vi "磨合台.vi"() -> ()   [LabVIEW 2020]
uses:
  <vilib>/Utility/config.llb/NI_LVConfig.lvlib
  <vilib>/Analysis/NI_AALBase.lvlib
  <vilib>/Analysis/baseanly.llb/Mean (DBL).vi
  Global_Variable/A131258.vi
  Global_Variable/Global.vi
  Database/Global1.vi
  <vilib>/addons/database/NI_Database_API.lvlib
  <vilib>/addons/database/Recordset.llb/Rec Fetch Recordset Data (R).vi
  <vilib>/addons/database/Connection.llb/DB Tools Open Connec (String).vi
  <vilib>/addons/database/Connection.llb/Conn Execute.vi
  <userlib>/_MGI/Menu Building/MenuItemStatusChange/MGI_MenuItemStatusChange.lvclass
  System.Windows.Forms
panel:
  in  "系数":bool
  out "右平均差":string
  out "左平均差":string
  out "右逆向空载":dbl
  out "左逆向空载":dbl
  in  "MenuStrip":refnum<k24>(container)
  in  "选项卡控件 2":enum32{"检测曲线", "参数查看"}(tab)
  out "平均值差下限":dbl format="%_4g"
  out "平均值差上限":dbl format="%_4g"
  out "右工位正逆平均扭矩差(Nm)":dbl format="%.3g"
  out "左工位正逆平均扭矩差(Nm)":dbl format="%.3g"
  out "最小值下限":dbl format="%_4g"
  out "力位移曲线 4":cluster{dbl[], dbl[]}[](graph)
  out "力位移曲线 3":cluster{dbl[], dbl[]}[](graph)
  out "不合格指示灯  2":bool
  out "合格指示灯 2":bool
  out "最大值上限":dbl format="%_4g"
  out "波动值下限":dbl format="%_4g"
  out "波动值上限":dbl format="%_4g"
  out "平均值下限":dbl format="%_4g"
  out "平均值上限":dbl format="%_4g"
  out "不合格指示灯":bool
  out "合格指示灯":bool
  out "最小值上限":dbl format="%_4g"
  out "最大值下限":dbl format="%_4g"
  out "左工位追溯码":string
  out "右工位追溯码":string
  out "左工位正向平均扭矩(Nm)":dbl format="%.3g"
  out "左工位正向波动扭矩(Nm)":dbl format="%.3g"
  out "左工位正向最大扭矩(Nm)":dbl format="%.3g"
  out "左工位正向最小扭矩(Nm)":dbl format="%.3g"
  out "右工位逆向平均扭矩(Nm)":dbl format="%.3g"
  out "右工位逆向波动扭矩(Nm)":dbl format="%.3g"
  out "右工位逆向最小扭矩(Nm)":dbl format="%.3g"
  out "右工位逆向最大扭矩(Nm)":dbl format="%.3g"
  out "左工位逆向最大扭矩(Nm)":dbl format="%.3g"
  out "左工位逆向最小扭矩(Nm)":dbl format="%.3g"
  out "左工位逆向波动扭矩(Nm)":dbl format="%.3g"
  out "左工位逆向平均扭矩(Nm)":dbl format="%.3g"
  out "右工位正向最小扭矩(Nm)":dbl format="%.3g"
  out "右工位正向最大扭矩(Nm)":dbl format="%.3g"
  out "右工位正向波动扭矩(Nm)":dbl format="%.3g"
  out "右工位正向平均扭矩(Nm)":dbl format="%.3g"
  in  "删除":bool
  in  "确定":bool
  in  "添加":bool
  in  "退出":bool
  in  "更新":bool
  in  "产品型号":string(combo)
  in  "选项卡控件 3":enum32{"工位参数", "产品管理", "用户管理"}(tab)
  in  "坐标轴参数":string[][](table)=[["mm"], ["mm/s"]]
  in  "判定框参数":string[][](table)=[["mm"], ["mm/s"]]
  in  "结果判定参数":string[][](table)=[["mm"], ["mm/s"]]
  in  "系数 2":string[][](table)=[["1"], ["1"], ["1"], ["1"], ["1"], ["0.75"]]
  in  "请输入添加的产品名称":string
  in  "请选择要删除的产品":string(combo)
  in  "确定按钮":bool
  out "左空载系数":dbl
  out "右空载系数":dbl
  out "右扭矩波动":dbl
  out "左扭矩波动":dbl
  out "右平均扭矩系数":dbl
  out "左平均扭矩系数":dbl
  out "系数":dbl
  out "字符串":string
  out "code 3":string
  out "code 2":string
  out "右正波结果":string
  out "右正平结果":string
  out "右正大结果":string
  out "右正小结果":string
  out "右逆波结果":string
  out "右逆平结果":string
  out "右逆大结果":string
  out "右逆小结果":string
  out "左正波结果":string
  out "左正平结果":string
  out "左正大结果":string
  out "左正小结果":string
  out "左逆波结果":string
  out "左逆平结果":string
  out "左逆大结果":string
  out "左逆小结果":string
  out "RIGHTRESULT":string
  out "LEFTRESULT":string
  out "RIGHTCODEID":string
  out "DEVICEID":string
  out "PRODUCTID":string
  out "USERID":string
  out "LEFTCODEID":string
  out "产品型号":string
  out "联机模式":string
  out "用户权限":string
  out "用户名":string
  in  "附加信息":string
  in  "设备状态":enum16{"设备离线", "设备正常", "设备缺料", "设备故障", "质量报警"}(ring)=enum."设备故障"
  in  "附加信息 2":string
  in  "设备状态 2":enum16{"设备离线", "设备正常", "设备缺料", "设备故障", "质量报警"}(ring)=enum."设备缺料"
  in  "附加信息 3":string
  in  "设备状态 3":enum16{"设备离线", "设备正常", "设备缺料", "设备故障", "质量报警"}(ring)=enum."质量报警"
  in  "质量报警":bool
  in  "设备缺料":bool
  in  "设备故障":bool
  in  "右工位判定结果 4":bool[][](array[boolean])=[[TRUE]]
  in  "右工位报表":string[][](table)=[["mm"], ["mm/s"]]
  in  "左工位判定结果 3":bool[][](array[boolean])=[[TRUE]]
  in  "左工位报表":string[][](table)=[["mm"], ["mm/s"]]
  in  "Initialize 4":bool
  in  "Initialize 2":bool
  in  "Initialize 5":bool
  in  "Initialize 3":bool
  # "020芯轴分总成磨合"
  # "左工位逆空载"
  # "右工位逆空载"
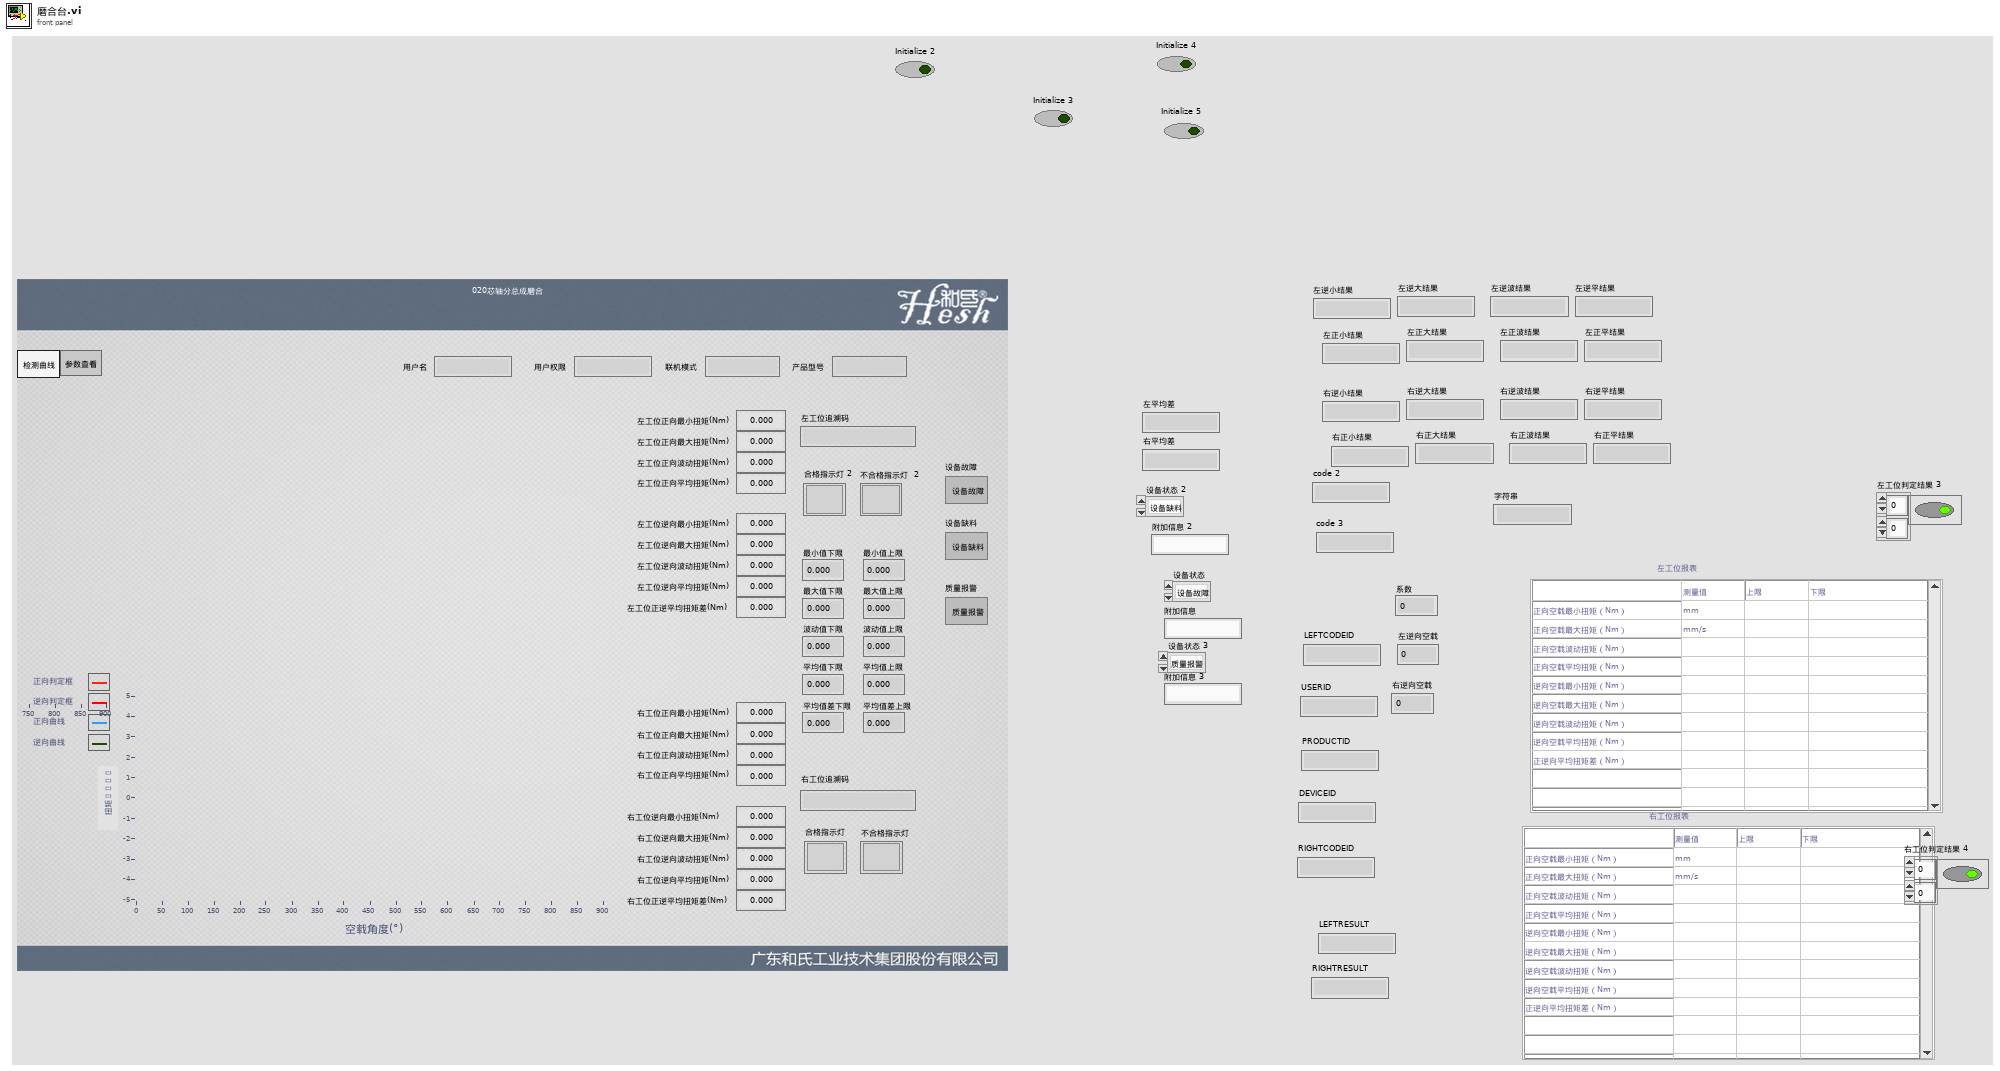
[diagram p1: front panel]
types:
  T1 = enum32{"Invalid", "Standard", "Closed", "Hidden", "Minimized", "Maximized"}
  T2 = cluster{"用户编号":string, "用户名":string, "用户密码(密文)":string, "用户权限":string}
  T3 = cluster{"设备名称":string, "用户名":string, "设备状态":enum16{"设备离线", "设备正常", "设备缺料", "设备故障", "质量报警"}, "附加信息":string}
  T4 = typedef "NI_LVConfig.lvlib/Config Data RefNum.ctl" = refnum<k1>
  T5 = cluster{i64, i64, string, "右工位正向波动扭矩(Nm)":dbl, "波动值下限":dbl, "波动值上限":dbl, string, "右正波结果  ":string}
  T6 = cluster{i64, i64, string, "右工位逆向最小扭矩(Nm)":dbl, "最小值下限":dbl, "最小值上限":dbl, string, "右逆小结果":string}
  T7 = cluster{i64, i64, string, "右工位逆向最大扭矩(Nm)":dbl, "最大值下限":dbl, "最大值上限":dbl, string, "右逆大结果 ":string}
  T8 = cluster{i64, i64, string, "右工位正向最大扭矩(Nm)":dbl, "最大值上限":dbl, "最大值下限":dbl, string, "右正大结果 ":string}
  T9 = cluster{i64, i64, string, "右工位逆向平均扭矩(Nm)":dbl, "平均值下限":dbl, "平均值上限":dbl, string, "右逆平结果 ":string}
  T10 = cluster{i64, i64, string, "右工位正向最小扭矩(Nm)":dbl, "最小值下限":dbl, "最小值上限":dbl, string, "右正小结果  ":string}
  T11 = cluster{i64, i64, string, "右工位正向平均扭矩(Nm)":dbl, "平均值下限":dbl, "平均值上限":dbl, string, "右正平结果  ":string}
  T12 = cluster{i64, i64, string, "右工位逆向波动扭矩(Nm)":dbl, "波动值下限":dbl, "波动值上限":dbl, string, "右逆波结果 ":string}
  T13 = cluster{i64, i64, string, "右工位正逆平均扭矩差(Nm)":dbl, "平均值差下限":dbl, "平均值差上限":dbl, string, "右平均差":string}
  T14 = cluster{i64, i64, string, "右工位正逆平均扭矩差(Nm)":dbl, "平均值差下限":dbl, "平均值差上限":dbl, string, "右平均差":string}[]
  T15 = typedef "NI_Database_API.lvlib/Conn ObjectReference.ctl" = refnum<k1>
  T16 = cluster{i64, i64, "右工位正逆平均扭矩差(Nm)":dbl, "平均值差下限":dbl, "平均值差上限":dbl, string, "右平均差":string}
  T17 = cluster{i64, i64, i64, "RIGHTRESULT":string, "result string":string}
  T18 = cluster{i64, i64, i64, "RIGHTRESULT":string, "result string":string}[]
  T19 = cluster{i64, i64, "RIGHTRESULT":string, "result string":string}
  T20 = cluster{i64, i64, string, "左工位逆向最小扭矩(Nm)":dbl, "最小值下限":dbl, "最小值上限":dbl, string, "左逆小结果":string}
  T21 = cluster{i64, i64, string, "左工位逆向最大扭矩(Nm)":dbl, "最大值下限":dbl, "最大值上限":dbl, string, "左逆大结果":string}
  T22 = cluster{i64, i64, string, "左工位逆向波动扭矩(Nm)":dbl, "波动值下限":dbl, "波动值上限":dbl, string, "左逆波结果":string}
  T23 = cluster{i64, i64, string, "左工位逆向平均扭矩(Nm)":dbl, "平均值下限":dbl, "平均值上限":dbl, string, "左逆平结果":string}
  T24 = cluster{i64, i64, string, "左工位正向最小扭矩(Nm)":dbl, "最小值下限":dbl, "最小值上限":dbl, string, "左正小结果 ":string}
  T25 = cluster{i64, i64, string, "左工位正向最大扭矩(Nm)":dbl, "最大值下限":dbl, "最大值上限":dbl, string, "左正大结果":string}
  T26 = cluster{i64, i64, string, "左工位正向波动扭矩(Nm)":dbl, "波动值下限":dbl, "波动值上限":dbl, string, "左正波结果 ":string}
  T27 = cluster{i64, i64, string, "左工位正向平均扭矩(Nm)":dbl, "平均值下限":dbl, "平均值上限":dbl, string, "左正平结果 ":string}
  T28 = cluster{i64, i64, string, "左工位正逆平均扭矩差(Nm)":dbl, "平均值差下限":dbl, "平均值差上限":dbl, string, "左正平结果 ":string}
  T29 = cluster{i64, i64, string, "左工位正逆平均扭矩差(Nm)":dbl, "平均值差下限":dbl, "平均值差上限":dbl, string, "左正平结果 ":string}[]
  T30 = cluster{i64, i64, "左工位正逆平均扭矩差(Nm)":dbl, "平均值差下限":dbl, "平均值差上限":dbl, string, "左正平结果 ":string}
  T31 = cluster{i64, i64, i64, "LEFTRESULT":string, "result string":string}
  T32 = cluster{i64, i64, i64, "LEFTRESULT":string, "result string":string}[]
  T33 = cluster{"LEFTRESULT":string, "result string":string}
  T34 = typedef "NI_Database_API.lvlib/Rec ObjectReference.ctl" = refnum<k1>
  T35 = cluster{"设备名称":string, "用户名":string, "设备状态 2":enum16{"设备离线", "设备正常", "设备缺料", "设备故障", "质量报警"}, "附加信息 2":string}
  T36 = cluster{"设备名称":string, "用户名":string, "设备状态 3":enum16{"设备离线", "设备正常", "设备缺料", "设备故障", "质量报警"}, "附加信息 3":string}
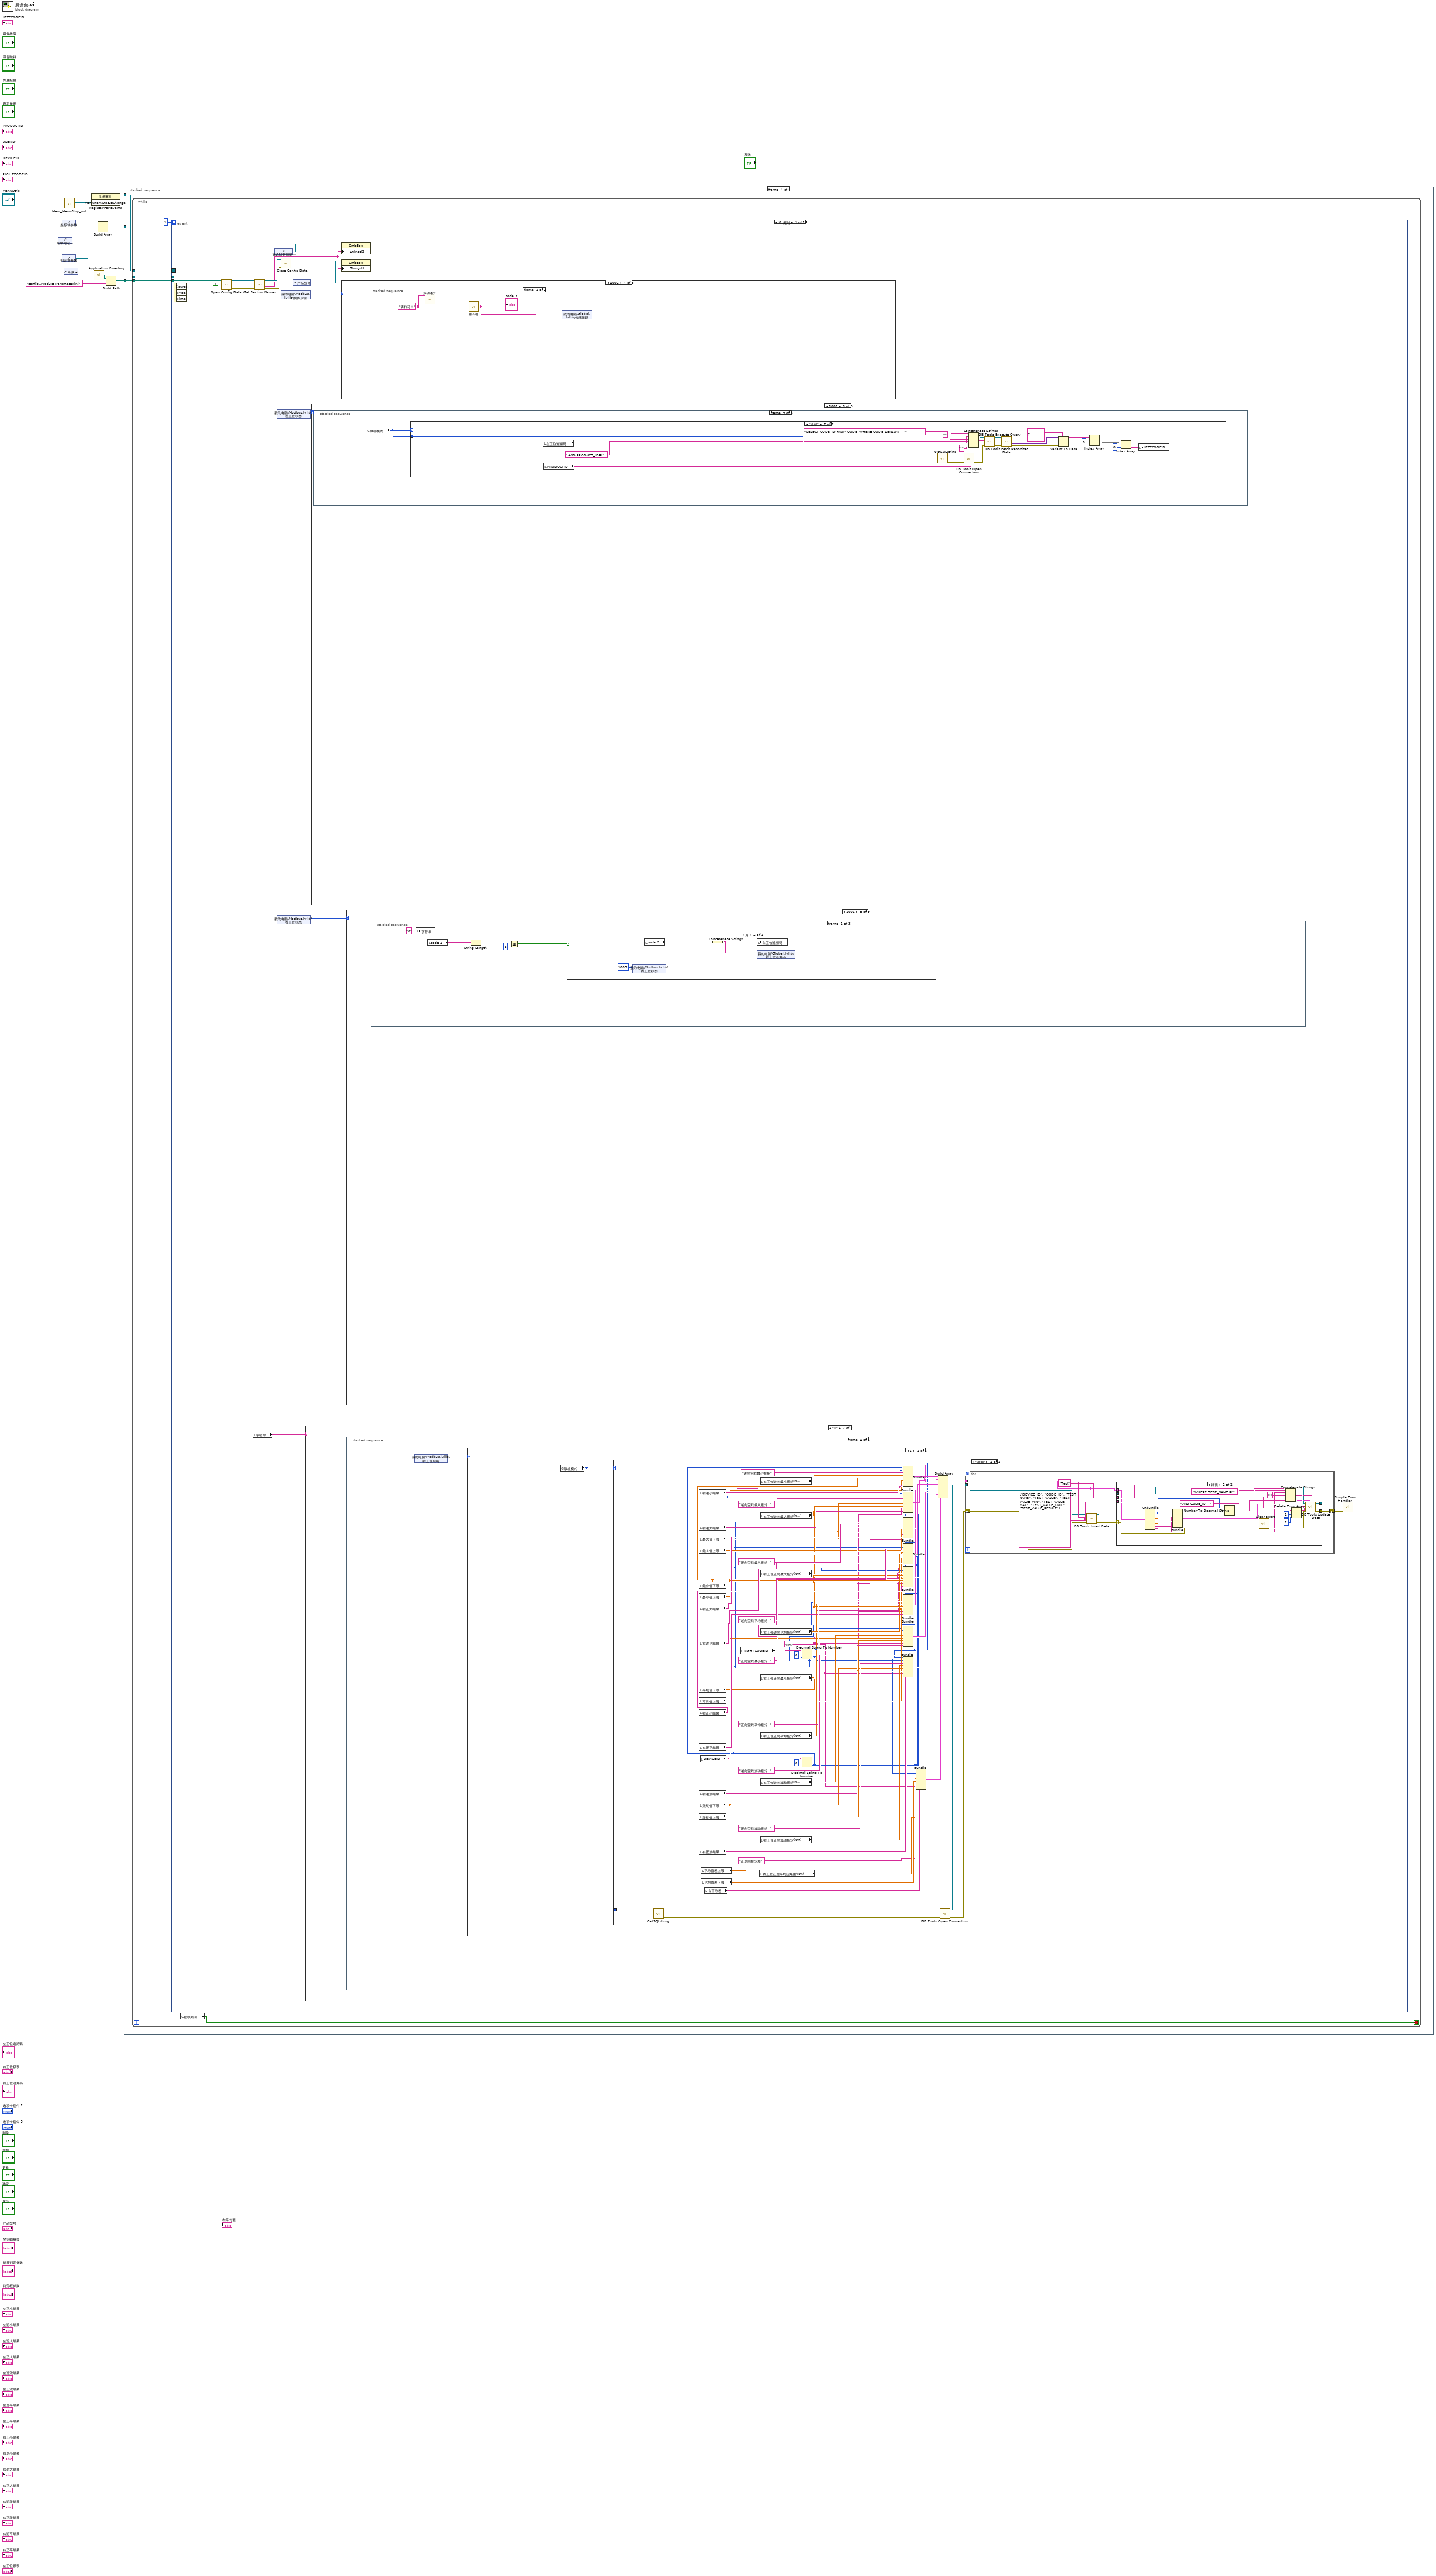
[diagram p0: block diagram]
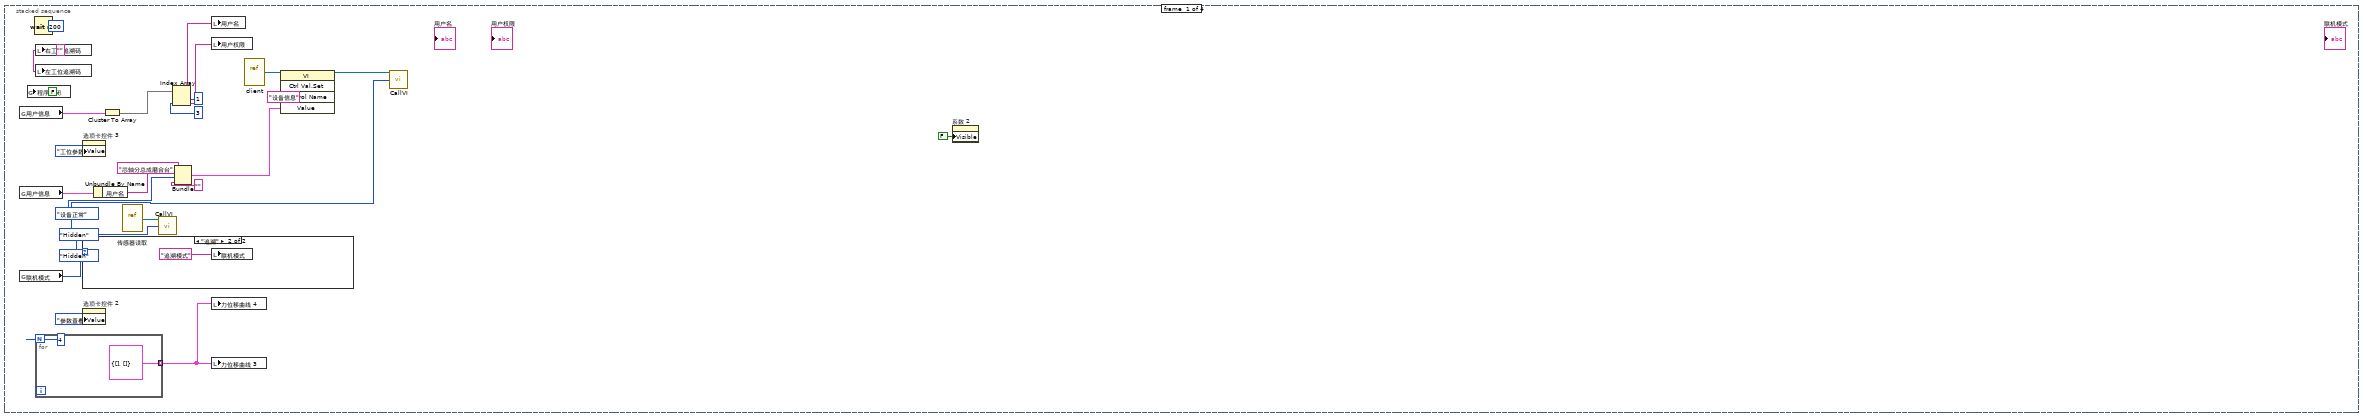
[diagram p2: hidden frame]
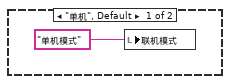
[diagram p3: hidden frame]
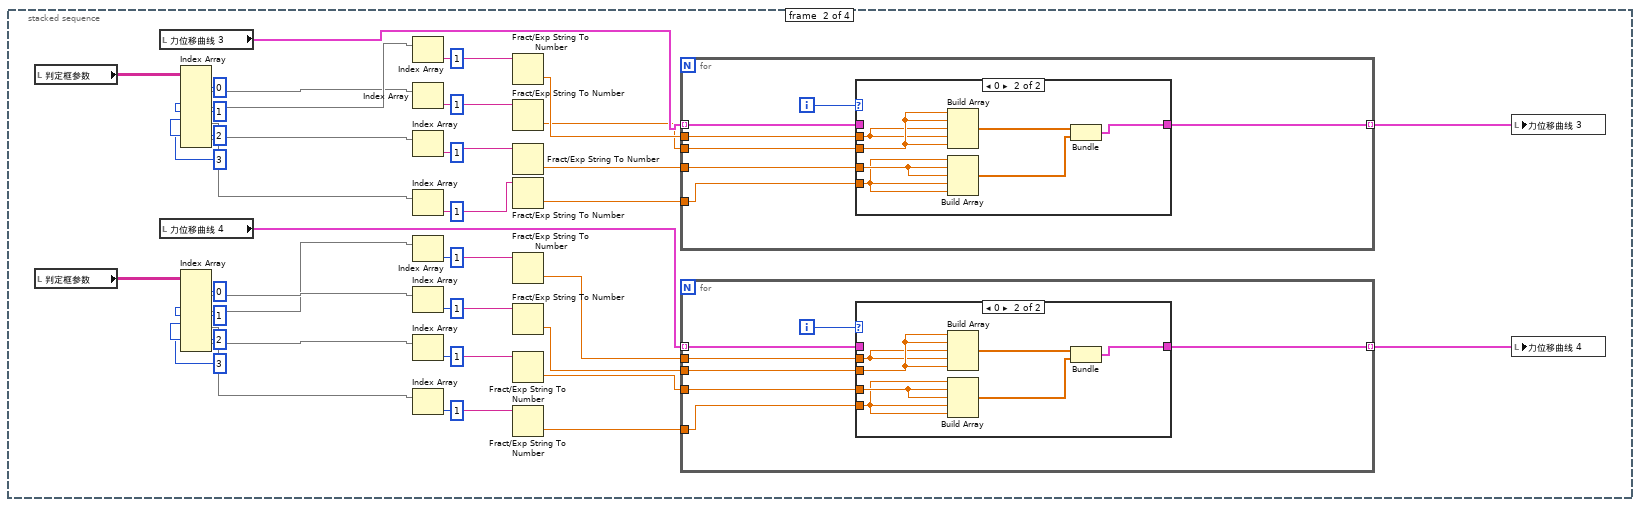
[diagram p4: hidden frame]
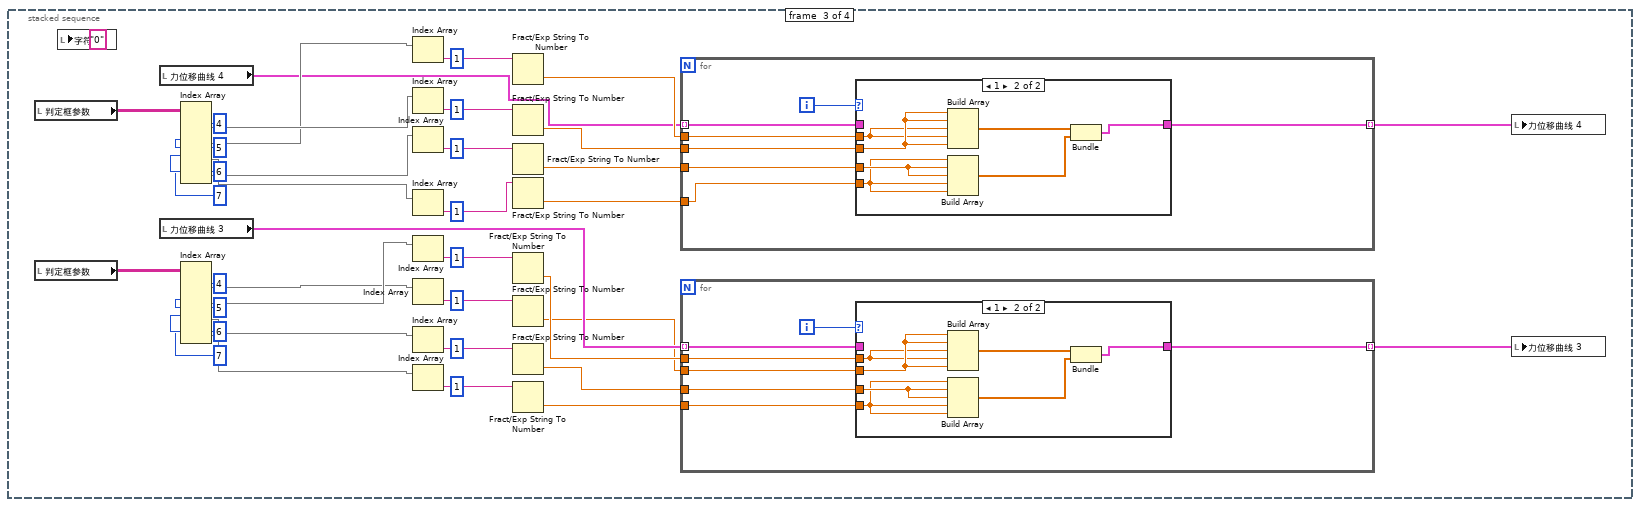
[diagram p7: hidden frame]
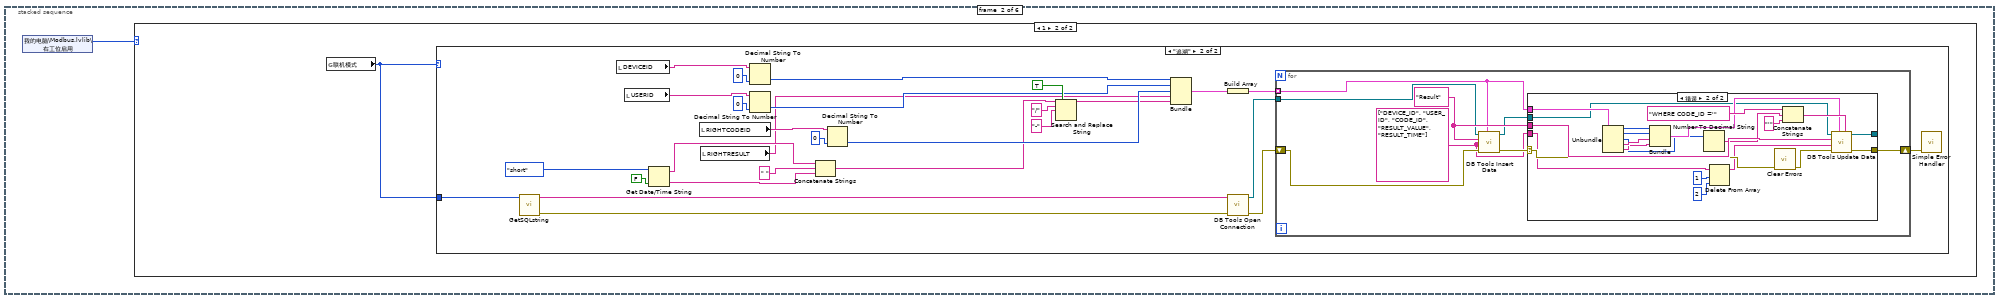
[diagram p14: hidden frame]
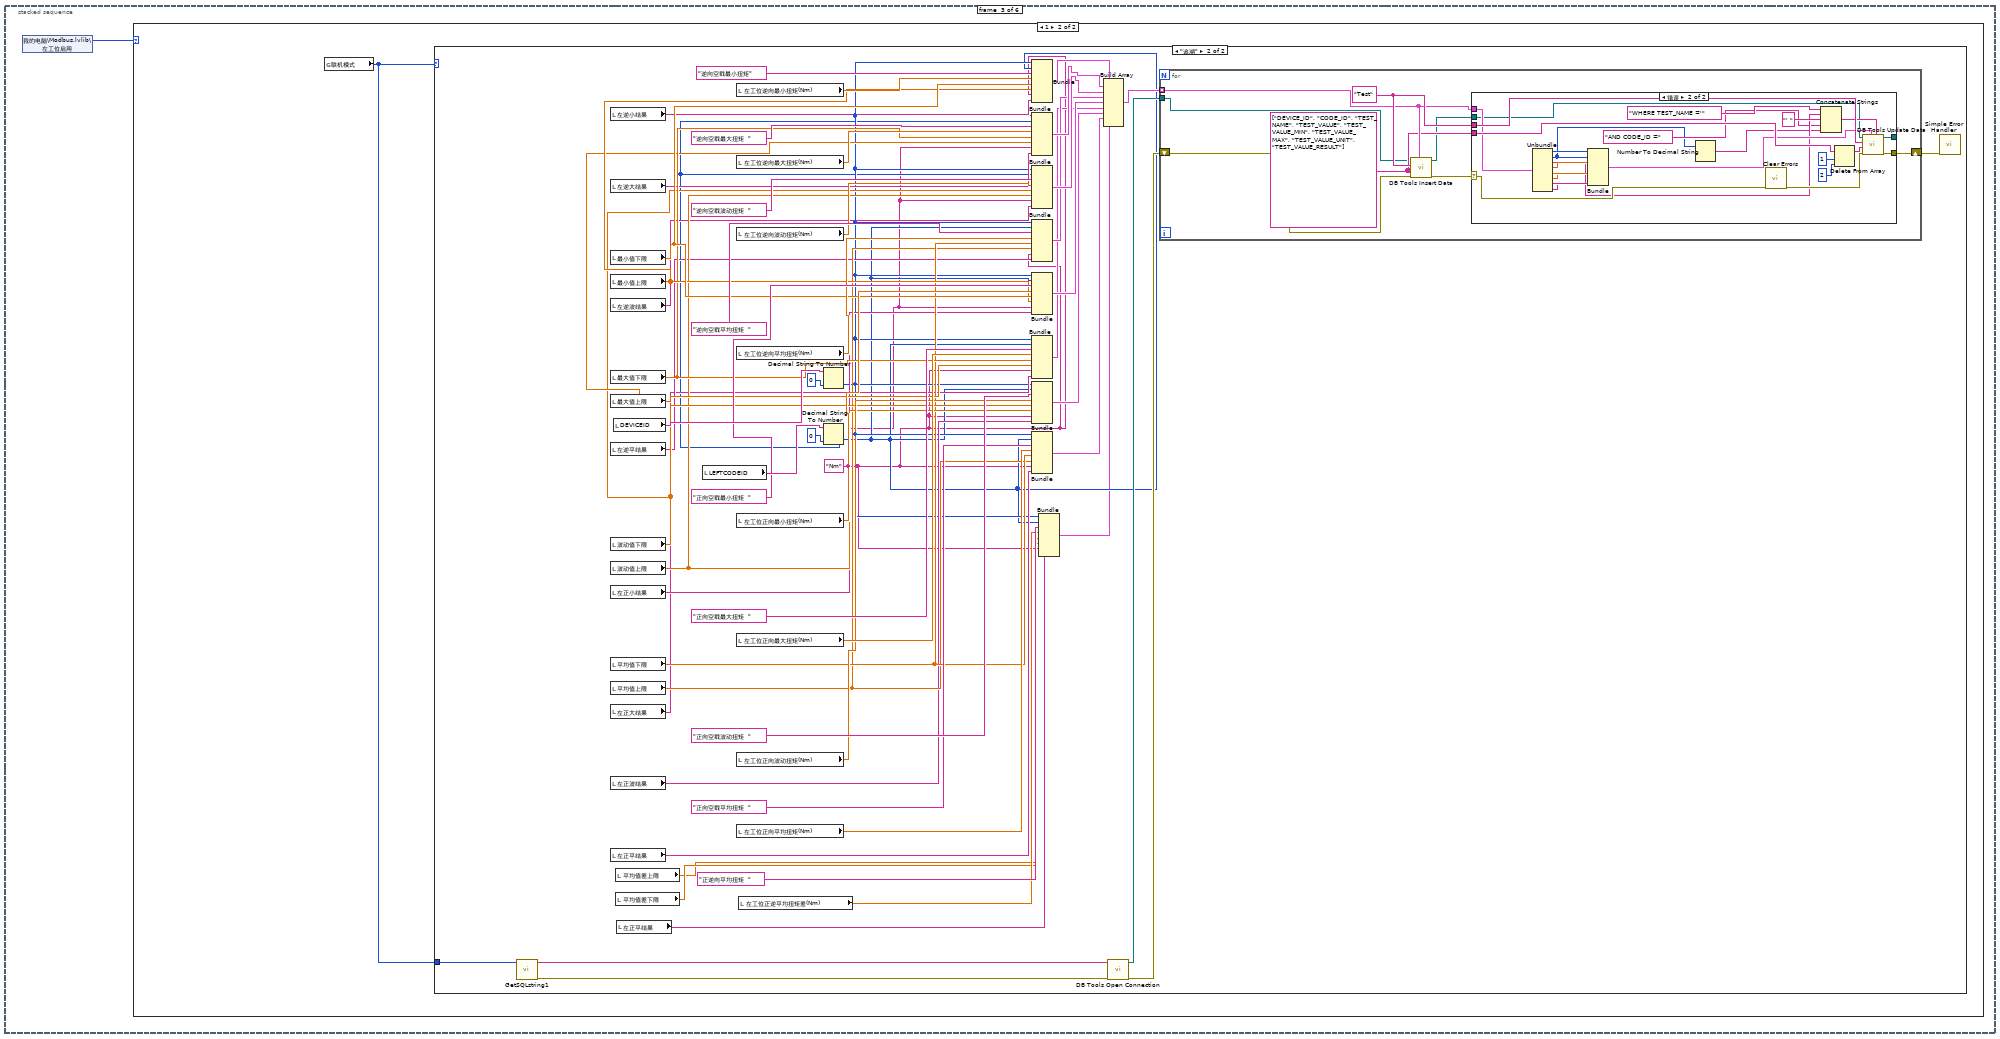
[diagram p18: hidden frame]
diagram:
  n1 = control-ref of="结果判定参数"() -> (w6:refnum<vi>)
  n2 = control-ref of="坐标轴参数"() -> (w7:refnum<vi>)
  n3 = control-ref of="判定框参数"() -> (w5:refnum<vi>)
  n4 = control-ref of="系数 2"() -> (w4:refnum<vi>)
  n5 = call "Main_MenuStrip_init.vi"("MenuStrip"="MenuStrip") -> ("MenuItemStatusChange"=w3:refnum<user-event>)  [unwired: 9 in, 1 out]
  n6 = register-events(w3) -> (reference out=w1:refnum<event-registration>)  [unwired: 2 in, 1 out]
  n7 = call <vilib>:"Application Directory.vi"() -> ("Application Directory"=w11:path)
  n8 = Build Array(w7, w6, w5, w4) -> (w8:refnum<vi>[])
  n9 = Build Path(base path=w11, name or relative path="config\\Product_Parameter.ini" ("名称或相对路径")) -> (appended path=w9:path)
  n10 = stacked-sequence {
    tunnel: w9 -> [_ _ _ w197]
    tunnel: w8 -> [_ _ _ w196]
    tunnel: w1 -> [_ _ _ w195]
    frame #0 {
      w28 = ""
      n11 = global read "Global1.vi" "用户信息"() -> (w36:T2)
      n12 = global read "Global1.vi" "用户信息"() -> (w21:T2)
      n13 = global read "Global1.vi" "联机模式"() -> (w30:enum16{"单机", "追溯"})
      n14 = global write "Global.vi" "程序关闭"(FALSE ("程序关闭")) -> ()
      n15 = Wait (ms)(milliseconds to wait=u32 200 ("等待时间（毫秒）")) -> ()  [unwired: 1 out]
      n16 = local write "右工位追溯码"(w28) -> ()
      n17 = local write "左工位追溯码"(w28) -> ()
      n18 = for {
        N: 4 -> [_]
        tunnel: [cluster{dbl[], dbl[]} {[], []}] -> w37 mode=indexing
      }
      n19 = property on="选项卡控件 3" class="TabCtl (严格)"("Value"=enum32{"工位参数", "产品管理", "用户管理"}."工位参数" ("选项卡控件 3")) -> ()  [unwired: 2 in, 2 out]
      n20 = case shown="\"追溯\"" w30 {
        frame "单机", Default {
          n21 = local write "联机模式"("单机模式" ("联机模式")) -> ()
        }
        frame "追溯" {
          n22 = local write "联机模式"("追溯模式" ("联机模式")) -> ()
        }
      }
      n23 = property on="选项卡控件 2" class="TabCtl (严格)"("Value"=enum32{"检测曲线", "参数查看"}."参数查看" ("选项卡控件 2")) -> ()  [unwired: 2 in, 2 out]
      n24 = Unbundle By Name(w21) -> ("用户名"=w20:string)
      n25 = Cluster To Array(cluster=w36) -> (array=w35:string[])
      n26 = vi-ref "传感器读取.vi"() -> (w27:refnum<vi>)
      n27 = call "CallVI.vi"("VI引用"=w27, "状态"=T1."Hidden") -> ()  [unwired: 11 in, 3 out]
      n28 = Index Array(array=w35, index #1=1 ("索引"), index #2=3 ("索引")) -> (element #1=w32:string, element #2=w31:string)
      n29 = Bundle("设备名称"="芯轴分总成磨合台", "用户名"=w20, "设备状态"=enum16{"设备离线", "设备正常", "设备缺料", "设备故障", "质量报警"}."设备正常", "附加信息"="") -> (w19:T3)  [unwired: 1 in]
      n30 = local write "用户名"(w32) -> ()
      n31 = local write "用户权限"(w31) -> ()
      n32 = local write "力位移曲线 4"(w37) -> ()
      n33 = local write "力位移曲线 3"(w37) -> ()
      n34 = vi-ref "client.vi"() -> (w18:refnum<vi>)
      n35 = invoke class="VI" method="Ctrl Val.Set"(reference=w18, "Control Name"="设备信息" ("控件名"), "Value"=w19) -> (reference out=w22:refnum<vi>)  [unwired: 2 in, 4 out]
      n36 = call "CallVI.vi"("VI引用"=w22, "状态"=T1."Hidden") -> ()  [unwired: 11 in, 3 out]
      n37 = property on="系数 2" class="Tbl (严格)"("Visible"=FALSE ("可见")) -> ()  [unwired: 2 in, 2 out]
    }
    frame #1 {
      n38 = local read "判定框参数"() -> (w64:string[][])
      n39 = local read "判定框参数"() -> (w65:string[][])
      n40 = local read "力位移曲线 3"() -> (w63:cluster{dbl[], dbl[]}[])
      n41 = local read "力位移曲线 4"() -> (w66:cluster{dbl[], dbl[]}[])
      n42 = Index Array(array=w64, index (row) #1=0 ("索引 (行)"), index (row) #2=1 ("索引 (行)"), index (row) #3=2 ("索引 (行)"), index (row) #4=3 ("索引 (行)")) -> (element #1=w50:string[], element #2=w51:string[], element #3=w52:string[], element #4=w53:string[])  [unwired: 4 in]
      n43 = Index Array(array=w65, index (row) #1=0 ("索引 (行)"), index (row) #2=1 ("索引 (行)"), index (row) #3=2 ("索引 (行)"), index (row) #4=3 ("索引 (行)")) -> (element #1=w83:string[], element #2=w78:string[], element #3=w77:string[], element #4=w76:string[])  [unwired: 4 in]
      n44 = Index Array(array=w51, index=1 ("索引")) -> (element=w59:string)
      n45 = Index Array(array=w50, index=1 ("索引")) -> (element=w58:string)
      n46 = Index Array(array=w53, index=1 ("索引")) -> (element=w61:string)
      n47 = Index Array(array=w52, index=1 ("索引")) -> (element=w60:string)
      n48 = Index Array(array=w78, index=1 ("索引")) -> (element=w70:string)
      n49 = Index Array(array=w83, index=1 ("索引")) -> (element=w71:string)
      n50 = Index Array(array=w76, index=1 ("索引")) -> (element=w68:string)
      n51 = Index Array(array=w77, index=1 ("索引")) -> (element=w69:string)
      n52 = Fract/Exp String To Number(string=w59) -> (number=w55:dbl)  [unwired: 3 in, 1 out]
      n53 = Fract/Exp String To Number(string=w58) -> (number=w54:dbl)  [unwired: 3 in, 1 out]
      n54 = Fract/Exp String To Number(string=w61) -> (number=w56:dbl)  [unwired: 3 in, 1 out]
      n55 = Fract/Exp String To Number(string=w60) -> (number=w57:dbl)  [unwired: 3 in, 1 out]
      n56 = Fract/Exp String To Number(string=w70) -> (number=w74:dbl)  [unwired: 3 in, 1 out]
      n57 = Fract/Exp String To Number(string=w71) -> (number=w75:dbl)  [unwired: 3 in, 1 out]
      n58 = Fract/Exp String To Number(string=w68) -> (number=w73:dbl)  [unwired: 3 in, 1 out]
      n59 = Fract/Exp String To Number(string=w69) -> (number=w72:dbl)  [unwired: 3 in, 1 out]
      n60 = for {
        tunnel: [w94] -> w62 mode=indexing
        tunnel: w63 -> [w93] mode=indexing
        tunnel: w54 -> [w91]
        tunnel: w55 -> [w90]
        tunnel: w56 -> [w89]
        tunnel: w57 -> [w88]
        i -> [w92]
        n61 = case shown="0" w92 {
          tunnel: [w95 w100] -> w94
          tunnel: w93 -> [w95 _]
          tunnel: w91 -> [_ w99]
          tunnel: w90 -> [_ w98]
          tunnel: w89 -> [_ w97]
          tunnel: w88 -> [_ w96]
          frame Default {
          }
          frame 0 {
            n62 = Build Array(w99, w99, w98, w98, w99) -> (w101:dbl[])
            n63 = Build Array(w96, w97, w97, w96, w96) -> (w102:dbl[])
            n64 = Bundle(w101, w102) -> (w100:cluster{dbl[], dbl[]})  [unwired: 1 in]
          }
        }
      }
      n65 = for {
        tunnel: [w109] -> w67 mode=indexing
        tunnel: w66 -> [w108] mode=indexing
        tunnel: w75 -> [w106]
        tunnel: w74 -> [w105]
        tunnel: w73 -> [w104]
        tunnel: w72 -> [w103]
        i -> [w107]
        n66 = case shown="0" w107 {
          tunnel: [w110 w115] -> w109
          tunnel: w108 -> [w110 _]
          tunnel: w106 -> [_ w114]
          tunnel: w105 -> [_ w113]
          tunnel: w104 -> [_ w112]
          tunnel: w103 -> [_ w111]
          frame Default {
          }
          frame 0 {
            n67 = Build Array(w114, w114, w113, w113, w114) -> (w116:dbl[])
            n68 = Build Array(w111, w112, w112, w111, w111) -> (w117:dbl[])
            n69 = Bundle(w116, w117) -> (w115:cluster{dbl[], dbl[]})  [unwired: 1 in]
          }
        }
      }
      n70 = local write "力位移曲线 3"(w62) -> ()
      n71 = local write "力位移曲线 4"(w67) -> ()
    }
    frame #2 {
      n72 = local read "判定框参数"() -> (w129:string[][])
      n73 = local read "判定框参数"() -> (w162:string[][])
      n74 = local write "字符串"("0" ("字符串")) -> ()
      n75 = local read "力位移曲线 4"() -> (w128:cluster{dbl[], dbl[]}[])
      n76 = local read "力位移曲线 3"() -> (w163:cluster{dbl[], dbl[]}[])
      n77 = Index Array(array=w129, index (row) #1=4 ("索引 (行)"), index (row) #2=5 ("索引 (行)"), index (row) #3=6 ("索引 (行)"), index (row) #4=7 ("索引 (行)")) -> (element #1=w141:string[], element #2=w140:string[], element #3=w139:string[], element #4=w138:string[])  [unwired: 4 in]
      n78 = Index Array(array=w162, index (row) #1=4 ("索引 (行)"), index (row) #2=5 ("索引 (行)"), index (row) #3=6 ("索引 (行)"), index (row) #4=7 ("索引 (行)")) -> (element #1=w150:string[], element #2=w151:string[], element #3=w152:string[], element #4=w153:string[])  [unwired: 4 in]
      n79 = Index Array(array=w140, index=1 ("索引")) -> (element=w132:string)
      n80 = Index Array(array=w141, index=1 ("索引")) -> (element=w133:string)
      n81 = Index Array(array=w138, index=1 ("索引")) -> (element=w130:string)
      n82 = Index Array(array=w139, index=1 ("索引")) -> (element=w131:string)
      n83 = Index Array(array=w151, index=1 ("索引")) -> (element=w159:string)
      n84 = Index Array(array=w150, index=1 ("索引")) -> (element=w158:string)
      n85 = Index Array(array=w153, index=1 ("索引")) -> (element=w161:string)
      n86 = Index Array(array=w152, index=1 ("索引")) -> (element=w160:string)
      n87 = Fract/Exp String To Number(string=w132) -> (number=w136:dbl)  [unwired: 3 in, 1 out]
      n88 = Fract/Exp String To Number(string=w133) -> (number=w137:dbl)  [unwired: 3 in, 1 out]
      n89 = Fract/Exp String To Number(string=w130) -> (number=w135:dbl)  [unwired: 3 in, 1 out]
      n90 = Fract/Exp String To Number(string=w131) -> (number=w134:dbl)  [unwired: 3 in, 1 out]
      n91 = Fract/Exp String To Number(string=w159) -> (number=w155:dbl)  [unwired: 3 in, 1 out]
      n92 = Fract/Exp String To Number(string=w158) -> (number=w154:dbl)  [unwired: 3 in, 1 out]
      n93 = Fract/Exp String To Number(string=w161) -> (number=w156:dbl)  [unwired: 3 in, 1 out]
      n94 = Fract/Exp String To Number(string=w160) -> (number=w157:dbl)  [unwired: 3 in, 1 out]
      n95 = for {
        tunnel: [w171] -> w127 mode=indexing
        tunnel: w128 -> [w170] mode=indexing
        tunnel: w137 -> [w168]
        tunnel: w136 -> [w167]
        tunnel: w135 -> [w166]
        tunnel: w134 -> [w165]
        i -> [w169]
        n96 = case shown="1" w169 {
          tunnel: [w172 w177] -> w171
          tunnel: w170 -> [w172 _]
          tunnel: w168 -> [_ w176]
          tunnel: w167 -> [_ w175]
          tunnel: w166 -> [_ w174]
          tunnel: w165 -> [_ w173]
          frame Default {
          }
          frame 1 {
            n97 = Build Array(w176, w176, w175, w175, w176) -> (w178:dbl[])
            n98 = Build Array(w173, w174, w174, w173, w173) -> (w179:dbl[])
            n99 = Bundle(w178, w179) -> (w177:cluster{dbl[], dbl[]})  [unwired: 1 in]
          }
        }
      }
      n100 = for {
        tunnel: [w186] -> w164 mode=indexing
        tunnel: w163 -> [w185] mode=indexing
        tunnel: w154 -> [w183]
        tunnel: w155 -> [w182]
        tunnel: w156 -> [w181]
        tunnel: w157 -> [w180]
        i -> [w184]
        n101 = case shown="1" w184 {
          tunnel: [w187 w192] -> w186
          tunnel: w185 -> [w187 _]
          tunnel: w183 -> [_ w191]
          tunnel: w182 -> [_ w190]
          tunnel: w181 -> [_ w189]
          tunnel: w180 -> [_ w188]
          frame Default {
          }
          frame 1 {
            n102 = Build Array(w191, w191, w190, w190, w191) -> (w193:dbl[])
            n103 = Build Array(w188, w189, w189, w188, w188) -> (w194:dbl[])
            n104 = Bundle(w193, w194) -> (w192:cluster{dbl[], dbl[]})  [unwired: 1 in]
          }
        }
      }
      n105 = local write "力位移曲线 4"(w127) -> ()
      n106 = local write "力位移曲线 3"(w164) -> ()
    }
    frame #3 {
      n107 = while {
        tunnel: w197 -> [w201]
        tunnel: w196 -> [w200]
        tunnel: w195 -> [w198]
        stop <- w199 stop-if-true
        n108 = event shown="[0] 超时" {
          selector: w198 -> [_ _ _ _ _ _ _ _ _ _ _ _ _ _ _ _]
          dyn-events: _ -> [_ _ _ _ _ _ _ _ _ _ _ _ _ _ _ _]
          timeout: 1 -> [_ _ _ _ _ _ _ _ _ _ _ _ _ _ _ _]
          tunnel: w201 -> [w207 _ w1677 _ _ _ w2017 w2036 _ w2047 _ _ _ _ _ _]
          tunnel: w200 -> [_ _ _ _ _ _ w2016 w2035 _ w2046 _ _ _ _ _ _]
          event Timeout {
            n109 = event-data() -> ()  [unwired: 1 in, 3 out]
            n110 = call <vilib>:"Open Config Data.vi"("create file if necessary (T)"=TRUE, "configuration file path"=w207) -> ("error out"=w212:errorcluster, "refnum"=w211:T4)  [unwired: 7 in, 1 out]
            n111 = local read "字符串"() -> (w204:string)
            n112 = call <vilib>:"Get Section Names.vi"("error in (no error)"=w212, "refnum"=w211) -> ("error out"=w214:errorcluster, "section names"=w210:string[], "refnum out"=w213:T4)  [unwired: 7 in]
            n113 = control-ref of="请选择要删除的产品"() -> (w208:refnum<vi>)
            n114 = shared-variable "我的电脑\\Modbus.lvlib\\左工位状态"() -> (w206:u16)  [unwired: 1 in, 1 out]
            n115 = shared-variable "我的电脑\\Modbus.lvlib\\右工位状态"() -> (w205:u16)  [unwired: 1 in, 1 out]
            n116 = call <vilib>:"Close Config Data.vi"("error in (no error)"=w214, "refnum"=w213) -> ()  [unwired: 8 in, 2 out]
            n117 = shared-variable "我的电脑\\Modbus.lvlib\\跳转步骤"() -> (w203:u16)  [unwired: 1 in, 1 out]
            n118 = control-ref of="产品型号"() -> (w209:refnum<vi>)
            n119 = case shown="\"1\"" w204 {
              frame "假", Default {
              }
              frame "1" {
                n120 = stacked-sequence {
                  frame #0 {
                    n121 = shared-variable "我的电脑\\Modbus.lvlib\\右工位启用"() -> (w216:u16)  [unwired: 1 in, 1 out]
                    n122 = case shown="1" w216 {
                      frame 0, Default {
                      }
                      frame 1 {
                        n123 = global read "Global1.vi" "联机模式"() -> (w217:enum16{"单机", "追溯"})
                        n124 = case shown="\"追溯\"" w217 {
                          tunnel: w217 -> [_ w276]
                          frame "单机", Default {
                          }
                          frame "追溯" {
                            w220 = "Nm"
                            n125 = call "GetSQLstring.vi"("联机模式"=w276) -> ("错误输出"=w274:errorcluster, "连接字符串"=w275:string)  [unwired: 9 in]
                            n126 = local read "右逆小结果"() -> (w258:string)
                            n127 = local read "右逆大结果"() -> (w257:string)
                            n128 = local read "最大值下限"() -> (w238:dbl)
                            n129 = local read "最大值上限"() -> (w239:dbl)
                            n130 = local read "最小值下限"() -> (w241:dbl)
                            n131 = local read "最小值上限"() -> (w240:dbl)
                            n132 = local read "右正大结果"() -> (w253:string)
                            n133 = local read "右逆平结果"() -> (w255:string)
                            n134 = local read "平均值下限"() -> (w235:dbl)
                            n135 = local read "平均值上限"() -> (w234:dbl)
                            n136 = local read "右正小结果"() -> (w254:string)
                            n137 = local read "右正平结果"() -> (w251:string)
                            n138 = local read "右逆波结果"() -> (w256:string)
                            n139 = local read "波动值下限"() -> (w237:dbl)
                            n140 = local read "波动值上限"() -> (w236:dbl)
                            n141 = local read "右正波结果"() -> (w252:string)
                            n142 = local read "DEVICEID"() -> (w269:string)
                            n143 = local read "平均值差上限"() -> (w221:dbl)
                            n144 = local read "平均值差下限"() -> (w224:dbl)
                            n145 = local read "右平均差"() -> (w219:string)
                            n146 = local read "RIGHTCODEID"() -> (w267:string)
                            n147 = local read "右工位正逆平均扭矩差(Nm)"() -> (w223:dbl)
                            n148 = local read "右工位逆向最小扭矩(Nm)"() -> (w250:dbl)
                            n149 = local read "右工位逆向最大扭矩(Nm)"() -> (w249:dbl)
                            n150 = local read "右工位正向最大扭矩(Nm)"() -> (w244:dbl)
                            n151 = local read "右工位逆向平均扭矩(Nm)"() -> (w246:dbl)
                            n152 = local read "右工位正向最小扭矩(Nm)"() -> (w245:dbl)
                            n153 = local read "右工位正向平均扭矩(Nm)"() -> (w242:dbl)
                            n154 = local read "右工位逆向波动扭矩(Nm)"() -> (w247:dbl)
                            n155 = local read "右工位正向波动扭矩(Nm)"() -> (w243:dbl)
                            n156 = Decimal String To Number(string=w267, default (0L)=i64 0 ("默认(0 I32)")) -> (number=w225:i64)  [unwired: 1 in, 1 out]
                            n157 = Decimal String To Number(string=w269, default (0L)=i64 0 ("默认(0 I32)")) -> (number=w226:i64)  [unwired: 1 in, 1 out]
                            n158 = Bundle(w226, w225, "正向空载波动扭矩  ", "右工位正向波动扭矩(Nm)"=w243, "波动值下限"=w237, "波动值上限"=w236, w220, "右正波结果"=w252) -> (w228:T5)  [unwired: 1 in]
                            n159 = Bundle(w226, w225, "逆向空载最小扭矩", "右工位逆向最小扭矩(Nm)"=w250, "最小值下限"=w241, "最小值上限"=w240, w220, "右逆小结果"=w258) -> (w271:T6)  [unwired: 1 in]
                            n160 = Bundle(w226, w225, "逆向空载最大扭矩  ", "右工位逆向最大扭矩(Nm)"=w249, "最大值下限"=w238, "最大值上限"=w239, w220, "右逆大结果"=w257) -> (w248:T7)  [unwired: 1 in]
                            n161 = Bundle(w226, w225, "正向空载最大扭矩  ", "右工位正向最大扭矩(Nm)"=w244, "最大值上限"=w239, "最大值下限"=w238, w220, "右正大结果"=w253) -> (w233:T8)  [unwired: 1 in]
                            n162 = Bundle(w226, w225, "逆向空载平均扭矩  ", "右工位逆向平均扭矩(Nm)"=w246, "平均值下限"=w235, "平均值上限"=w234, w220, "右逆平结果"=w255) -> (w232:T9)  [unwired: 1 in]
                            n163 = Bundle(w226, w225, "正向空载最小扭矩  ", "右工位正向最小扭矩(Nm)"=w245, "最小值下限"=w241, "最小值上限"=w240, w220, "右正小结果"=w254) -> (w231:T10)  [unwired: 1 in]
                            n164 = Bundle(w226, w225, "正向空载平均扭矩  ", "右工位正向平均扭矩(Nm)"=w242, "平均值下限"=w235, "平均值上限"=w234, w220, "右正平结果"=w251) -> (w230:T11)  [unwired: 1 in]
                            n165 = Bundle(w226, w225, "逆向空载波动扭矩  ", "右工位逆向波动扭矩(Nm)"=w247, "波动值下限"=w237, "波动值上限"=w236, w220, "右逆波结果"=w256) -> (w229:T12)  [unwired: 1 in]
                            n166 = Bundle(w226, w225, "正逆向扭矩差", "右工位正逆平均扭矩差(Nm)"=w223, "平均值差下限"=w224, "平均值差上限"=w221, w220, "右平均差"=w219) -> (w218:T13)  [unwired: 1 in]
                            n167 = Build Array(w271, w248, w233, w232, w231, w230, w229, w228, w218) -> (w270:T14)
                            n168 = call-poly <vilib>:"DB Tools Open Connection.vi"("error in (no error)"=w274, "connection information"=w275) -> ("error out"=w277:errorcluster, "connection reference"=w273:T15)  [unwired: 6 in]
                            n169 = for {
                              tunnel: w270 -> [w282] mode=indexing
                              tunnel: w273 -> [w280]
                              shift-right: [w278] -> w272
                              shift-left: w277 -> [w285]
                              w281 = string[] ["DEVICE_ID", "CODE_ID", "TEST_NAME", "TEST_VALUE", "TEST_VALUE_MIN", "TEST_VALUE_MAX", "TEST_VALUE_UNIT", "TEST_VALUE_RESULT"] ("columns")
                              w283 = "Test" ("table")
                              n170 = call <vilib>:"DB Tools Insert Data.vi"("data"=w282, "error in (no error)"=w285, "columns"=w281, "table"=w283, "connection reference"=w280) -> ("error out"=w284:errorcluster, "connection reference out"=w279:T15)  [unwired: 5 in]
                              n171 = case shown="错误" w284 {
                                selector: w284 -> [w286 w311]
                                tunnel: w281 -> [_ w308]
                                tunnel: w279 -> [w287 w293]
                                tunnel: w283 -> [_ w312]
                                tunnel: w282 -> [_ w302]
                                tunnel: [w287 w292] -> _
                                tunnel: [w286 w291] -> w278
                                frame No Error {
                                }
                                frame Error {
                                n172 = Unbundle(w302) -> (w301:i64, w289:i64, w294:string, "右工位正逆平均扭矩差(Nm)"=w300:dbl, "平均值差下限"=w299:dbl, "平均值差上限"=w298:dbl, w297:string, "右平均差"=w296:string)
                                n173 = Bundle(w301, w289, "右工位正逆平均扭矩差(Nm)"=w300, "平均值差下限"=w299, "平均值差上限"=w298, w297, "右平均差"=w296) -> (w295:T16)  [unwired: 1 in]
                                n174 = Number To Decimal String(number=w289) -> (decimal integer string=w288:string)  [unwired: 1 in]
                                n175 = call <vilib>:"Clear Errors.vi"("error in (no error)"=w311) -> ("error out"=w310:errorcluster)  [unwired: 5 in, 1 out]
                                n176 = Concatenate Strings("WHERE TEST_NAME ='" ("condition"), w294, "'", "AND CODE_ID =" ("condition"), w288) -> (w304:string)
                                n177 = Delete From Array(array=w308, length=1 ("长度"), index=2 ("索引")) -> (array with subset deleted=w309:string[])  [unwired: 1 out]
                                n178 = call <vilib>:"DB Tools Update Data.vi"("condition"=w304, "data"=w295, "error in (no error)"=w310, "columns"=w309, "table"=w312, "connection reference"=w293) -> ("error out"=w291:errorcluster, "connection reference out"=w292:T15)  [unwired: 4 in]
                                }
                              }
                            }
                            n179 = call <vilib>:"Simple Error Handler.vi"("error in (no error)"=w272) -> ()  [unwired: 4 in, 5 out]
                          }
                        }
                      }
                    }
                  }
                  frame #1 {
                    n180 = shared-variable "我的电脑\\Modbus.lvlib\\右工位启用"() -> (w313:u16)  [unwired: 1 in, 1 out]
                    n181 = case shown="1" w313 {
                      frame 0, Default {
                      }
                      frame 1 {
                        n182 = global read "Global1.vi" "联机模式"() -> (w314:enum16{"单机", "追溯"})
                        n183 = case shown="\"追溯\"" w314 {
                          tunnel: w314 -> [_ w341]
                          frame "单机", Default {
                          }
                          frame "追溯" {
                            n184 = call "GetSQLstring.vi"("联机模式"=w341) -> ("错误输出"=w339:errorcluster, "连接字符串"=w340:string)  [unwired: 9 in]
                            n185 = local read "DEVICEID"() -> (w334:string)
                            n186 = local read "USERID"() -> (w316:string)
                            n187 = Get Date/Time String(date format (0)=enum16{"short", "long", "abbreviated"}."short" ("日期格式(0)"), want seconds? (F)=FALSE ("需要秒？(F)")) -> (date string=w326:string, time string=w325:string)  [unwired: 1 in]
                            n188 = local read "RIGHTCODEID"() -> (w331:string)
                            n189 = local read "RIGHTRESULT"() -> (w315:string)
                            n190 = Decimal String To Number(string=w334, default (0L)=i64 0 ("默认(0 I32)")) -> (number=w332:i64)  [unwired: 1 in, 1 out]
                            n191 = Decimal String To Number(string=w316, default (0L)=i64 0 ("默认(0 I32)")) -> (number=w317:i64)  [unwired: 1 in, 1 out]
                            n192 = Concatenate Strings(w326, " " ("字符串"), w325) -> (w322:string)
                            n193 = Decimal String To Number(string=w331, default (0L)=i64 0 ("默认(0 I32)")) -> (number=w329:i64)  [unwired: 1 in, 1 out]
                            n194 = Search and Replace String(replace all?=TRUE ("替换全部？(F)"), input string=w322, search string="/" ("替换字符串(\"\")"), replace string="-" ("替换字符串(\"\")")) -> (result string=w323:string)  [unwired: 4 in, 3 out]
                            n195 = Bundle(w332, w317, w329, "RIGHTRESULT"=w315, "result string"=w323) -> (w336:T17)  [unwired: 1 in]
                            n196 = Build Array(w336) -> (w335:T18)
                            n197 = call-poly <vilib>:"DB Tools Open Connection.vi"("error in (no error)"=w339, "connection information"=w340) -> ("error out"=w342:errorcluster, "connection reference"=w338:T15)  [unwired: 6 in]
                            n198 = for {
                              tunnel: w335 -> [w347] mode=indexing
                              tunnel: w338 -> [w345]
                              shift-right: [w343] -> w337
                              shift-left: w342 -> [w350]
                              w346 = string[] ["DEVICE_ID", "USER_ID", "CODE_ID", "RESULT_VALUE", "RESULT_TIME"] ("columns")
                              w348 = "Result" ("table")
                              n199 = call <vilib>:"DB Tools Insert Data.vi"("data"=w347, "error in (no error)"=w350, "columns"=w346, "table"=w348, "connection reference"=w345) -> ("error out"=w349:errorcluster, "connection reference out"=w344:T15)  [unwired: 5 in]
                              n200 = case shown="错误" w349 {
                                selector: w349 -> [w351 w372]
                                tunnel: w346 -> [_ w369]
                                tunnel: w344 -> [w352 w357]
                                tunnel: w348 -> [_ w373]
                                tunnel: w347 -> [_ w363]
                                tunnel: [w352 w356] -> _
                                tunnel: [w351 w355] -> w343
                                frame No Error {
                                }
                                frame Error {
                                n201 = Unbundle(w363) -> (w362:i64, w361:i64, w353:i64, "RIGHTRESULT"=w360:string, "result string"=w359:string)
                                n202 = Bundle(w362, w361, "RIGHTRESULT"=w360, "result string"=w359) -> (w358:T19)  [unwired: 1 in]
                                n203 = Number To Decimal String(number=w353) -> (decimal integer string=w354:string)  [unwired: 1 in]
                                n204 = Delete From Array(array=w369, length=1 ("长度"), index=2 ("索引")) -> (array with subset deleted=w370:string[])  [unwired: 1 out]
                                n205 = call <vilib>:"Clear Errors.vi"("error in (no error)"=w372) -> ("error out"=w371:errorcluster)  [unwired: 5 in, 1 out]
                                n206 = Concatenate Strings("WHERE CODE_ID ='" ("condition"), w354, "'") -> (w365:string)
                                n207 = call <vilib>:"DB Tools Update Data.vi"("condition"=w365, "data"=w358, "error in (no error)"=w371, "columns"=w370, "table"=w373, "connection reference"=w357) -> ("error out"=w355:errorcluster, "connection reference out"=w356:T15)  [unwired: 4 in]
                                }
                              }
                            }
                            n208 = call <vilib>:"Simple Error Handler.vi"("error in (no error)"=w337) -> ()  [unwired: 4 in, 5 out]
                          }
                        }
                      }
                    }
                  }
                  frame #2 {
                    n209 = shared-variable "我的电脑\\Modbus.lvlib\\左工位启用"() -> (w374:u16)  [unwired: 1 in, 1 out]
                    n210 = case shown="1" w374 {
                      frame 0, Default {
                      }
                      frame 1 {
                        n211 = global read "Global1.vi" "联机模式"() -> (w375:enum16{"单机", "追溯"})
                        n212 = case shown="\"追溯\"" w375 {
                          tunnel: w375 -> [_ w385]
                          frame "单机", Default {
                          }
                          frame "追溯" {
                            w378 = "Nm"
                            n213 = call "GetSQLstring1.vi"("联机模式"=w385) -> ("错误输出"=w433:errorcluster, "连接字符串"=w434:string)  [unwired: 9 in]
                            n214 = local read "左逆小结果"() -> (w398:string)
                            n215 = local read "左逆大结果"() -> (w397:string)
                            n216 = local read "最小值下限"() -> (w409:dbl)
                            n217 = local read "最小值上限"() -> (w408:dbl)
                            n218 = local read "左逆波结果"() -> (w396:string)
                            n219 = local read "最大值下限"() -> (w406:dbl)
                            n220 = local read "最大值上限"() -> (w405:dbl)
                            n221 = local read "左逆平结果"() -> (w395:string)
                            n222 = local read "波动值下限"() -> (w403:dbl)
                            n223 = local read "波动值上限"() -> (w402:dbl)
                            n224 = local read "左正小结果"() -> (w394:string)
                            n225 = local read "平均值下限"() -> (w400:dbl)
                            n226 = local read "平均值上限"() -> (w399:dbl)
                            n227 = local read "左正大结果"() -> (w393:string)
                            n228 = local read "左正波结果"() -> (w392:string)
                            n229 = local read "左正平结果"() -> (w391:string)
                            n230 = local read "DEVICEID"() -> (w427:string)
                            n231 = local read "平均值差上限"() -> (w379:dbl)
                            n232 = local read "平均值差下限"() -> (w380:dbl)
                            n233 = local read "左正平结果"() -> (w377:string)
                            n234 = local read "LEFTCODEID"() -> (w425:string)
                            n235 = local read "左工位逆向最小扭矩(Nm)"() -> (w414:dbl)
                            n236 = local read "左工位逆向最大扭矩(Nm)"() -> (w413:dbl)
                            n237 = local read "左工位逆向波动扭矩(Nm)"() -> (w412:dbl)
                            n238 = local read "左工位逆向平均扭矩(Nm)"() -> (w411:dbl)
                            n239 = local read "左工位正向最小扭矩(Nm)"() -> (w410:dbl)
                            n240 = local read "左工位正向最大扭矩(Nm)"() -> (w407:dbl)
                            n241 = local read "左工位正向波动扭矩(Nm)"() -> (w404:dbl)
                            n242 = local read "左工位正向平均扭矩(Nm)"() -> (w401:dbl)
                            n243 = local read "左工位正逆平均扭矩差(Nm)"() -> (w381:dbl)
                            n244 = Decimal String To Number(string=w427, default (0L)=i64 0 ("默认(0 I32)")) -> (number=w384:i64)  [unwired: 1 in, 1 out]
                            n245 = Decimal String To Number(string=w425, default (0L)=i64 0 ("默认(0 I32)")) -> (number=w383:i64)  [unwired: 1 in, 1 out]
                            n246 = Bundle(w384, w383, "逆向空载最小扭矩", "左工位逆向最小扭矩(Nm)"=w414, "最小值下限"=w409, "最小值上限"=w408, w378, "左逆小结果"=w398) -> (w429:T20)  [unwired: 1 in]
                            n247 = Bundle(w384, w383, "逆向空载最大扭矩  ", "左工位逆向最大扭矩(Nm)"=w413, "最大值下限"=w406, "最大值上限"=w405, w378, "左逆大结果"=w397) -> (w416:T21)  [unwired: 1 in]
                            n248 = Bundle(w384, w383, "逆向空载波动扭矩  ", "左工位逆向波动扭矩(Nm)"=w412, "波动值下限"=w403, "波动值上限"=w402, w378, "左逆波结果"=w396) -> (w415:T22)  [unwired: 1 in]
                            n249 = Bundle(w384, w383, "逆向空载平均扭矩  ", "左工位逆向平均扭矩(Nm)"=w411, "平均值下限"=w400, "平均值上限"=w399, w378, "左逆平结果"=w395) -> (w390:T23)  [unwired: 1 in]
                            n250 = Bundle(w384, w383, "正向空载最小扭矩  ", "左工位正向最小扭矩(Nm)"=w410, "最小值下限"=w409, "最小值上限"=w408, w378, "左正小结果"=w394) -> (w389:T24)  [unwired: 1 in]
                            n251 = Bundle(w384, w383, "正向空载最大扭矩  ", "左工位正向最大扭矩(Nm)"=w407, "最大值下限"=w406, "最大值上限"=w405, w378, "左正大结果"=w393) -> (w388:T25)  [unwired: 1 in]
                            n252 = Bundle(w384, w383, "正向空载波动扭矩  ", "左工位正向波动扭矩(Nm)"=w404, "波动值下限"=w403, "波动值上限"=w402, w378, "左正波结果"=w392) -> (w387:T26)  [unwired: 1 in]
                            n253 = Bundle(w384, w383, "正向空载平均扭矩  ", "左工位正向平均扭矩(Nm)"=w401, "平均值下限"=w400, "平均值上限"=w399, w378, "左正平结果"=w391) -> (w386:T27)  [unwired: 1 in]
                            n254 = Bundle(w384, w383, "正逆向平均扭矩  ", "左工位正逆平均扭矩差(Nm)"=w381, "平均值差下限"=w380, "平均值差上限"=w379, w378, "左正平结果"=w377) -> (w376:T28)  [unwired: 1 in]
                            n255 = Build Array(w429, w416, w415, w390, w389, w388, w387, w386, w376) -> (w428:T29)
                            n256 = call-poly <vilib>:"DB Tools Open Connection.vi"("error in (no error)"=w433, "connection information"=w434) -> ("error out"=w435:errorcluster, "connection reference"=w432:T15)  [unwired: 6 in]
                            n257 = for {
                              tunnel: w428 -> [w440] mode=indexing
                              tunnel: w432 -> [w438]
                              shift-right: [w436] -> w430
                              shift-left: w435 -> [w443]
                              w439 = string[] ["DEVICE_ID", "CODE_ID", "TEST_NAME", "TEST_VALUE", "TEST_VALUE_MIN", "TEST_VALUE_MAX", "TEST_VALUE_UNIT", "TEST_VALUE_RESULT"] ("columns")
                              w441 = "Test" ("table")
                              n258 = call <vilib>:"DB Tools Insert Data.vi"("data"=w440, "error in (no error)"=w443, "columns"=w439, "table"=w441, "connection reference"=w438) -> ("error out"=w442:errorcluster, "connection reference out"=w437:T15)  [unwired: 5 in]
                              n259 = case shown="错误" w442 {
                                selector: w442 -> [w444 w469]
                                tunnel: w439 -> [_ w466]
                                tunnel: w437 -> [w445 w451]
                                tunnel: w441 -> [_ w470]
                                tunnel: w440 -> [_ w460]
                                tunnel: [w445 w450] -> _
                                tunnel: [w444 w449] -> w436
                                frame No Error {
                                }
                                frame Error {
                                n260 = Unbundle(w460) -> (w459:i64, w447:i64, w452:string, "左工位正逆平均扭矩差(Nm)"=w458:dbl, "平均值差下限"=w457:dbl, "平均值差上限"=w456:dbl, w455:string, "左正平结果"=w454:string)
                                n261 = Bundle(w459, w447, "左工位正逆平均扭矩差(Nm)"=w458, "平均值差下限"=w457, "平均值差上限"=w456, w455, "左正平结果"=w454) -> (w453:T30)  [unwired: 1 in]
                                n262 = Number To Decimal String(number=w447) -> (decimal integer string=w446:string)  [unwired: 1 in]
                                n263 = call <vilib>:"Clear Errors.vi"("error in (no error)"=w469) -> ("error out"=w468:errorcluster)  [unwired: 5 in, 1 out]
                                n264 = Concatenate Strings("WHERE TEST_NAME ='" ("condition"), w452, "' ", "AND CODE_ID =" ("condition"), w446) -> (w462:string)
                                n265 = Delete From Array(array=w466, length=1 ("长度"), index=2 ("索引")) -> (array with subset deleted=w467:string[])  [unwired: 1 out]
                                n266 = call <vilib>:"DB Tools Update Data.vi"("condition"=w462, "data"=w453, "error in (no error)"=w468, "columns"=w467, "table"=w470, "connection reference"=w451) -> ("error out"=w449:errorcluster, "connection reference out"=w450:T15)  [unwired: 4 in]
                                }
                              }
                            }
                            n267 = call <vilib>:"Simple Error Handler.vi"("error in (no error)"=w430) -> ()  [unwired: 4 in, 5 out]
                          }
                        }
                      }
                    }
                  }
                  frame #3 {
                    n268 = shared-variable "我的电脑\\Modbus.lvlib\\左工位启用"() -> (w471:u16)  [unwired: 1 in, 1 out]
                    n269 = case shown="1" w471 {
                      frame 0, Default {
                      }
                      frame 1 {
                        n270 = global read "Global1.vi" "联机模式"() -> (w472:enum16{"单机", "追溯"})
                        n271 = case shown="\"追溯\"" w472 {
                          tunnel: w472 -> [_ w499]
                          frame "单机", Default {
                          }
                          frame "追溯" {
                            n272 = call "GetSQLstring1.vi"("联机模式"=w499) -> ("错误输出"=w497:errorcluster, "连接字符串"=w498:string)  [unwired: 9 in]
                            n273 = local read "DEVICEID"() -> (w492:string)
                            n274 = local read "USERID"() -> (w474:string)
                            n275 = Get Date/Time String(date format (0)=enum16{"short", "long", "abbreviated"}."short" ("日期格式(0)"), want seconds? (F)=FALSE ("需要秒？(F)")) -> (date string=w484:string, time string=w483:string)  [unwired: 1 in]
                            n276 = local read "LEFTCODEID"() -> (w489:string)
                            n277 = local read "LEFTRESULT"() -> (w473:string)
                            n278 = Decimal String To Number(string=w492, default (0L)=i64 0 ("默认(0 I32)")) -> (number=w490:i64)  [unwired: 1 in, 1 out]
                            n279 = Decimal String To Number(string=w474, default (0L)=i64 0 ("默认(0 I32)")) -> (number=w475:i64)  [unwired: 1 in, 1 out]
                            n280 = Concatenate Strings(w484, " " ("字符串"), w483) -> (w480:string)
                            n281 = Decimal String To Number(string=w489, default (0L)=i64 0 ("默认(0 I32)")) -> (number=w487:i64)  [unwired: 1 in, 1 out]
                            n282 = Search and Replace String(replace all?=TRUE ("替换全部？(F)"), input string=w480, search string="/" ("替换字符串(\"\")"), replace string="-" ("替换字符串(\"\")")) -> (result string=w481:string)  [unwired: 4 in, 3 out]
                            n283 = Bundle(w490, w475, w487, "LEFTRESULT"=w473, "result string"=w481) -> (w494:T31)  [unwired: 1 in]
                            n284 = Build Array(w494) -> (w493:T32)
                            n285 = call-poly <vilib>:"DB Tools Open Connection.vi"("error in (no error)"=w497, "connection information"=w498) -> ("error out"=w500:errorcluster, "connection reference"=w496:T15)  [unwired: 6 in]
                            n286 = for {
                              tunnel: w493 -> [w505] mode=indexing
                              tunnel: w496 -> [w503]
                              shift-right: [w501] -> w495
                              shift-left: w500 -> [w508]
                              w504 = string[] ["DEVICE_ID", "USER_ID", "CODE_ID", "RESULT_VALUE", "RESULT_TIME"] ("columns")
                              w506 = "Result" ("table")
                              n287 = call <vilib>:"DB Tools Insert Data.vi"("data"=w505, "error in (no error)"=w508, "columns"=w504, "table"=w506, "connection reference"=w503) -> ("error out"=w507:errorcluster, "connection reference out"=w502:T15)  [unwired: 5 in]
                              n288 = case shown="错误" w507 {
                                selector: w507 -> [w509 w530]
                                tunnel: w504 -> [_ w527]
                                tunnel: w502 -> [w510 w518]
                                tunnel: w506 -> [_ w531]
                                tunnel: w505 -> [_ w522]
                                tunnel: [w510 w517] -> _
                                tunnel: [w509 w516] -> w501
                                frame No Error {
                                }
                                frame Error {
                                n289 = Unbundle(w522) -> (w511:i64, w514:i64, "LEFTRESULT"=w521:string, "result string"=w520:string)  [unwired: 1 out]
                                n290 = Bundle("LEFTRESULT"=w521, "result string"=w520) -> (w519:T33)  [unwired: 1 in]
                                n291 = Array Subset(array=w527, index=3 ("长度"), length=2 ("索引")) -> (w528:string[])
                                n292 = Number To Decimal String(number=w514) -> (decimal integer string=w515:string)  [unwired: 1 in]
                                n293 = Number To Decimal String(number=w511) -> (decimal integer string=w512:string)  [unwired: 1 in]
                                n294 = Concatenate Strings("WHERE CODE_ID =" ("condition"), w515, "AND DEVICE_ID=", w512) -> (w513:string)
                                n295 = call <vilib>:"Clear Errors.vi"("error in (no error)"=w530) -> ("error out"=w529:errorcluster)  [unwired: 5 in, 1 out]
                                n296 = call <vilib>:"DB Tools Update Data.vi"("condition"=w513, "data"=w519, "error in (no error)"=w529, "columns"=w528, "table"=w531, "connection reference"=w518) -> ("error out"=w516:errorcluster, "connection reference out"=w517:T15)  [unwired: 4 in]
                                }
                              }
                            }
                            n297 = call <vilib>:"Simple Error Handler.vi"("error in (no error)"=w495) -> ()  [unwired: 4 in, 5 out]
                          }
                        }
                      }
                    }
                  }
                  frame #4 {
                    n298 = Wait (ms)(milliseconds to wait=u32 1000 ("等待时间（毫秒）")) -> ()  [unwired: 1 out]
                  }
                  frame #5 {
                    n299 = local write "字符串"("0" ("字符串")) -> ()
                  }
                }
              }
            }
            n300 = case shown="1001" w206 {
              frame 0, Default {
              }
              frame 500 {
                n301 = local read "力位移曲线 4"() -> (w1091:cluster{dbl[], dbl[]}[])
                n302 = for {
                  tunnel: [w1095] -> w1092 mode=indexing
                  tunnel: w1091 -> [w1094] mode=indexing
                  i -> [w1093]
                  n303 = case shown="2" w1093 {
                    tunnel: [w1096 w1110] -> w1095
                    tunnel: w1094 -> [w1096 w1109]
                    frame Default {
                    }
                    frame 2 {
                      n304 = local read "左空载系数"() -> (w1104:dbl)
                      n305 = local write "Initialize 2"(FALSE ("Initialize 2")) -> ()
                      n306 = global read "全局1.vi" "左加载"() -> (w1101:dbl)
                      n307 = global read "Global.vi" "空载速度(°/s)"() -> (w1097:dbl)
                      n308 = case shown="假" "Initialize 2" {
                        tunnel: [w1115 0.0] -> w1099
                        frame False {
                          n309 = global read "全局 1.vi" "工位2正向磨合开始时间"() -> (w1116:u32)
                          n310 = Tick Count (ms)() -> (millisecond timer value=w1119:u32)
                          n311 = Subtract(x=w1119, y=w1116) -> (x-y=w1118:u32)
                          n312 = Divide(x=w1118, y=u32 1000) -> (x/y=w1115:dbl)
                          n313 = global write "全局 1.vi" "工位2正向磨合结束时间"(w1115) -> ()
                        }
                        frame True {
                          n314 = Tick Count (ms)() -> (millisecond timer value=w1121:u32)
                          n315 = global write "全局 1.vi" "工位2正向磨合开始时间"(w1121) -> ()
                        }
                      }
                      n316 = Subtract(x=w1101, y=0.0) -> (x-y=w1105:dbl)
                      n317 = shared-variable "我的电脑\\Modbus.lvlib\\加载传感器偏移值"() -> (w1108:sgl[])  [unwired: 1 in, 1 out]
                      n318 = Multiply(x=w1105, y=w1104) -> (x*y=w1103:dbl)
                      n319 = Unbundle(w1109) -> (w1114:dbl[], w1113:dbl[])
                      n320 = Build Array (concatenate)(w1113, w1103) -> (w1111:dbl[])
                      n321 = Index Array(array=w1108, index=0) -> ()  [unwired: 1 out]
                      n322 = Multiply(x=w1097, y=w1099) -> (x*y=w1098:dbl)
                      n323 = Build Array (concatenate)(w1114, w1098) -> (w1112:dbl[])
                      n324 = Bundle(w1112, w1111) -> (w1110:cluster{dbl[], dbl[]})  [unwired: 1 in]
                    }
                  }
                }
                n325 = local write "力位移曲线 4"(w1092) -> ()
              }
              frame 600 {
                n326 = local read "力位移曲线 4"() -> (w1122:cluster{dbl[], dbl[]}[])
                n327 = for {
                  tunnel: [w1126] -> w1123 mode=indexing
                  tunnel: w1122 -> [w1125] mode=indexing
                  i -> [w1124]
                  n328 = case shown="3" w1124 {
                    tunnel: [w1127 w1141] -> w1126
                    tunnel: w1125 -> [w1127 w1140]
                    frame Default {
                    }
                    frame 3 {
                      n329 = local write "Initialize 4"(FALSE ("Initialize 2")) -> ()
                      n330 = local read "左逆向空载"() -> (w1128:dbl)
                      n331 = global read "全局1.vi" "左加载"() -> (w1133:dbl)
                      n332 = global read "Global.vi" "空载速度(°/s)"() -> (w1129:dbl)
                      n333 = case shown="假" "Initialize 4" {
                        tunnel: [w1146 w1153] -> w1131
                        frame False {
                          n334 = global read "全局 1.vi" "工位2正向磨合结束时间"() -> (w1148:dbl)
                          n335 = global read "全局 1.vi" "工位2逆向磨合开始时间"() -> (w1149:u32)
                          n336 = Tick Count (ms)() -> (millisecond timer value=w1152:u32)
                          n337 = Subtract(x=w1152, y=w1149) -> (x-y=w1151:u32)
                          n338 = Divide(x=w1151, y=u32 1000) -> (x/y=w1147:dbl)
                          n339 = Subtract(x=w1148, y=w1147) -> (x-y=w1146:dbl)
                        }
                        frame True {
                          n340 = Tick Count (ms)() -> (millisecond timer value=w1154:u32)
                          n341 = global write "全局 1.vi" "工位2逆向磨合开始时间"(w1154) -> ()
                          n342 = global read "全局 1.vi" "工位2正向磨合结束时间"() -> (w1153:dbl)
                        }
                      }
                      n343 = Subtract(x=w1133, y=0.0) -> (x-y=w1136:dbl)
                      n344 = shared-variable "我的电脑\\Modbus.lvlib\\加载传感器偏移值"() -> (w1139:sgl[])  [unwired: 1 in, 1 out]
                      n345 = Multiply(x=w1136, y=w1128) -> (x*y=w1135:dbl)
                      n346 = Unbundle(w1140) -> (w1145:dbl[], w1144:dbl[])
                      n347 = Build Array (concatenate)(w1144, w1135) -> (w1142:dbl[])
                      n348 = Index Array(array=w1139, index=1) -> ()  [unwired: 1 out]
                      n349 = Multiply(x=w1131, y=w1129) -> (x*y=w1130:dbl)
                      n350 = Build Array (concatenate)(w1145, w1130) -> (w1143:dbl[])
                      n351 = Bundle(w1143, w1142) -> (w1141:cluster{dbl[], dbl[]})  [unwired: 1 in]
                    }
                  }
                }
                n352 = local write "力位移曲线 4"(w1123) -> ()
              }
              frame 700 {
                n353 = local read "左扭矩波动"() -> (w1163:dbl)
                n354 = local read "判定框参数"() -> (w1190:string[][])
                n355 = local read "左平均扭矩系数"() -> (w1168:dbl)
                n356 = local read "力位移曲线 4"() -> (w1219:cluster{dbl[], dbl[]}[])
                n357 = local read "力位移曲线 4"() -> (w1203:cluster{dbl[], dbl[]}[])
                n358 = Index Array(array=w1190, index (row) #1=4 ("索引 (行)"), index (row) #2=5 ("索引 (行)"), index (row) #3=0 ("索引 (行)"), index (row) #4=1 ("索引 (行)")) -> (element #1=w1182:string[], element #2=w1183:string[], element #3=w1184:string[], element #4=w1185:string[])  [unwired: 4 in]
                n359 = Index Array(array=w1219) -> (element #4=w1214:cluster{dbl[], dbl[]})  [unwired: 4 in, 3 out]
                n360 = Index Array(array=w1203) -> (element #3=w1196:cluster{dbl[], dbl[]})  [unwired: 4 in, 3 out]
                n361 = Unbundle(w1214) -> (w1209:dbl[], w1211:dbl[])
                n362 = Index Array(array=w1182, index=1 ("索引")) -> (element=w1186:string)
                n363 = Index Array(array=w1183, index=1 ("索引")) -> (element=w1187:string)
                n364 = Index Array(array=w1184, index=1 ("索引")) -> (element=w1188:string)
                n365 = Index Array(array=w1185, index=1 ("索引")) -> (element=w1189:string)
                n366 = Fract/Exp String To Number(string=w1186) -> (number=w1170:dbl)  [unwired: 3 in, 1 out]
                n367 = Fract/Exp String To Number(string=w1187) -> (number=w1171:dbl)  [unwired: 3 in, 1 out]
                n368 = Fract/Exp String To Number(string=w1188) -> (number=w1172:dbl)  [unwired: 3 in, 1 out]
                n369 = Fract/Exp String To Number(string=w1189) -> (number=w1173:dbl)  [unwired: 3 in, 1 out]
                n370 = Reverse 1D Array(array=w1209) -> (reversed array=w1210:dbl[])
                n371 = Unbundle(w1196) -> (w1201:dbl[], w1202:dbl[])
                n372 = Threshold 1D Array(2:w1170, 3:w1210) -> (0:w1218:dbl)  [unwired: 1 in]
                n373 = Threshold 1D Array(2:w1172, 3:w1201) -> (0:w1200:dbl)  [unwired: 1 in]
                n374 = Reverse 1D Array(array=w1211) -> (reversed array=w1212:dbl[])
                n375 = Split 1D Array(array=w1212, index=w1218) -> (second subarray=w1217:dbl[])  [unwired: 1 out]
                n376 = Split 1D Array(array=w1202, index=w1200) -> (second subarray=w1199:dbl[])  [unwired: 1 out]
                n377 = Split 1D Array(array=w1210, index=w1218) -> (second subarray=w1216:dbl[])  [unwired: 1 out]
                n378 = Split 1D Array(array=w1201, index=w1200) -> (second subarray=w1198:dbl[])  [unwired: 1 out]
                n379 = Threshold 1D Array(2:w1171, 3:w1216) -> (0:w1215:dbl)  [unwired: 1 in]
                n380 = Threshold 1D Array(2:w1173, 3:w1198) -> (0:w1197:dbl)  [unwired: 1 in]
                n381 = Split 1D Array(array=w1216, index=w1215) -> ()  [unwired: 2 out]
                n382 = Split 1D Array(array=w1198, index=w1197) -> ()  [unwired: 2 out]
                n383 = Split 1D Array(array=w1217, index=w1215) -> (first subarray=w1213:dbl[])  [unwired: 1 out]
                n384 = Split 1D Array(array=w1199, index=w1197) -> (first subarray=w1195:dbl[])  [unwired: 1 out]
                n385 = call-poly <vilib>:"Mean.vi"("X"=w1213) -> ("mean"=w1208:dbl)  [unwired: 1 out]
                n386 = call-poly <vilib>:"Mean.vi"("X"=w1195) -> ("mean"=w1191:dbl)  [unwired: 1 out]
                n387 = Array Max & Min(array=w1213) -> (max value=w1160:dbl, min value=w1159:dbl)  [unwired: 2 out]
                n388 = Array Max & Min(array=w1195) -> (max value=w1162:dbl, min value=w1161:dbl)  [unwired: 2 out]
                n389 = Subtract(x=w1160, y=w1159) -> (x-y=w1206:dbl)
                n390 = Subtract(x=w1161, y=w1162) -> (x-y=w1192:dbl)
                n391 = Absolute Value(x=w1160) -> (abs(x)=→"左工位逆向最小扭矩(Nm)":dbl)
                n392 = Absolute Value(x=w1159) -> (abs(x)=→"左工位逆向最大扭矩(Nm)":dbl)
                n393 = Absolute Value(x=w1208) -> (abs(x)=w1207:dbl)
                n394 = Absolute Value(x=w1162) -> (abs(x)=→"左工位正向最大扭矩(Nm)":dbl)
                n395 = Absolute Value(x=w1161) -> (abs(x)=→"左工位正向最小扭矩(Nm)":dbl)
                n396 = Absolute Value(x=w1191) -> (abs(x)=w1169:dbl)
                n397 = Multiply(x=w1168, y=w1207) -> (x*y=w1158:dbl)
                "左工位逆向平均扭矩(Nm)" <- w1158
                n398 = Multiply(x=w1169, y=w1168) -> (x*y=w1157:dbl)
                "左工位正向平均扭矩(Nm)" <- w1157
                n399 = Absolute Value(x=w1206) -> (abs(x)=w1167:dbl)
                n400 = Absolute Value(x=w1192) -> (abs(x)=w1165:dbl)
                n401 = Subtract(x=w1158, y=w1157) -> (x-y=w1156:dbl)
                n402 = Multiply(x=w1167, y=w1163) -> (x*y=→"左工位逆向波动扭矩(Nm)":dbl)
                n403 = Multiply(x=w1165, y=w1163) -> (x*y=→"左工位正向波动扭矩(Nm)":dbl)
                n404 = Absolute Value(x=w1156) -> (abs(x)=→"左工位正逆平均扭矩差(Nm)":dbl)
              }
              frame 1 {
                n405 = stacked-sequence {
                  frame #0 {
                    n406 = Wait (ms)(milliseconds to wait=u32 200 ("等待时间（毫秒）")) -> ()  [unwired: 1 out]
                    n407 = control-ref of="力位移曲线 4"() -> (w1263:refnum<vi>)
                    n408 = local read "结果判定参数"() -> (w1285:string[][])
                    n409 = global write "A131258.vi" "左工位空载曲线"(w1263) -> ()
                    n410 = local read "左工位逆向最大扭矩(Nm)"() -> (w1245:dbl)
                    n411 = local read "左工位正向最大扭矩(Nm)"() -> (w1243:dbl)
                    n412 = local read "左工位逆向波动扭矩(Nm)"() -> (w1311:dbl)
                    n413 = local read "左工位正向平均扭矩(Nm)"() -> (w1310:dbl)
                    n414 = local read "左工位正向波动扭矩(Nm)"() -> (w1315:dbl)
                    n415 = local read "左工位逆向平均扭矩(Nm)"() -> (w1307:dbl)
                    n416 = local read "左工位逆向最小扭矩(Nm)"() -> (w1239:dbl)
                    n417 = local read "左工位正向最小扭矩(Nm)"() -> (w1235:dbl)
                    n418 = Index Array(array=w1285, index (row) #1=0 ("索引 (行)"), index (row) #2=0 ("索引 (行)"), index (row) #3=1 ("索引 (行)"), index (row) #4=1 ("索引 (行)"), index (row) #5=2 ("索引 (行)"), index (row) #6=2 ("索引 (行)"), index (row) #7=3 ("索引 (行)"), index (row) #8=4 ("索引 (行)")) -> (element #1=w1293:string[], element #2=w1292:string[], element #3=w1291:string[], element #4=w1290:string[], element #5=w1282:string[], element #6=w1281:string[], element #7=w1257:string[], element #8=w1231:string[])  [unwired: 8 in]
                    n419 = local read "左工位正逆平均扭矩差(Nm)"() -> (w1224:dbl)
                    n420 = Index Array(array=w1231, index #1=1 ("索引"), index #2=2 ("索引")) -> (element #1=w1228:string, element #2=w1227:string)
                    n421 = Index Array(array=w1293, index=1 ("索引")) -> (element=w1289:string)
                    n422 = Index Array(array=w1292, index=2 ("索引")) -> (element=w1288:string)
                    n423 = Index Array(array=w1291, index=1 ("索引")) -> (element=w1287:string)
                    n424 = Index Array(array=w1290, index=2 ("索引")) -> (element=w1286:string)
                    n425 = Index Array(array=w1282, index=1 ("索引")) -> (element=w1284:string)
                    n426 = Index Array(array=w1281, index=2 ("索引")) -> (element=w1283:string)
                    n427 = Index Array(array=w1257, index #1=2 ("索引"), index #2=1 ("索引")) -> (element #1=w1259:string, element #2=w1237:string)
                    n428 = Fract/Exp String To Number(string=w1228) -> (number=w1226:dbl)  [unwired: 3 in, 1 out]
                    n429 = Fract/Exp String To Number(string=w1227) -> (number=w1225:dbl)  [unwired: 3 in, 1 out]
                    n430 = Fract/Exp String To Number(string=w1289) -> (number=w1242:dbl)  [unwired: 3 in, 1 out]
                    n431 = Fract/Exp String To Number(string=w1288) -> (number=w1241:dbl)  [unwired: 3 in, 1 out]
                    n432 = Fract/Exp String To Number(string=w1287) -> (number=w1267:dbl)  [unwired: 3 in, 1 out]
                    n433 = Fract/Exp String To Number(string=w1286) -> (number=w1266:dbl)  [unwired: 3 in, 1 out]
                    n434 = Fract/Exp String To Number(string=w1284) -> (number=w1265:dbl)  [unwired: 3 in, 1 out]
                    n435 = Fract/Exp String To Number(string=w1283) -> (number=w1264:dbl)  [unwired: 3 in, 1 out]
                    n436 = Fract/Exp String To Number(string=w1237) -> (number=w1234:dbl)  [unwired: 3 in, 1 out]
                    n437 = Fract/Exp String To Number(string=w1259) -> (number=w1233:dbl)  [unwired: 3 in, 1 out]
                    n438 = In Range and Coerce(upper limit=w1226, x=w1224, lower limit=w1225) -> (In Range?=w1222:bool)  [unwired: 1 out]
                    n439 = Greater Or Equal?(x=w1267, y=w1311) -> (x >= y?=w1268:bool)
                    n440 = Greater Or Equal?(x=w1311, y=w1266) -> (x >= y?=w1312:bool)
                    n441 = Greater Or Equal?(x=w1265, y=w1310) -> (x >= y?=w1309:bool)
                    n442 = Greater Or Equal?(x=w1310, y=w1264) -> (x >= y?=w1308:bool)
                    n443 = Greater Or Equal?(x=w1267, y=w1315) -> (x >= y?=w1314:bool)
                    n444 = Greater Or Equal?(x=w1315, y=w1266) -> (x >= y?=w1313:bool)
                    n445 = Greater Or Equal?(x=w1265, y=w1307) -> (x >= y?=w1306:bool)
                    n446 = Greater Or Equal?(x=w1307, y=w1264) -> (x >= y?=w1305:bool)
                    n447 = In Range and Coerce(upper limit=w1242, x=w1245, lower limit=w1241) -> (In Range?=w1246:bool)  [unwired: 1 out]
                    n448 = In Range and Coerce(upper limit=w1242, x=w1243, lower limit=w1241) -> (In Range?=w1244:bool)  [unwired: 1 out]
                    n449 = In Range and Coerce(upper limit=w1234, x=w1239, lower limit=w1233) -> (In Range?=w1240:bool)  [unwired: 1 out]
                    n450 = In Range and Coerce(upper limit=w1234, x=w1235, lower limit=w1233) -> (In Range?=w1236:bool)  [unwired: 1 out]
                    n451 = case shown="真" w1246 {
                      tunnel: [u32 16711680 u32 56369] -> w1252
                      frame False {
                        n452 = local write "左逆大结果"("NG" ("LEFTRESULT")) -> ()
                      }
                      frame True {
                        n453 = local write "左逆大结果"("OK" ("LEFTRESULT")) -> ()
                      }
                    }
                    n454 = case shown="真" w1240 {
                      tunnel: [u32 16711680 u32 56369] -> w1255
                      frame False {
                        n455 = local write "左逆小结果"("NG" ("LEFTRESULT")) -> ()
                      }
                      frame True {
                        n456 = local write "左逆小结果"("OK" ("LEFTRESULT")) -> ()
                      }
                    }
                    n457 = case shown="假" w1244 {
                      tunnel: [u32 16711680 u32 56369] -> w1251
                      frame False {
                        n458 = local write "左正大结果"("NG" ("LEFTRESULT")) -> ()
                      }
                      frame True {
                        n459 = local write "左正大结果"("OK" ("LEFTRESULT")) -> ()
                      }
                    }
                    n460 = case shown="假" w1236 {
                      tunnel: [u32 16711680 u32 56369] -> w1256
                      frame False {
                        n461 = local write "左正小结果"("NG" ("LEFTRESULT")) -> ()
                      }
                      frame True {
                        n462 = local write "左正小结果"("OK" ("LEFTRESULT")) -> ()
                      }
                    }
                    n463 = case shown="真" w1222 {
                      tunnel: [u32 16711680 u32 56369] -> w1223
                      frame False {
                        n464 = local write "左平均差"("NG" ("LEFTRESULT")) -> ()
                      }
                      frame True {
                        n465 = local write "左平均差"("OK" ("LEFTRESULT")) -> ()
                      }
                    }
                    n466 = And(x=w1246, y=w1244) -> (x .and. y?=w1300:bool)
                    n467 = And(x=w1240, y=w1236) -> (x .and. y?=w1253:bool)
                    n468 = And(x=w1268, y=w1312) -> (x .and. y?=w1304:bool)
                    n469 = And(x=w1309, y=w1308) -> (x .and. y?=w1303:bool)
                    n470 = And(x=w1314, y=w1313) -> (x .and. y?=w1302:bool)
                    n471 = And(x=w1306, y=w1305) -> (x .and. y?=w1301:bool)
                    n472 = case shown="假" w1303 {
                      tunnel: [u32 16711680 u32 56369] -> w1247
                      frame False {
                        n473 = local write "左正平结果"("NG" ("LEFTRESULT")) -> ()
                      }
                      frame True {
                        n474 = local write "左正平结果"("OK" ("LEFTRESULT")) -> ()
                      }
                    }
                    n475 = case shown="假" w1301 {
                      tunnel: [u32 16711680 u32 56369] -> w1249
                      frame False {
                        n476 = local write "左逆平结果"("NG" ("LEFTRESULT")) -> ()
                      }
                      frame True {
                        n477 = local write "左逆平结果"("OK" ("LEFTRESULT")) -> ()
                      }
                    }
                    n478 = case shown="真" w1304 {
                      tunnel: [u32 16711680 u32 56369] -> w1248
                      frame False {
                        n479 = local write "左逆波结果"("NG" ("LEFTRESULT")) -> ()
                      }
                      frame True {
                        n480 = local write "左逆波结果"("OK" ("LEFTRESULT")) -> ()
                      }
                    }
                    n481 = case shown="真" w1302 {
                      tunnel: [u32 16711680 u32 56369] -> w1250
                      frame False {
                        n482 = local write "左正波结果"("NG" ("LEFTRESULT")) -> ()
                      }
                      frame True {
                        n483 = local write "左正波结果"("OK" ("LEFTRESULT")) -> ()
                      }
                    }
                    n484 = And(x=w1304, y=w1303) -> (x .and. y?=w1299:bool)
                    n485 = And(x=w1302, y=w1301) -> (x .and. y?=w1298:bool)
                    n486 = And(x=w1300, y=w1299) -> (x .and. y?=w1297:bool)
                    n487 = And(x=w1297, y=w1298) -> (x .and. y?=w1254:bool)
                    n488 = And(x=w1254, y=w1253) -> (x .and. y?=w1221:bool)
                    n489 = And(x=w1221, y=w1222) -> (x .and. y?=w1220:bool)
                    n490 = case shown="真" w1220 {
                      tunnel: [u16 2 ("左工位生产结果") u16 1 ("左工位生产结果")] -> w1296
                      tunnel: [FALSE ("合格指示灯") TRUE ("合格指示灯")] -> w1295
                      tunnel: [TRUE ("不合格指示灯") FALSE ("不合格指示灯")] -> w1294
                      tunnel: [bool[][] [[TRUE, FALSE]] ("判定结果") bool[][] [[TRUE, TRUE]] ("判定结果")] -> w1261
                      frame False {
                        n491 = local write "LEFTRESULT"("NG" ("LEFTRESULT")) -> ()
                      }
                      frame True {
                        "LEFTRESULT" <- "OK" ("LEFTRESULT")
                      }
                    }
                    "不合格指示灯  2" <- w1294
                    "合格指示灯 2" <- w1295
                    n492 = property on="左工位逆向最大扭矩(Nm)" class="DigNum (严格)"("NumText.BGColor"=w1252) -> ()  [unwired: 2 in, 2 out]
                    n493 = property on="左工位逆向最小扭矩(Nm)" class="DigNum (严格)"("NumText.BGColor"=w1255) -> ()  [unwired: 2 in, 2 out]
                    n494 = property on="左工位正向最大扭矩(Nm)" class="DigNum (严格)"("NumText.BGColor"=w1251) -> ()  [unwired: 2 in, 2 out]
                    n495 = property on="左工位正向最小扭矩(Nm)" class="DigNum (严格)"("NumText.BGColor"=w1256) -> ()  [unwired: 2 in, 2 out]
                    n496 = property on="左工位正逆平均扭矩差(Nm)" class="DigNum (严格)"("NumText.BGColor"=w1223) -> ()  [unwired: 2 in, 2 out]
                    n497 = property on="左工位正向平均扭矩(Nm)" class="DigNum (严格)"("NumText.BGColor"=w1247) -> ()  [unwired: 2 in, 2 out]
                    n498 = property on="左工位逆向平均扭矩(Nm)" class="DigNum (严格)"("NumText.BGColor"=w1249) -> ()  [unwired: 2 in, 2 out]
                    n499 = property on="左工位逆向波动扭矩(Nm)" class="DigNum (严格)"("NumText.BGColor"=w1248) -> ()  [unwired: 2 in, 2 out]
                    n500 = property on="左工位正向波动扭矩(Nm)" class="DigNum (严格)"("NumText.BGColor"=w1250) -> ()  [unwired: 2 in, 2 out]
                    n501 = shared-variable "我的电脑\\Modbus.lvlib\\左工位生产结果"(w1296) -> ()  [unwired: 1 in, 1 out]
                    n502 = local write "左工位判定结果 3"(w1261) -> ()
                  }
                  frame #1 {
                    n503 = stacked-sequence {
                      frame #0 {
                        n504 = Wait (ms)(milliseconds to wait=u32 500 ("等待时间（毫秒）")) -> ()  [unwired: 1 out]
                        n505 = call "浮动通知.vi"("通知内容"="报表生成中" ("Status")) -> ()  [unwired: 11 in]
                      }
                      frame #1 {
                      }
                    }
                    n506 = local read "最小值上限"() -> (w1384:dbl)
                    n507 = local read "最小值下限"() -> (w1382:dbl)
                    n508 = local read "最大值上限"() -> (w1440:dbl)
                    n509 = local read "最大值下限"() -> (w1439:dbl)
                    n510 = local read "波动值上限"() -> (w1436:dbl)
                    n511 = local read "波动值下限"() -> (w1435:dbl)
                    n512 = local read "平均值上限"() -> (w1428:dbl)
                    n513 = local read "平均值下限"() -> (w1426:dbl)
                    n514 = local read "最小值上限"() -> (w1375:dbl)
                    n515 = local read "最小值下限"() -> (w1377:dbl)
                    n516 = local read "最大值上限"() -> (w1415:dbl)
                    n517 = local read "最大值下限"() -> (w1413:dbl)
                    n518 = local read "波动值上限"() -> (w1402:dbl)
                    n519 = local read "波动值下限"() -> (w1401:dbl)
                    n520 = local read "平均值上限"() -> (w1393:dbl)
                    n521 = local read "平均值下限"() -> (w1392:dbl)
                    n522 = control-ref of="左工位报表"() -> (w1390:refnum<vi>)
                    n523 = local read "左工位正逆平均扭矩差(Nm)"() -> (w1364:dbl)
                    n524 = local read "平均值差上限"() -> (w1363:dbl)
                    n525 = local read "平均值差下限"() -> (w1362:dbl)
                    n526 = global write "Global.vi" "Result"(w1390) -> ()
                    n527 = local read "左工位正向最小扭矩(Nm)"() -> (w1443:dbl)
                    n528 = local read "左工位正向最大扭矩(Nm)"() -> (w1442:dbl)
                    n529 = local read "左工位正向波动扭矩(Nm)"() -> (w1437:dbl)
                    n530 = local read "左工位正向平均扭矩(Nm)"() -> (w1430:dbl)
                    n531 = local read "左工位逆向最小扭矩(Nm)"() -> (w1422:dbl)
                    n532 = local read "左工位逆向最大扭矩(Nm)"() -> (w1417:dbl)
                    n533 = local read "左工位逆向波动扭矩(Nm)"() -> (w1403:dbl)
                    n534 = local read "左工位逆向平均扭矩(Nm)"() -> (w1394:dbl)
                    n535 = Number To Fractional String(number=w1443, precision (6)=i16 3 ("精度(6)")) -> (F-format string=w1454:string)  [unwired: 2 in]
                    n536 = Number To Fractional String(number=w1384, precision (6)=i16 3 ("精度(6)")) -> (F-format string=w1380:string)  [unwired: 2 in]
                    n537 = Number To Fractional String(number=w1382, precision (6)=i16 3 ("精度(6)")) -> (F-format string=w1379:string)  [unwired: 2 in]
                    n538 = Number To Fractional String(number=w1442, precision (6)=i16 3 ("精度(6)")) -> (F-format string=w1452:string)  [unwired: 2 in]
                    n539 = Number To Fractional String(number=w1440, precision (6)=i16 3 ("精度(6)")) -> (F-format string=w1451:string)  [unwired: 2 in]
                    n540 = Number To Fractional String(number=w1439, precision (6)=i16 3 ("精度(6)")) -> (F-format string=w1449:string)  [unwired: 2 in]
                    n541 = Number To Fractional String(number=w1437, precision (6)=i16 3 ("精度(6)")) -> (F-format string=w1447:string)  [unwired: 2 in]
                    n542 = Number To Fractional String(number=w1436, precision (6)=i16 3 ("精度(6)")) -> (F-format string=w1446:string)  [unwired: 2 in]
                    n543 = Number To Fractional String(number=w1435, precision (6)=i16 3 ("精度(6)")) -> (F-format string=w1445:string)  [unwired: 2 in]
                    n544 = Number To Fractional String(number=w1430, precision (6)=i16 3 ("精度(6)")) -> (F-format string=w1432:string)  [unwired: 2 in]
                    n545 = Number To Fractional String(number=w1428, precision (6)=i16 3 ("精度(6)")) -> (F-format string=w1433:string)  [unwired: 2 in]
                    n546 = Number To Fractional String(number=w1426, precision (6)=i16 3 ("精度(6)")) -> (F-format string=w1434:string)  [unwired: 2 in]
                    n547 = Number To Fractional String(number=w1422, precision (6)=i16 3 ("精度(6)")) -> (F-format string=w1424:string)  [unwired: 2 in]
                    n548 = Number To Fractional String(number=w1375, precision (6)=i16 3 ("精度(6)")) -> (F-format string=w1374:string)  [unwired: 2 in]
                    n549 = Number To Fractional String(number=w1377, precision (6)=i16 3 ("精度(6)")) -> (F-format string=w1373:string)  [unwired: 2 in]
                    n550 = Number To Fractional String(number=w1417, precision (6)=i16 3 ("精度(6)")) -> (F-format string=w1418:string)  [unwired: 2 in]
                    n551 = Number To Fractional String(number=w1415, precision (6)=i16 3 ("精度(6)")) -> (F-format string=w1419:string)  [unwired: 2 in]
                    n552 = Number To Fractional String(number=w1413, precision (6)=i16 3 ("精度(6)")) -> (F-format string=w1420:string)  [unwired: 2 in]
                    n553 = Number To Fractional String(number=w1403, precision (6)=i16 3 ("精度(6)")) -> (F-format string=w1407:string)  [unwired: 2 in]
                    n554 = Number To Fractional String(number=w1402, precision (6)=i16 3 ("精度(6)")) -> (F-format string=w1406:string)  [unwired: 2 in]
                    n555 = Number To Fractional String(number=w1401, precision (6)=i16 3 ("精度(6)")) -> (F-format string=w1405:string)  [unwired: 2 in]
                    n556 = Number To Fractional String(number=w1394, precision (6)=i16 3 ("精度(6)")) -> (F-format string=w1398:string)  [unwired: 2 in]
                    n557 = Number To Fractional String(number=w1393, precision (6)=i16 3 ("精度(6)")) -> (F-format string=w1399:string)  [unwired: 2 in]
                    n558 = Number To Fractional String(number=w1392, precision (6)=i16 3 ("精度(6)")) -> (F-format string=w1400:string)  [unwired: 2 in]
                    n559 = Number To Fractional String(number=w1364, precision (6)=i16 3 ("精度(6)")) -> (F-format string=w1368:string)  [unwired: 2 in]
                    n560 = Number To Fractional String(number=w1363, precision (6)=i16 3 ("精度(6)")) -> (F-format string=w1367:string)  [unwired: 2 in]
                    n561 = Number To Fractional String(number=w1362, precision (6)=i16 3 ("精度(6)")) -> (F-format string=w1366:string)  [unwired: 2 in]
                    n562 = Build Array(w1454, w1380, w1379) -> (w1453:string[])
                    n563 = Build Array(w1452, w1451, w1449) -> (w1450:string[])
                    n564 = Build Array(w1447, w1446, w1445) -> (w1448:string[])
                    n565 = Build Array(w1432, w1433, w1434) -> (w1431:string[])
                    n566 = Build Array(w1424, w1374, w1373) -> (w1423:string[])
                    n567 = Build Array(w1418, w1419, w1420) -> (w1411:string[])
                    n568 = Build Array(w1407, w1406, w1405) -> (w1404:string[])
                    n569 = Build Array(w1398, w1399, w1400) -> (w1391:string[])
                    n570 = Build Array(w1368, w1367, w1366) -> (w1365:string[])
                    n571 = Build Array(w1453, w1450, w1448, w1431, w1423, w1411, w1404, w1391, w1365) -> (w1444:string[][])
                    n572 = local write "左工位报表"(w1444) -> ()
                    "字符串" <- "1" ("字符串")
                  }
                  frame #2 {
                    n573 = Wait (ms)(milliseconds to wait=u32 10 ("等待时间（毫秒）")) -> ()  [unwired: 1 out]
                    n574 = shared-variable "我的电脑\\Global.lvlib\\工位追溯码"() -> (w1460:string)  [unwired: 1 in, 1 out]
                    n575 = call "Report_A131258.vi"("文件重命名"=TRUE, "文件名称"=w1460, "布尔数组"="左工位判定结果 3") -> ()  [unwired: 8 in, 1 out]
                  }
                  frame #3 {
                    n576 = Wait (ms)(milliseconds to wait=u32 0 ("等待时间（毫秒）")) -> ()  [unwired: 1 out]
                  }
                  frame #4 {
                  }
                  frame #5 {
                  }
                  frame #6 {
                    n577 = shared-variable "我的电脑\\Modbus.lvlib\\左工位状态"(u16 1000 ("左工位状态")) -> ()  [unwired: 1 in, 1 out]
                  }
                }
              }
              frame 3 {
                w1471 = FALSE ("合格指示灯")
                w1464 = u32 13816530
                w1463 = 0
                n578 = shared-variable "我的电脑\\Modbus.lvlib\\左工位生产结果"(u16 0 ("左工位生产结果")) -> ()  [unwired: 1 in, 1 out]
                n579 = local write "左工位追溯码"("" ("左工位追溯码")) -> ()
                n580 = local write "合格指示灯 2"(w1471) -> ()
                n581 = local write "不合格指示灯  2"(w1471) -> ()
                n582 = property on="左工位正向波动扭矩(Nm)" class="DigNum (严格)"("NumText.BGColor"=w1464) -> ()  [unwired: 2 in, 2 out]
                n583 = property on="左工位正向平均扭矩(Nm)" class="DigNum (严格)"("NumText.BGColor"=w1464) -> ()  [unwired: 2 in, 2 out]
                n584 = property on="左工位正向最小扭矩(Nm)" class="DigNum (严格)"("NumText.BGColor"=w1464) -> ()  [unwired: 2 in, 2 out]
                n585 = property on="左工位逆向波动扭矩(Nm)" class="DigNum (严格)"("NumText.BGColor"=w1464) -> ()  [unwired: 2 in, 2 out]
                n586 = property on="左工位逆向最小扭矩(Nm)" class="DigNum (严格)"("NumText.BGColor"=w1464) -> ()  [unwired: 2 in, 2 out]
                n587 = property on="左工位逆向平均扭矩(Nm)" class="DigNum (严格)"("NumText.BGColor"=w1464) -> ()  [unwired: 2 in, 2 out]
                n588 = property on="左工位正向最大扭矩(Nm)" class="DigNum (严格)"("NumText.BGColor"=w1464) -> ()  [unwired: 2 in, 2 out]
                n589 = property on="左工位逆向最大扭矩(Nm)" class="DigNum (严格)"("NumText.BGColor"=w1464) -> ()  [unwired: 2 in, 2 out]
                n590 = property on="左工位正逆平均扭矩差(Nm)" class="DigNum (严格)"("NumText.BGColor"=w1464) -> ()  [unwired: 2 in, 2 out]
                n591 = local write "左工位逆向平均扭矩(Nm)"(w1463) -> ()
                n592 = local write "左工位正逆平均扭矩差(Nm)"(w1463) -> ()
                n593 = local write "左工位正向最小扭矩(Nm)"(w1463) -> ()
                n594 = local write "左工位正向平均扭矩(Nm)"(w1463) -> ()
                n595 = local write "左工位正向最大扭矩(Nm)"(w1463) -> ()
                n596 = local write "左工位正向波动扭矩(Nm)"(w1463) -> ()
                n597 = local write "左工位逆向最大扭矩(Nm)"(w1463) -> ()
                n598 = local write "左工位逆向最小扭矩(Nm)"(w1463) -> ()
                n599 = local write "左工位逆向波动扭矩(Nm)"(w1463) -> ()
                n600 = for {
                  N: 4 -> [_]
                  tunnel: [cluster{dbl[], dbl[]} {[], []}] -> w1469 mode=indexing
                }
                "力位移曲线 4" <- w1469
                n601 = shared-variable "我的电脑\\Modbus.lvlib\\空载速度"() -> (w1466:sgl)  [unwired: 1 in, 1 out]
                n602 = Multiply(x=w1466, y=sgl 6.0) -> (x*y=w1467:sgl)
                n603 = global write "Global.vi" "空载速度(°/s)"(w1467) -> ()
              }
              frame 200 {
                n604 = stacked-sequence {
                  frame #0 {
                    w1477 = FALSE ("合格指示灯")
                    w1474 = u32 13816530
                    w1475 = 0.0 ("正向空载最小扭矩(Nm)")
                    n605 = shared-variable "我的电脑\\Modbus.lvlib\\左工位生产结果"(u16 0 ("左工位生产结果")) -> ()  [unwired: 1 in, 1 out]
                    n606 = local write "左工位正逆平均扭矩差(Nm)"(w1475) -> ()
                    n607 = local write "合格指示灯 2"(w1477) -> ()
                    n608 = local write "不合格指示灯  2"(w1477) -> ()
                    n609 = local write "左工位正向最小扭矩(Nm)"(w1475) -> ()
                    n610 = local write "左工位正向最大扭矩(Nm)"(w1475) -> ()
                    n611 = local write "左工位正向波动扭矩(Nm)"(w1475) -> ()
                    n612 = local write "左工位正向平均扭矩(Nm)"(w1475) -> ()
                    n613 = local write "左工位逆向最小扭矩(Nm)"(w1475) -> ()
                    n614 = local write "左工位逆向最大扭矩(Nm)"(w1475) -> ()
                    n615 = local write "左工位逆向波动扭矩(Nm)"(w1475) -> ()
                    n616 = local write "左工位逆向平均扭矩(Nm)"(w1475) -> ()
                    n617 = property on="左工位正向波动扭矩(Nm)" class="DigNum (严格)"("NumText.BGColor"=w1474) -> ()  [unwired: 2 in, 2 out]
                    n618 = property on="左工位正向最小扭矩(Nm)" class="DigNum (严格)"("NumText.BGColor"=w1474) -> ()  [unwired: 2 in, 2 out]
                    n619 = property on="左工位正向平均扭矩(Nm)" class="DigNum (严格)"("NumText.BGColor"=w1474) -> ()  [unwired: 2 in, 2 out]
                    n620 = property on="左工位逆向最大扭矩(Nm)" class="DigNum (严格)"("NumText.BGColor"=w1474) -> ()  [unwired: 2 in, 2 out]
                    n621 = property on="左工位逆向最小扭矩(Nm)" class="DigNum (严格)"("NumText.BGColor"=w1474) -> ()  [unwired: 2 in, 2 out]
                    n622 = property on="左工位逆向波动扭矩(Nm)" class="DigNum (严格)"("NumText.BGColor"=w1474) -> ()  [unwired: 2 in, 2 out]
                    n623 = property on="左工位逆向平均扭矩(Nm)" class="DigNum (严格)"("NumText.BGColor"=w1474) -> ()  [unwired: 2 in, 2 out]
                    n624 = property on="左工位正向最大扭矩(Nm)" class="DigNum (严格)"("NumText.BGColor"=w1474) -> ()  [unwired: 2 in, 2 out]
                    n625 = for {
                      N: 4 -> [_]
                      tunnel: [cluster{dbl[], dbl[]} {[], []}] -> w1479 mode=indexing
                    }
                    n626 = property on="左工位正逆平均扭矩差(Nm)" class="DigNum (严格)"("NumText.BGColor"=w1474) -> ()  [unwired: 2 in, 2 out]
                    n627 = local write "力位移曲线 4"(w1479) -> ()
                  }
                  frame #1 {
                    w1481 = TRUE ("Initialize 2")
                    n628 = local write "Initialize 2"(w1481) -> ()
                    n629 = local write "Initialize 4"(w1481) -> ()
                    n630 = local read "力位移曲线 4"() -> (w1482:cluster{dbl[], dbl[]}[])
                    n631 = for {
                      tunnel: [w1486] -> w1483 mode=indexing
                      tunnel: w1482 -> [w1485] mode=indexing
                      i -> [w1484]
                      n632 = case shown="0" w1484 {
                        tunnel: [w1487 w1509] -> w1486
                        tunnel: w1485 -> [w1487 _]
                        frame Default {
                        }
                        frame 0 {
                          n633 = local read "判定框参数"() -> (w1500:string[][])
                          n634 = Index Array(array=w1500, index (row) #1=0 ("索引 (行)"), index (row) #2=1 ("索引 (行)"), index (row) #3=2 ("索引 (行)"), index (row) #4=3 ("索引 (行)")) -> (element #1=w1508:string[], element #2=w1507:string[], element #3=w1506:string[], element #4=w1505:string[])  [unwired: 4 in]
                          n635 = Index Array(array=w1508, index=1 ("索引")) -> (element=w1504:string)
                          n636 = Index Array(array=w1507, index=1 ("索引")) -> (element=w1503:string)
                          n637 = Index Array(array=w1506, index=1 ("索引")) -> (element=w1502:string)
                          n638 = Index Array(array=w1505, index=1 ("索引")) -> (element=w1501:string)
                          n639 = Fract/Exp String To Number(string=w1504) -> (number=w1490:dbl)  [unwired: 3 in, 1 out]
                          n640 = Fract/Exp String To Number(string=w1502) -> (number=w1488:dbl)  [unwired: 3 in, 1 out]
                          n641 = Fract/Exp String To Number(string=w1503) -> (number=w1491:dbl)  [unwired: 3 in, 1 out]
                          n642 = Fract/Exp String To Number(string=w1501) -> (number=w1489:dbl)  [unwired: 3 in, 1 out]
                          n643 = Build Array(w1491, w1491, w1490, w1490, w1491) -> (w1510:dbl[])
                          n644 = Build Array(w1489, w1488, w1488, w1489, w1489) -> (w1511:dbl[])
                          n645 = Bundle(w1510, w1511) -> (w1509:cluster{dbl[], dbl[]})  [unwired: 1 in]
                        }
                      }
                    }
                    n646 = local write "力位移曲线 4"(w1483) -> ()
                  }
                  frame #2 {
                    n647 = local read "力位移曲线 4"() -> (w1512:cluster{dbl[], dbl[]}[])
                    n648 = for {
                      tunnel: [w1516] -> w1513 mode=indexing
                      tunnel: w1512 -> [w1515] mode=indexing
                      i -> [w1514]
                      n649 = case shown="1" w1514 {
                        tunnel: [w1517 w1539] -> w1516
                        tunnel: w1515 -> [w1517 _]
                        frame Default {
                        }
                        frame 1 {
                          # "的事实"
                          n650 = local read "判定框参数"() -> (w1530:string[][])
                          n651 = Index Array(array=w1530, index (row) #1=4 ("索引 (行)"), index (row) #2=5 ("索引 (行)"), index (row) #3=6 ("索引 (行)"), index (row) #4=7 ("索引 (行)")) -> (element #1=w1538:string[], element #2=w1537:string[], element #3=w1536:string[], element #4=w1535:string[])  [unwired: 4 in]
                          n652 = Index Array(array=w1537, index=1 ("索引")) -> (element=w1533:string)
                          n653 = Index Array(array=w1538, index=1 ("索引")) -> (element=w1534:string)
                          n654 = Index Array(array=w1536, index=1 ("索引")) -> (element=w1532:string)
                          n655 = Index Array(array=w1535, index=1 ("索引")) -> (element=w1531:string)
                          n656 = Fract/Exp String To Number(string=w1533) -> (number=w1520:dbl)  [unwired: 3 in, 1 out]
                          n657 = Fract/Exp String To Number(string=w1532) -> (number=w1519:dbl)  [unwired: 3 in, 1 out]
                          n658 = Fract/Exp String To Number(string=w1534) -> (number=w1521:dbl)  [unwired: 3 in, 1 out]
                          n659 = Fract/Exp String To Number(string=w1531) -> (number=w1518:dbl)  [unwired: 3 in, 1 out]
                          n660 = Build Array(w1521, w1521, w1520, w1520, w1521) -> (w1540:dbl[])
                          n661 = Build Array(w1518, w1519, w1519, w1518, w1518) -> (w1541:dbl[])
                          n662 = Bundle(w1540, w1541) -> (w1539:cluster{dbl[], dbl[]})  [unwired: 1 in]
                        }
                      }
                    }
                    n663 = local write "力位移曲线 4"(w1513) -> ()
                  }
                }
              }
              frame 1001 {
                n664 = stacked-sequence {
                  frame #0 {
                    n665 = local write "字符串"("0" ("字符串")) -> ()
                    n666 = local read "code 2"() -> (w1544:string)
                    n667 = String Length(string=w1544) -> (length=w1546:i32)
                    n668 = Greater Or Equal?(x=w1546, y=3) -> (x >= y?=w1545:bool)
                    n669 = case shown="真" w1545 {
                      frame False {
                      }
                      frame True {
                        n670 = shared-variable "我的电脑\\Modbus.lvlib\\左工位状态"(u16 1003 ("左工位状态")) -> ()  [unwired: 1 in, 1 out]
                        n671 = local read "code 2"() -> (w1548:string)
                        n672 = Concatenate Strings(w1548) -> (w1549:string)
                        n673 = local write "左工位追溯码"(w1549) -> ()
                        n674 = shared-variable "我的电脑\\Global.lvlib\\工位追溯码"(w1549) -> ()  [unwired: 1 in, 1 out]
                      }
                    }
                  }
                  frame #1 {
                    n675 = global read "Global1.vi" "联机模式"() -> (w1550:enum16{"单机", "追溯"})
                    n676 = case shown="\"追溯\"" w1550 {
                      selector: w1550 -> [_ w1552]
                      frame "单机", Default {
                      }
                      frame "追溯" {
                        n677 = shared-variable "我的电脑\\Global.lvlib\\工位追溯码"() -> ()  [unwired: 1 in, 2 out]
                        n678 = local read "左工位追溯码"() -> (w1551:string)
                        n679 = local read "PRODUCTID"() -> (w1553:string)
                        n680 = call "GetSQLstring.vi"("联机模式"=w1552) -> ("错误输出"=w1558:errorcluster, "连接字符串"=w1559:string)  [unwired: 9 in]
                        n681 = Bundle("左工位追溯码"=w1551, "PRODUCTID"=w1553) -> (w1555:cluster{"左工位追溯码":string, "PRODUCTID":string})  [unwired: 1 in]
                        n682 = call-poly <vilib>:"DB Tools Open Connection.vi"("error in (no error)"=w1558, "connection information"=w1559) -> ("error out"=w1560:errorcluster, "connection reference"=w1557:T15)  [unwired: 6 in]
                        n683 = Build Array(w1555) -> (w1554:cluster{"左工位追溯码":string, "PRODUCTID":string}[])
                        n684 = for {
                          tunnel: w1554 -> [w1565] mode=indexing
                          tunnel: w1557 -> [w1564]
                          shift-right: [w1562] -> w1556
                          shift-left: w1560 -> [w1568]
                          w1561 = string[] ["CODE_SENSOR", "PRODUCT_ID"] ("columns")
                          w1566 = "Code" ("table")
                          n685 = call <vilib>:"DB Tools Insert Data.vi"("data"=w1565, "error in (no error)"=w1568, "columns"=w1561, "table"=w1566, "connection reference"=w1564) -> ("error out"=w1567:errorcluster, "connection reference out"=w1563:T15)  [unwired: 5 in]
                          n686 = case shown="错误" w1567 {
                            selector: w1567 -> [w1569 w1572]
                            tunnel: w1561 -> [_ _]
                            tunnel: w1563 -> [w1570 w1573]
                            tunnel: w1566 -> [_ _]
                            tunnel: w1565 -> [_ _]
                            tunnel: [w1570 w1573] -> _
                            tunnel: [w1569 w1571] -> w1562
                            frame No Error {
                            }
                            frame Error {
                              n687 = call <vilib>:"Clear Errors.vi"("error in (no error)"=w1572) -> ("error out"=w1571:errorcluster)  [unwired: 5 in, 1 out]
                            }
                          }
                        }
                        n688 = call <vilib>:"Simple Error Handler.vi"("error in (no error)"=w1556) -> ()  [unwired: 4 in, 5 out]
                      }
                    }
                  }
                  frame #2 {
                    n689 = global read "Global1.vi" "联机模式"() -> (w1574:enum16{"单机", "追溯"})
                    n690 = case shown="\"追溯\"" w1574 {
                      tunnel: w1574 -> [_ w1596]
                      frame "单机", Default {
                      }
                      frame "追溯" {
                        n691 = local read "左工位追溯码"() -> (w1575:string)
                        n692 = local read "PRODUCTID"() -> (w1579:string)
                        n693 = call "GetSQLstring.vi"("联机模式"=w1596) -> ("错误输出"=w1594:errorcluster, "连接字符串"=w1595:string)  [unwired: 9 in]
                        n694 = call-poly <vilib>:"DB Tools Open Connection.vi"("error in (no error)"=w1594, "connection information"=w1595) -> ("error out"=w1587:errorcluster, "connection reference"=w1588:T15)  [unwired: 6 in]
                        n695 = Concatenate Strings("SELECT CODE_ID FROM CODE  WHERE CODE_SENSOR = '" ("table"), w1575, "'" ("字符串"), " AND PRODUCT_ID='" ("字符串"), w1579, "'" ("字符串")) -> (w1593:string)
                        n696 = call-poly <vilib>:"DB Tools Execute Query.vi"("error in (no error)"=w1587, "SQL query"=w1593, "connection reference"=w1588) -> ("error out"=w1591:errorcluster, "recordset reference"=w1592:T34)  [unwired: 5 in]
                        n697 = call-poly <vilib>:"DB Tools Fetch Recordset Data.vi"("error in (no error)"=w1591, "recordset reference"=w1592) -> ("error out"=w1585:errorcluster, "recordset data"=w1590:variant[][])  [unwired: 3 in, 1 out]
                        n698 = Variant To Data(error in=w1585, type=string[][] [], Variant=w1590) -> (data=w1584:string[][])  [unwired: 1 out]
                        n699 = Index Array(array=w1584, index (row)=0 ("索引 (行)")) -> (element=w1582:string[])  [unwired: 1 in]
                        n700 = Index Array(array=w1582, index=0 ("索引 (行)")) -> (element=w1578:string)
                        n701 = local write "LEFTCODEID"(w1578) -> ()
                      }
                    }
                  }
                }
              }
              frame 1002 {
                n702 = stacked-sequence {
                  frame #0 {
                    n703 = local read "code 3"() -> (w1598:string)
                    n704 = String Length(string=w1598) -> (length=w1600:i32)
                    n705 = Greater Or Equal?(x=w1600, y=3) -> (x >= y?=w1599:bool)
                    n706 = case shown="真" w1599 {
                      frame False {
                      }
                      frame True {
                        n707 = shared-variable "我的电脑\\Modbus.lvlib\\左工位状态"(u16 1003 ("左工位状态")) -> ()  [unwired: 1 in, 1 out]
                        n708 = local read "code 3"() -> (w1601:string)
                        n709 = Concatenate Strings(w1601) -> (w1603:string)
                        n710 = local write "左工位追溯码"(w1603) -> ()
                        n711 = shared-variable "我的电脑\\Global.lvlib\\工位追溯码"(w1603) -> ()  [unwired: 1 in, 1 out]
                      }
                    }
                  }
                  frame #1 {
                    n712 = global read "Global1.vi" "联机模式"() -> (w1604:enum16{"单机", "追溯"})
                    n713 = case shown="\"追溯\"" w1604 {
                      tunnel: w1604 -> [_ w1606]
                      frame "单机", Default {
                      }
                      frame "追溯" {
                        n714 = shared-variable "我的电脑\\Global.lvlib\\工位追溯码"() -> ()  [unwired: 1 in, 2 out]
                        n715 = local read "左工位追溯码"() -> (w1605:string)
                        n716 = local read "PRODUCTID"() -> (w1607:string)
                        n717 = Bundle("左工位追溯码"=w1605, "PRODUCTID"=w1607) -> (w1609:cluster{"左工位追溯码":string, "PRODUCTID":string})  [unwired: 1 in]
                        n718 = call "GetSQLstring.vi"("联机模式"=w1606) -> ("错误输出"=w1612:errorcluster, "连接字符串"=w1613:string)  [unwired: 9 in]
                        n719 = call-poly <vilib>:"DB Tools Open Connection.vi"("error in (no error)"=w1612, "connection information"=w1613) -> ("error out"=w1614:errorcluster, "connection reference"=w1611:T15)  [unwired: 6 in]
                        n720 = Build Array(w1609) -> (w1608:cluster{"左工位追溯码":string, "PRODUCTID":string}[])
                        n721 = for {
                          tunnel: w1608 -> [w1619] mode=indexing
                          tunnel: w1611 -> [w1618]
                          shift-right: [w1616] -> w1610
                          shift-left: w1614 -> [w1622]
                          w1615 = string[] ["CODE_SENSOR", "PRODUCT_ID"] ("columns")
                          w1620 = "Code" ("table")
                          n722 = call <vilib>:"DB Tools Insert Data.vi"("data"=w1619, "error in (no error)"=w1622, "columns"=w1615, "table"=w1620, "connection reference"=w1618) -> ("error out"=w1621:errorcluster, "connection reference out"=w1617:T15)  [unwired: 5 in]
                          n723 = case shown="错误" w1621 {
                            selector: w1621 -> [w1623 w1626]
                            tunnel: w1615 -> [_ _]
                            tunnel: w1617 -> [w1624 w1627]
                            tunnel: w1620 -> [_ _]
                            tunnel: w1619 -> [_ _]
                            tunnel: [w1624 w1627] -> _
                            tunnel: [w1623 w1625] -> w1616
                            frame No Error {
                            }
                            frame Error {
                              n724 = call <vilib>:"Clear Errors.vi"("error in (no error)"=w1626) -> ("error out"=w1625:errorcluster)  [unwired: 5 in, 1 out]
                            }
                          }
                        }
                        n725 = call <vilib>:"Simple Error Handler.vi"("error in (no error)"=w1610) -> ()  [unwired: 4 in, 5 out]
                      }
                    }
                  }
                  frame #2 {
                    n726 = global read "Global1.vi" "联机模式"() -> (w1628:enum16{"单机", "追溯"})
                    n727 = case shown="\"追溯\"" w1628 {
                      tunnel: w1628 -> [_ w1650]
                      frame "单机", Default {
                      }
                      frame "追溯" {
                        n728 = shared-variable "我的电脑\\Global.lvlib\\工位追溯码"() -> ()  [unwired: 1 in, 2 out]
                        n729 = local read "左工位追溯码"() -> (w1629:string)
                        n730 = local read "PRODUCTID"() -> (w1633:string)
                        n731 = call "GetSQLstring.vi"("联机模式"=w1650) -> ("错误输出"=w1648:errorcluster, "连接字符串"=w1649:string)  [unwired: 9 in]
                        n732 = call-poly <vilib>:"DB Tools Open Connection.vi"("error in (no error)"=w1648, "connection information"=w1649) -> ("error out"=w1641:errorcluster, "connection reference"=w1642:T15)  [unwired: 6 in]
                        n733 = Concatenate Strings("SELECT CODE_ID FROM CODE  WHERE CODE_SENSOR = '" ("table"), w1629, "'" ("字符串"), " AND PRODUCT_ID='" ("字符串"), w1633, "'" ("字符串")) -> (w1647:string)
                        n734 = call-poly <vilib>:"DB Tools Execute Query.vi"("error in (no error)"=w1641, "SQL query"=w1647, "connection reference"=w1642) -> ("error out"=w1645:errorcluster, "recordset reference"=w1646:T34)  [unwired: 5 in]
                        n735 = call-poly <vilib>:"DB Tools Fetch Recordset Data.vi"("error in (no error)"=w1645, "recordset reference"=w1646) -> ("error out"=w1639:errorcluster, "recordset data"=w1644:variant[][])  [unwired: 3 in, 1 out]
                        n736 = Variant To Data(error in=w1639, type=string[][] [], Variant=w1644) -> (data=w1638:string[][])  [unwired: 1 out]
                        n737 = Index Array(array=w1638, index (row)=0 ("索引 (行)")) -> (element=w1636:string[])  [unwired: 1 in]
                        n738 = Index Array(array=w1636, index=0 ("索引 (行)")) -> (element=w1632:string)
                        n739 = local write "LEFTCODEID"(w1632) -> ()
                      }
                    }
                  }
                }
              }
            }
            n740 = property on="属性节点" class="CmbBox"(reference=w208, "Strings[]"=w210) -> ()  [unwired: 1 in, 2 out]
            n741 = property on="属性节点" class="CmbBox"(reference=w209, "Strings[]"=w210) -> ()  [unwired: 1 in, 2 out]
            n742 = case shown="1002" w203 {
              frame 0, Default {
              }
              frame 1000 {
                n743 = stacked-sequence {
                  frame #0 {
                    w1653 = "" ("传感器码")
                    n744 = Wait (ms)(milliseconds to wait=u32 300 ("等待时间（毫秒）")) -> ()  [unwired: 1 out]
                    n745 = shared-variable "我的电脑\\Modbus.lvlib\\跳转步骤"(u16 1001 ("跳转步骤")) -> ()  [unwired: 1 in, 1 out]
                    n746 = shared-variable "我的电脑\\Global.lvlib\\传感器码"(w1653) -> ()  [unwired: 1 in, 1 out]
                    n747 = local write "code 2"(w1653) -> ()
                    n748 = local write "左工位追溯码"(w1653) -> ()
                    n749 = local write "右工位追溯码"(w1653) -> ()
                  }
                  frame #1 {
                    w1655 = "请扫码！" ("通知内容")
                    n750 = call "浮动通知.vi"("通知内容"=w1655) -> ()  [unwired: 11 in]
                    n751 = call "输入框.vi"("提示信息"=w1655) -> ("条形码输出"=w1654:string)
                    "code 2" <- w1654
                    n752 = shared-variable "我的电脑\\Global.lvlib\\传感器码"(w1654) -> ()  [unwired: 1 in, 1 out]
                  }
                }
              }
              frame 1001 {
                n753 = stacked-sequence {
                  frame #0 {
                    n754 = Wait (ms)(milliseconds to wait=u32 500 ("等待时间（毫秒）")) -> ()  [unwired: 1 out]
                  }
                  frame #1 {
                    n755 = shared-variable "我的电脑\\Modbus.lvlib\\左工位工件在位"() -> (w1658:u16)  [unwired: 1 in, 1 out]
                    n756 = shared-variable "我的电脑\\Modbus.lvlib\\右工位工件在位"() -> (w1657:u16)  [unwired: 1 in, 1 out]
                    n757 = case shown="1" w1658 {
                      frame 0, Default {
                      }
                      frame 1 {
                        n758 = shared-variable "我的电脑\\Modbus.lvlib\\左工位工件在位"(u16 0 ("左工位工件在位")) -> ()  [unwired: 1 in, 1 out]
                        n759 = shared-variable "我的电脑\\Modbus.lvlib\\左工位状态"(u16 1001 ("左工位状态")) -> ()  [unwired: 1 in, 1 out]
                      }
                    }
                    n760 = case shown="1" w1657 {
                      frame 0, Default {
                      }
                      frame 1 {
                        n761 = shared-variable "我的电脑\\Modbus.lvlib\\右工位工件在位"(u16 0 ("右工位工件在位")) -> ()  [unwired: 1 in, 1 out]
                        n762 = shared-variable "我的电脑\\Modbus.lvlib\\右工位状态"(u16 1001 ("左工位状态")) -> ()  [unwired: 1 in, 1 out]
                      }
                    }
                  }
                }
              }
              frame 1002 {
                n763 = stacked-sequence {
                  frame #0 {
                    w1665 = "" ("传感器码")
                    n764 = Wait (ms)(milliseconds to wait=u32 300 ("等待时间（毫秒）")) -> ()  [unwired: 1 out]
                    n765 = shared-variable "我的电脑\\Modbus.lvlib\\跳转步骤"(u16 1003 ("跳转步骤")) -> ()  [unwired: 1 in, 1 out]
                    n766 = shared-variable "我的电脑\\Global.lvlib\\传感器码"(w1665) -> ()  [unwired: 1 in, 1 out]
                    n767 = local write "code 3"(w1665) -> ()
                  }
                  frame #1 {
                    w1667 = "请扫码！" ("通知内容")
                    n768 = call "浮动通知.vi"("通知内容"=w1667) -> ()  [unwired: 11 in]
                    n769 = call "输入框.vi"("提示信息"=w1667) -> ("条形码输出"=w1666:string)
                    "code 3" <- w1666
                    n770 = shared-variable "我的电脑\\Global.lvlib\\传感器码"(w1666) -> ()  [unwired: 1 in, 1 out]
                  }
                }
              }
              frame 1003 {
                n771 = stacked-sequence {
                  frame #0 {
                    n772 = Wait (ms)(milliseconds to wait=u32 500 ("等待时间（毫秒）")) -> ()  [unwired: 1 out]
                  }
                  frame #1 {
                    n773 = shared-variable "我的电脑\\Modbus.lvlib\\左工位工件在位"() -> (w1670:u16)  [unwired: 1 in, 1 out]
                    n774 = shared-variable "我的电脑\\Modbus.lvlib\\右工位工件在位"() -> (w1669:u16)  [unwired: 1 in, 1 out]
                    n775 = case shown="1" w1670 {
                      frame 0, Default {
                      }
                      frame 1 {
                        n776 = shared-variable "我的电脑\\Modbus.lvlib\\左工位工件在位"(u16 0 ("左工位工件在位")) -> ()  [unwired: 1 in, 1 out]
                        n777 = shared-variable "我的电脑\\Modbus.lvlib\\左工位状态"(u16 1002 ("左工位状态")) -> ()  [unwired: 1 in, 1 out]
                      }
                    }
                    n778 = case shown="1" w1669 {
                      frame 0, Default {
                      }
                      frame 1 {
                        n779 = shared-variable "我的电脑\\Modbus.lvlib\\右工位工件在位"(u16 0 ("右工位工件在位")) -> ()  [unwired: 1 in, 1 out]
                        n780 = shared-variable "我的电脑\\Modbus.lvlib\\右工位状态"(u16 1002 ("左工位状态")) -> ()  [unwired: 1 in, 1 out]
                      }
                    }
                  }
                }
              }
            }
            n781 = case shown="1001" w205 {
              frame 0, Default {
              }
              frame 500 {
                n782 = local read "力位移曲线 3"() -> (w534:cluster{dbl[], dbl[]}[])
                n783 = for {
                  tunnel: [w538] -> w535 mode=indexing
                  tunnel: w534 -> [w537] mode=indexing
                  i -> [w536]
                  n784 = case shown="2" w536 {
                    tunnel: [w539 w553] -> w538
                    tunnel: w537 -> [w539 w552]
                    frame Default {
                    }
                    frame 2 {
                      n785 = shared-variable "我的电脑\\Modbus.lvlib\\编码器位移"() -> ()  [unwired: 1 in, 2 out]
                      n786 = local write "Initialize 3"(FALSE ("Initialize 2")) -> ()
                      n787 = local read "右空载系数"() -> (w548:dbl)
                      n788 = global read "全局2.vi" "右加载"() -> (w544:dbl)
                      n789 = global read "Global.vi" "空载速度(°/s)"() -> (w540:dbl)
                      n790 = case shown="真" "Initialize 3" {
                        tunnel: [w558 0.0] -> w542
                        frame False {
                          n791 = global read "全局 1.vi" "工位1正向磨合开始时间"() -> (w559:u32)
                          n792 = Tick Count (ms)() -> (millisecond timer value=w562:u32)
                          n793 = Subtract(x=w562, y=w559) -> (x-y=w561:u32)
                          n794 = Divide(x=w561, y=u32 1000) -> (x/y=w558:dbl)
                          n795 = global write "全局 1.vi" "工位1正向磨合结束时间"(w558) -> ()
                        }
                        frame True {
                          n796 = Tick Count (ms)() -> (millisecond timer value=w564:u32)
                          n797 = global write "全局 1.vi" "工位1正向磨合开始时间"(w564) -> ()
                        }
                      }
                      n798 = Subtract(x=w544, y=0.0) -> (x-y=w547:dbl)
                      n799 = shared-variable "我的电脑\\Modbus.lvlib\\加载传感器偏移值"() -> (w551:sgl[])  [unwired: 1 in, 1 out]
                      n800 = Multiply(x=w547, y=w548) -> (x*y=w546:dbl)
                      n801 = Unbundle(w552) -> (w557:dbl[], w556:dbl[])
                      n802 = Build Array (concatenate)(w556, w546) -> (w554:dbl[])
                      n803 = Index Array(array=w551, index=2) -> ()  [unwired: 1 out]
                      n804 = Multiply(x=w540, y=w542) -> (x*y=w541:dbl)
                      n805 = Build Array (concatenate)(w557, w541) -> (w555:dbl[])
                      n806 = Bundle(w555, w554) -> (w553:cluster{dbl[], dbl[]})  [unwired: 1 in]
                    }
                  }
                }
                n807 = local write "力位移曲线 3"(w535) -> ()
              }
              frame 600 {
                n808 = local read "力位移曲线 3"() -> (w565:cluster{dbl[], dbl[]}[])
                n809 = for {
                  tunnel: [w569] -> w566 mode=indexing
                  tunnel: w565 -> [w568] mode=indexing
                  i -> [w567]
                  n810 = case shown="3" w567 {
                    tunnel: [w570 w585] -> w569
                    tunnel: w568 -> [w570 w584]
                    frame Default {
                    }
                    frame 3 {
                      n811 = local write "Initialize 5"(FALSE ("Initialize 5")) -> ()
                      n812 = local read "右逆向空载"() -> (w571:dbl)
                      n813 = global read "全局2.vi" "右加载"() -> (w576:dbl)
                      n814 = shared-variable "我的电脑\\Modbus.lvlib\\编码器位移"() -> (w583:sgl[])  [unwired: 1 in, 1 out]
                      n815 = global read "Global.vi" "空载速度(°/s)"() -> (w572:dbl)
                      n816 = case shown="假" "Initialize 5" {
                        tunnel: [w591 w598] -> w574
                        frame False {
                          n817 = global read "全局 1.vi" "工位1正向磨合结束时间"() -> (w593:dbl)
                          n818 = global read "全局 1.vi" "工位1逆向磨合开始时间"() -> (w594:u32)
                          n819 = Tick Count (ms)() -> (millisecond timer value=w597:u32)
                          n820 = Subtract(x=w597, y=w594) -> (x-y=w596:u32)
                          n821 = Divide(x=w596, y=u32 1000) -> (x/y=w592:dbl)
                          n822 = Subtract(x=w593, y=w592) -> (x-y=w591:dbl)
                        }
                        frame True {
                          n823 = Tick Count (ms)() -> (millisecond timer value=w599:u32)
                          n824 = global write "全局 1.vi" "工位1逆向磨合开始时间"(w599) -> ()
                          n825 = global read "全局 1.vi" "工位1正向磨合结束时间"() -> (w598:dbl)
                        }
                      }
                      n826 = Subtract(x=w576, y=0.0) -> (x-y=w579:dbl)
                      n827 = shared-variable "我的电脑\\Modbus.lvlib\\加载传感器偏移值"() -> (w582:sgl[])  [unwired: 1 in, 1 out]
                      n828 = Multiply(x=w579, y=w571) -> (x*y=w578:dbl)
                      n829 = Unbundle(w584) -> (w589:dbl[], w588:dbl[])
                      n830 = Index Array(array=w583, index=4) -> ()  [unwired: 1 out]
                      n831 = Build Array (concatenate)(w588, w578) -> (w586:dbl[])
                      n832 = Index Array(array=w582, index=3) -> ()  [unwired: 1 out]
                      n833 = Multiply(x=w572, y=w574) -> (x*y=w573:dbl)
                      n834 = Build Array (concatenate)(w589, w573) -> (w587:dbl[])
                      n835 = Bundle(w587, w586) -> (w585:cluster{dbl[], dbl[]})  [unwired: 1 in]
                    }
                  }
                }
                n836 = local write "力位移曲线 3"(w566) -> ()
              }
              frame 700 {
                n837 = local read "右扭矩波动"() -> (w608:dbl)
                n838 = local read "判定框参数"() -> (w636:string[][])
                n839 = local read "右平均扭矩系数"() -> (w613:dbl)
                n840 = local read "力位移曲线 3"() -> (w664:cluster{dbl[], dbl[]}[])
                n841 = local read "力位移曲线 3"() -> (w657:cluster{dbl[], dbl[]}[])
                n842 = Index Array(array=w636, index (row) #1=1 ("索引 (行)"), index (row) #2=0 ("索引 (行)"), index (row) #3=5 ("索引 (行)"), index (row) #4=4 ("索引 (行)")) -> (element #1=w628:string[], element #2=w629:string[], element #3=w630:string[], element #4=w631:string[])  [unwired: 4 in]
                n843 = Index Array(array=w657) -> (element #4=w651:cluster{dbl[], dbl[]})  [unwired: 4 in, 3 out]
                n844 = Index Array(array=w664) -> (element #3=w652:cluster{dbl[], dbl[]})  [unwired: 4 in, 3 out]
                n845 = Unbundle ("解除捆绑")(w651) -> (w645:dbl[], w647:dbl[])
                n846 = Index Array(array=w629, index=1 ("索引")) -> (element=w633:string)
                n847 = Index Array(array=w628, index=1 ("索引")) -> (element=w632:string)
                n848 = Index Array(array=w631, index=1 ("索引")) -> (element=w635:string)
                n849 = Index Array(array=w630, index=1 ("索引")) -> (element=w634:string)
                n850 = Fract/Exp String To Number(string=w633) -> (number=w625:dbl)  [unwired: 3 in, 1 out]
                n851 = Fract/Exp String To Number(string=w632) -> (number=w624:dbl)  [unwired: 3 in, 1 out]
                n852 = Fract/Exp String To Number(string=w635) -> (number=w627:dbl)  [unwired: 3 in, 1 out]
                n853 = Fract/Exp String To Number(string=w634) -> (number=w626:dbl)  [unwired: 3 in, 1 out]
                n854 = Unbundle(w652) -> (w662:dbl[], w663:dbl[])
                n855 = Reverse 1D Array(array=w645) -> (reversed array=w646:dbl[])
                n856 = Threshold 1D Array(2:w625, 3:w662) -> (0:w661:dbl)  [unwired: 1 in]
                n857 = Threshold 1D Array(2:w627, 3:w646) -> (0:w656:dbl)  [unwired: 1 in]
                n858 = Reverse 1D Array(array=w647) -> (reversed array=w648:dbl[])
                n859 = Split 1D Array(array=w663, index=w661) -> (second subarray=w660:dbl[])  [unwired: 1 out]
                n860 = Split 1D Array(array=w648, index=w656) -> (second subarray=w655:dbl[])  [unwired: 1 out]
                n861 = Split 1D Array(array=w662, index=w661) -> (second subarray=w659:dbl[])  [unwired: 1 out]
                n862 = Split 1D Array(array=w646, index=w656) -> (second subarray=w654:dbl[])  [unwired: 1 out]
                n863 = Threshold 1D Array(2:w624, 3:w659) -> (0:w658:dbl)  [unwired: 1 in]
                n864 = Threshold 1D Array(2:w626, 3:w654) -> (0:w653:dbl)  [unwired: 1 in]
                n865 = Split 1D Array(array=w659, index=w658) -> ()  [unwired: 2 out]
                n866 = Split 1D Array(array=w654, index=w653) -> ()  [unwired: 2 out]
                n867 = Split 1D Array(array=w660, index=w658) -> (first subarray=w650:dbl[])  [unwired: 1 out]
                n868 = Split 1D Array(array=w655, index=w653) -> (first subarray=w649:dbl[])  [unwired: 1 out]
                n869 = call-poly <vilib>:"Mean.vi"("X"=w650) -> ("mean"=w641:dbl)  [unwired: 1 out]
                n870 = call-poly <vilib>:"Mean.vi"("X"=w649) -> ("mean"=w637:dbl)  [unwired: 1 out]
                n871 = Array Max & Min(array=w650) -> (max value=w607:dbl, min value=w606:dbl)  [unwired: 2 out]
                n872 = Array Max & Min(array=w649) -> (max value=w605:dbl, min value=w604:dbl)  [unwired: 2 out]
                n873 = Subtract(x=w607, y=w606) -> (x-y=w642:dbl)
                n874 = Subtract(x=w605, y=w604) -> (x-y=w639:dbl)
                n875 = Absolute Value(x=w607) -> (abs(x)=→"右工位正向最大扭矩(Nm)":dbl)
                n876 = Absolute Value(x=w606) -> (abs(x)=→"右工位正向最小扭矩(Nm)":dbl)
                n877 = Absolute Value(x=w641) -> (abs(x)=w615:dbl)
                n878 = Absolute Value(x=w637) -> (abs(x)=w614:dbl)
                n879 = Absolute Value(x=w605) -> (abs(x)=→"右工位逆向最小扭矩(Nm)":dbl)
                n880 = Absolute Value(x=w604) -> (abs(x)=→"右工位逆向最大扭矩(Nm)":dbl)
                n881 = Multiply(x=w615, y=w613) -> (x*y=w603:dbl)
                "右工位正向平均扭矩(Nm)" <- w603
                n882 = Multiply(x=w614, y=w613) -> (x*y=w602:dbl)
                "右工位逆向平均扭矩(Nm)" <- w602
                n883 = Subtract(x=w603, y=w602) -> (x-y=w601:dbl)
                n884 = Absolute Value(x=w601) -> (abs(x)=→"右工位正逆平均扭矩差(Nm)":dbl)
                n885 = Absolute Value(x=w642) -> (abs(x)=w612:dbl)
                n886 = Absolute Value(x=w639) -> (abs(x)=w610:dbl)
                n887 = Multiply(x=w612, y=w608) -> (x*y=→"右工位正向波动扭矩(Nm)":dbl)
                n888 = Multiply(x=w610, y=w608) -> (x*y=→"右工位逆向波动扭矩(Nm)":dbl)
              }
              frame 1 {
                n889 = stacked-sequence {
                  frame #0 {
                    n890 = Wait (ms)(milliseconds to wait=u32 200 ("等待时间（毫秒）")) -> ()  [unwired: 1 out]
                    n891 = control-ref of="力位移曲线 3"() -> (w696:refnum<vi>)
                    n892 = local read "结果判定参数"() -> (w720:string[][])
                    n893 = local read "右工位正逆平均扭矩差(Nm)"() -> (w669:dbl)
                    n894 = global write "A131258.vi" "右工位空载曲线 2"(w696) -> ()
                    n895 = local read "右工位正向最大扭矩(Nm)"() -> (w758:dbl)
                    n896 = local read "右工位正向波动扭矩(Nm)"() -> (w755:dbl)
                    n897 = local read "右工位正向平均扭矩(Nm)"() -> (w752:dbl)
                    n898 = local read "右工位逆向最大扭矩(Nm)"() -> (w749:dbl)
                    n899 = local read "右工位逆向波动扭矩(Nm)"() -> (w746:dbl)
                    n900 = local read "右工位逆向平均扭矩(Nm)"() -> (w743:dbl)
                    n901 = local read "右工位正向最小扭矩(Nm)"() -> (w683:dbl)
                    n902 = local read "右工位逆向最小扭矩(Nm)"() -> (w681:dbl)
                    n903 = Index Array(array=w720, index (row) #1=0 ("索引 (行)"), index (row) #2=0 ("索引 (行)"), index (row) #3=1 ("索引 (行)"), index (row) #4=1 ("索引 (行)"), index (row) #5=2 ("索引 (行)"), index (row) #6=2 ("索引 (行)"), index (row) #7=3 ("索引 (行)"), index (row) #8=4 ("索引 (行)")) -> (element #1=w727:string[], element #2=w726:string[], element #3=w725:string[], element #4=w724:string[], element #5=w717:string[], element #6=w716:string[], element #7=w690:string[], element #8=w674:string[])  [unwired: 8 in]
                    n904 = Index Array(array=w674, index #1=1 ("索引"), index #2=2 ("索引")) -> (element #1=w673:string, element #2=w671:string)
                    n905 = Index Array(array=w727, index=1 ("索引")) -> (element=w703:string)
                    n906 = Index Array(array=w726, index=2 ("索引")) -> (element=w723:string)
                    n907 = Index Array(array=w725, index=1 ("索引")) -> (element=w722:string)
                    n908 = Index Array(array=w724, index=2 ("索引")) -> (element=w721:string)
                    n909 = Index Array(array=w717, index=1 ("索引")) -> (element=w719:string)
                    n910 = Index Array(array=w716, index=2 ("索引")) -> (element=w718:string)
                    n911 = Index Array(array=w690, index #1=2 ("索引"), index #2=1 ("索引")) -> (element #1=w691:string, element #2=w684:string)
                    n912 = Fract/Exp String To Number(string=w673) -> (number=w672:dbl)  [unwired: 3 in, 1 out]
                    n913 = Fract/Exp String To Number(string=w671) -> (number=w670:dbl)  [unwired: 3 in, 1 out]
                    n914 = Fract/Exp String To Number(string=w703) -> (number=w710:dbl)  [unwired: 3 in, 1 out]
                    n915 = Fract/Exp String To Number(string=w723) -> (number=w715:dbl)  [unwired: 3 in, 1 out]
                    n916 = Fract/Exp String To Number(string=w722) -> (number=w714:dbl)  [unwired: 3 in, 1 out]
                    n917 = Fract/Exp String To Number(string=w721) -> (number=w713:dbl)  [unwired: 3 in, 1 out]
                    n918 = Fract/Exp String To Number(string=w719) -> (number=w712:dbl)  [unwired: 3 in, 1 out]
                    n919 = Fract/Exp String To Number(string=w718) -> (number=w711:dbl)  [unwired: 3 in, 1 out]
                    n920 = Fract/Exp String To Number(string=w684) -> (number=w680:dbl)  [unwired: 3 in, 1 out]
                    n921 = Fract/Exp String To Number(string=w691) -> (number=w679:dbl)  [unwired: 3 in, 1 out]
                    n922 = In Range and Coerce(upper limit=w672, x=w669, lower limit=w670) -> (In Range?=w666:bool)  [unwired: 1 out]
                    n923 = Greater Or Equal?(x=w710, y=w758) -> (x >= y?=w757:bool)
                    n924 = Greater Or Equal?(x=w758, y=w715) -> (x >= y?=w756:bool)
                    n925 = Greater Or Equal?(x=w714, y=w755) -> (x >= y?=w754:bool)
                    n926 = Greater Or Equal?(x=w755, y=w713) -> (x >= y?=w753:bool)
                    n927 = Greater Or Equal?(x=w712, y=w752) -> (x >= y?=w751:bool)
                    n928 = Greater Or Equal?(x=w752, y=w711) -> (x >= y?=w750:bool)
                    n929 = Greater Or Equal?(x=w710, y=w749) -> (x >= y?=w748:bool)
                    n930 = Greater Or Equal?(x=w749, y=w715) -> (x >= y?=w747:bool)
                    n931 = Greater Or Equal?(x=w714, y=w746) -> (x >= y?=w745:bool)
                    n932 = Greater Or Equal?(x=w746, y=w713) -> (x >= y?=w744:bool)
                    n933 = Greater Or Equal?(x=w712, y=w743) -> (x >= y?=w742:bool)
                    n934 = Greater Or Equal?(x=w743, y=w711) -> (x >= y?=w741:bool)
                    n935 = In Range and Coerce(upper limit=w680, x=w683, lower limit=w679) -> (In Range?=w682:bool)  [unwired: 1 out]
                    n936 = In Range and Coerce(upper limit=w680, x=w681, lower limit=w679) -> (In Range?=w678:bool)  [unwired: 1 out]
                    n937 = case shown="真" w682 {
                      tunnel: [u32 16711680 u32 56369] -> w689
                      frame False {
                        n938 = local write "右正小结果"("NG" ("LEFTRESULT")) -> ()
                      }
                      frame True {
                        n939 = local write "右正小结果"("OK" ("LEFTRESULT")) -> ()
                      }
                    }
                    n940 = case shown="真" w678 {
                      tunnel: [u32 16711680 u32 56369] -> w688
                      frame False {
                        n941 = local write "右逆小结果"("NG" ("LEFTRESULT")) -> ()
                      }
                      frame True {
                        n942 = local write "右逆小结果"("OK" ("LEFTRESULT")) -> ()
                      }
                    }
                    n943 = case shown="假" w666 {
                      tunnel: [u32 16711680 u32 56369] -> w668
                      frame False {
                        n944 = local write "右平均差"("NG" ("LEFTRESULT")) -> ()
                      }
                      frame True {
                        n945 = local write "右平均差"("OK" ("LEFTRESULT")) -> ()
                      }
                    }
                    n946 = And(x=w682, y=w678) -> (x .and. y?=w686:bool)
                    n947 = And(x=w757, y=w756) -> (x .and. y?=w740:bool)
                    n948 = And(x=w754, y=w753) -> (x .and. y?=w739:bool)
                    n949 = And(x=w751, y=w750) -> (x .and. y?=w731:bool)
                    n950 = And(x=w748, y=w747) -> (x .and. y?=w738:bool)
                    n951 = And(x=w745, y=w744) -> (x .and. y?=w737:bool)
                    n952 = And(x=w742, y=w741) -> (x .and. y?=w736:bool)
                    n953 = case shown="真" w738 {
                      frame False {
                        n954 = local write "右逆大结果"("NG" ("LEFTRESULT")) -> ()
                        n955 = property on="右工位逆向最大扭矩(Nm)" class="DigNum (严格)"("NumText.BGColor"=u32 16711680) -> ()  [unwired: 2 in, 2 out]
                      }
                      frame True {
                        n956 = local write "右逆大结果"("OK" ("LEFTRESULT")) -> ()
                        n957 = property on="右工位逆向最大扭矩(Nm)" class="DigNum (严格)"("NumText.BGColor"=u32 56369) -> ()  [unwired: 2 in, 2 out]
                      }
                    }
                    n958 = case shown="真" w740 {
                      frame False {
                        n959 = local write "右正大结果"("NG" ("LEFTRESULT")) -> ()
                        n960 = property on="右工位正向最大扭矩(Nm)" class="DigNum (严格)"("NumText.BGColor"=u32 16711680) -> ()  [unwired: 2 in, 2 out]
                      }
                      frame True {
                        n961 = local write "右正大结果"("OK" ("LEFTRESULT")) -> ()
                        n962 = property on="右工位正向最大扭矩(Nm)" class="DigNum (严格)"("NumText.BGColor"=u32 56369) -> ()  [unwired: 2 in, 2 out]
                      }
                    }
                    n963 = case shown="真" w739 {
                      frame False {
                        n964 = local write "右正波结果"("NG" ("LEFTRESULT")) -> ()
                        n965 = property on="右工位正向波动扭矩(Nm)" class="DigNum (严格)"("NumText.BGColor"=u32 16711680) -> ()  [unwired: 2 in, 2 out]
                      }
                      frame True {
                        n966 = local write "右正波结果"("OK" ("LEFTRESULT")) -> ()
                        n967 = property on="右工位正向波动扭矩(Nm)" class="DigNum (严格)"("NumText.BGColor"=u32 56369) -> ()  [unwired: 2 in, 2 out]
                      }
                    }
                    n968 = case shown="真" w737 {
                      frame False {
                        n969 = local write "右逆波结果"("NG" ("LEFTRESULT")) -> ()
                        n970 = property on="右工位逆向波动扭矩(Nm)" class="DigNum (严格)"("NumText.BGColor"=u32 16711680) -> ()  [unwired: 2 in, 2 out]
                      }
                      frame True {
                        n971 = local write "右逆波结果"("OK" ("LEFTRESULT")) -> ()
                        n972 = property on="右工位逆向波动扭矩(Nm)" class="DigNum (严格)"("NumText.BGColor"=u32 56369) -> ()  [unwired: 2 in, 2 out]
                      }
                    }
                    n973 = case shown="真" w731 {
                      frame False {
                        n974 = local write "右正平结果"("NG" ("LEFTRESULT")) -> ()
                        n975 = property on="右工位正向平均扭矩(Nm)" class="DigNum (严格)"("NumText.BGColor"=u32 16711680) -> ()  [unwired: 2 in, 2 out]
                      }
                      frame True {
                        n976 = local write "右正平结果"("OK" ("LEFTRESULT")) -> ()
                        n977 = property on="右工位正向平均扭矩(Nm)" class="DigNum (严格)"("NumText.BGColor"=u32 56369) -> ()  [unwired: 2 in, 2 out]
                      }
                    }
                    n978 = case shown="真" w736 {
                      frame False {
                        n979 = local write "右逆平结果"("NG" ("LEFTRESULT")) -> ()
                        n980 = property on="右工位逆向平均扭矩(Nm)" class="DigNum (严格)"("NumText.BGColor"=u32 16711680) -> ()  [unwired: 2 in, 2 out]
                      }
                      frame True {
                        n981 = local write "右逆平结果"("OK" ("LEFTRESULT")) -> ()
                        n982 = property on="右工位逆向平均扭矩(Nm)" class="DigNum (严格)"("NumText.BGColor"=u32 56369) -> ()  [unwired: 2 in, 2 out]
                      }
                    }
                    n983 = And(x=w740, y=w739) -> (x .and. y?=w735:bool)
                    n984 = And(x=w731, y=w738) -> (x .and. y?=w734:bool)
                    n985 = And(x=w737, y=w736) -> (x .and. y?=w732:bool)
                    n986 = And(x=w735, y=w734) -> (x .and. y?=w733:bool)
                    n987 = And(x=w733, y=w732) -> (x .and. y?=w687:bool)
                    n988 = And(x=w687, y=w686) -> (x .and. y?=w667:bool)
                    n989 = And(x=w667, y=w666) -> (x .and. y?=w665:bool)
                    n990 = case shown="假" w665 {
                      tunnel: [u16 2 ("左工位生产结果") u16 1 ("左工位生产结果")] -> w730
                      tunnel: [TRUE ("不合格指示灯") FALSE ("不合格指示灯")] -> w729
                      tunnel: [FALSE ("合格指示灯") TRUE ("合格指示灯")] -> w728
                      tunnel: [bool[][] [[TRUE, FALSE]] ("判定结果") bool[][] [[TRUE, TRUE]] ("判定结果")] -> w694
                      frame False {
                        "RIGHTRESULT" <- "NG" ("LEFTRESULT")
                      }
                      frame True {
                        n991 = local write "RIGHTRESULT"("OK" ("LEFTRESULT")) -> ()
                      }
                    }
                    "不合格指示灯" <- w729
                    "合格指示灯" <- w728
                    n992 = property on="右工位正逆平均扭矩差(Nm)" class="DigNum (严格)"("NumText.BGColor"=w668) -> ()  [unwired: 2 in, 2 out]
                    n993 = property on="右工位正向最小扭矩(Nm)" class="DigNum (严格)"("NumText.BGColor"=w689) -> ()  [unwired: 2 in, 2 out]
                    n994 = property on="右工位逆向最小扭矩(Nm)" class="DigNum (严格)"("NumText.BGColor"=w688) -> ()  [unwired: 2 in, 2 out]
                    n995 = shared-variable "我的电脑\\Modbus.lvlib\\右工位生产结果"(w730) -> ()  [unwired: 1 in, 1 out]
                    n996 = local write "右工位判定结果 4"(w694) -> ()
                  }
                  frame #1 {
                    n997 = stacked-sequence {
                      frame #0 {
                        n998 = Wait (ms)(milliseconds to wait=u32 500 ("等待时间（毫秒）")) -> ()  [unwired: 1 out]
                        n999 = call "浮动通知.vi"("通知内容"="报表生成中" ("Status")) -> ()  [unwired: 11 in]
                      }
                      frame #1 {
                      }
                    }
                    n1000 = local write "字符串"("1" ("字符串")) -> ()
                    n1001 = local read "最小值上限"() -> (w828:dbl)
                    n1002 = local read "最小值下限"() -> (w827:dbl)
                    n1003 = local read "最大值上限"() -> (w851:dbl)
                    n1004 = local read "最大值下限"() -> (w850:dbl)
                    n1005 = local read "波动值上限"() -> (w848:dbl)
                    n1006 = local read "波动值下限"() -> (w847:dbl)
                    n1007 = local read "平均值上限"() -> (w845:dbl)
                    n1008 = local read "平均值下限"() -> (w844:dbl)
                    n1009 = local read "最小值上限"() -> (w819:dbl)
                    n1010 = local read "最小值下限"() -> (w820:dbl)
                    n1011 = local read "最大值上限"() -> (w841:dbl)
                    n1012 = local read "最大值下限"() -> (w840:dbl)
                    n1013 = local read "波动值上限"() -> (w838:dbl)
                    n1014 = local read "波动值下限"() -> (w837:dbl)
                    n1015 = local read "平均值上限"() -> (w835:dbl)
                    n1016 = local read "平均值下限"() -> (w834:dbl)
                    n1017 = control-ref of="右工位报表"() -> (w832:refnum<vi>)
                    n1018 = local read "平均值差上限"() -> (w807:dbl)
                    n1019 = local read "平均值差下限"() -> (w806:dbl)
                    n1020 = global write "Global.vi" "Result  右工位"(w832) -> ()
                    n1021 = local read "右工位正向最小扭矩(Nm)"() -> (w853:dbl)
                    n1022 = local read "右工位正向最大扭矩(Nm)"() -> (w852:dbl)
                    n1023 = local read "右工位正向波动扭矩(Nm)"() -> (w849:dbl)
                    n1024 = local read "右工位正向平均扭矩(Nm)"() -> (w846:dbl)
                    n1025 = local read "右工位逆向最小扭矩(Nm)"() -> (w843:dbl)
                    n1026 = local read "右工位逆向最大扭矩(Nm)"() -> (w842:dbl)
                    n1027 = local read "右工位逆向波动扭矩(Nm)"() -> (w839:dbl)
                    n1028 = local read "右工位逆向平均扭矩(Nm)"() -> (w836:dbl)
                    n1029 = local read "右工位正逆平均扭矩差(Nm)"() -> (w808:dbl)
                    n1030 = Number To Fractional String(number=w808, precision (6)=i16 3 ("精度(6)")) -> (F-format string=w811:string)  [unwired: 2 in]
                    n1031 = Number To Fractional String(number=w807, precision (6)=i16 3 ("精度(6)")) -> (F-format string=w810:string)  [unwired: 2 in]
                    n1032 = Number To Fractional String(number=w806, precision (6)=i16 3 ("精度(6)")) -> (F-format string=w809:string)  [unwired: 2 in]
                    n1033 = Number To Fractional String(number=w853, precision (6)=i16 3 ("精度(6)")) -> (F-format string=w897:string)  [unwired: 2 in]
                    n1034 = Number To Fractional String(number=w828, precision (6)=i16 3 ("精度(6)")) -> (F-format string=w830:string)  [unwired: 2 in]
                    n1035 = Number To Fractional String(number=w827, precision (6)=i16 3 ("精度(6)")) -> (F-format string=w829:string)  [unwired: 2 in]
                    n1036 = Number To Fractional String(number=w852, precision (6)=i16 3 ("精度(6)")) -> (F-format string=w895:string)  [unwired: 2 in]
                    n1037 = Number To Fractional String(number=w851, precision (6)=i16 3 ("精度(6)")) -> (F-format string=w894:string)  [unwired: 2 in]
                    n1038 = Number To Fractional String(number=w850, precision (6)=i16 3 ("精度(6)")) -> (F-format string=w892:string)  [unwired: 2 in]
                    n1039 = Number To Fractional String(number=w849, precision (6)=i16 3 ("精度(6)")) -> (F-format string=w890:string)  [unwired: 2 in]
                    n1040 = Number To Fractional String(number=w848, precision (6)=i16 3 ("精度(6)")) -> (F-format string=w889:string)  [unwired: 2 in]
                    n1041 = Number To Fractional String(number=w847, precision (6)=i16 3 ("精度(6)")) -> (F-format string=w888:string)  [unwired: 2 in]
                    n1042 = Number To Fractional String(number=w846, precision (6)=i16 3 ("精度(6)")) -> (F-format string=w883:string)  [unwired: 2 in]
                    n1043 = Number To Fractional String(number=w845, precision (6)=i16 3 ("精度(6)")) -> (F-format string=w884:string)  [unwired: 2 in]
                    n1044 = Number To Fractional String(number=w844, precision (6)=i16 3 ("精度(6)")) -> (F-format string=w885:string)  [unwired: 2 in]
                    n1045 = Number To Fractional String(number=w843, precision (6)=i16 3 ("精度(6)")) -> (F-format string=w878:string)  [unwired: 2 in]
                    n1046 = Number To Fractional String(number=w819, precision (6)=i16 3 ("精度(6)")) -> (F-format string=w817:string)  [unwired: 2 in]
                    n1047 = Number To Fractional String(number=w820, precision (6)=i16 3 ("精度(6)")) -> (F-format string=w816:string)  [unwired: 2 in]
                    n1048 = Number To Fractional String(number=w842, precision (6)=i16 3 ("精度(6)")) -> (F-format string=w873:string)  [unwired: 2 in]
                    n1049 = Number To Fractional String(number=w841, precision (6)=i16 3 ("精度(6)")) -> (F-format string=w874:string)  [unwired: 2 in]
                    n1050 = Number To Fractional String(number=w840, precision (6)=i16 3 ("精度(6)")) -> (F-format string=w875:string)  [unwired: 2 in]
                    n1051 = Number To Fractional String(number=w839, precision (6)=i16 3 ("精度(6)")) -> (F-format string=w865:string)  [unwired: 2 in]
                    n1052 = Number To Fractional String(number=w838, precision (6)=i16 3 ("精度(6)")) -> (F-format string=w864:string)  [unwired: 2 in]
                    n1053 = Number To Fractional String(number=w837, precision (6)=i16 3 ("精度(6)")) -> (F-format string=w863:string)  [unwired: 2 in]
                    n1054 = Number To Fractional String(number=w836, precision (6)=i16 3 ("精度(6)")) -> (F-format string=w859:string)  [unwired: 2 in]
                    n1055 = Number To Fractional String(number=w835, precision (6)=i16 3 ("精度(6)")) -> (F-format string=w860:string)  [unwired: 2 in]
                    n1056 = Number To Fractional String(number=w834, precision (6)=i16 3 ("精度(6)")) -> (F-format string=w861:string)  [unwired: 2 in]
                    n1057 = Build Array(w811, w810, w809) -> (w805:string[])
                    n1058 = Build Array(w897, w830, w829) -> (w896:string[])
                    n1059 = Build Array(w895, w894, w892) -> (w893:string[])
                    n1060 = Build Array(w890, w889, w888) -> (w891:string[])
                    n1061 = Build Array(w883, w884, w885) -> (w882:string[])
                    n1062 = Build Array(w878, w817, w816) -> (w877:string[])
                    n1063 = Build Array(w873, w874, w875) -> (w869:string[])
                    n1064 = Build Array(w865, w864, w863) -> (w862:string[])
                    n1065 = Build Array(w859, w860, w861) -> (w855:string[])
                    n1066 = Build Array(w896, w893, w891, w882, w877, w869, w862, w855, w805) -> (w833:string[][])
                    n1067 = local write "右工位报表"(w833) -> ()
                  }
                  frame #2 {
                    n1068 = Wait (ms)(milliseconds to wait=u32 10 ("等待时间（毫秒）")) -> ()  [unwired: 1 out]
                    n1069 = shared-variable "我的电脑\\Global.lvlib\\右工位追溯码"() -> (w903:string)  [unwired: 1 in, 1 out]
                    n1070 = call "Report_A131258-右.vi"("文件重命名"=TRUE, "文件名称"=w903, "布尔数组"="右工位判定结果 4") -> ()  [unwired: 8 in, 1 out]
                  }
                  frame #3 {
                  }
                  frame #4 {
                  }
                  frame #5 {
                    n1071 = shared-variable "我的电脑\\Modbus.lvlib\\右工位状态"(u16 1000 ("左工位状态")) -> ()  [unwired: 1 in, 1 out]
                  }
                }
              }
              frame 3 {
                w913 = FALSE ("合格指示灯")
                w905 = u32 13816530
                w906 = 0
                n1072 = shared-variable "我的电脑\\Modbus.lvlib\\右工位生产结果"(u16 0 ("右工位生产结果")) -> ()  [unwired: 1 in, 1 out]
                n1073 = local write "右工位追溯码"("" ("右工位追溯码")) -> ()
                n1074 = property on="右工位正向最大扭矩(Nm)" class="DigNum (严格)"("NumText.BGColor"=w905) -> ()  [unwired: 2 in, 2 out]
                n1075 = property on="右工位正向波动扭矩(Nm)" class="DigNum (严格)"("NumText.BGColor"=w905) -> ()  [unwired: 2 in, 2 out]
                n1076 = property on="右工位正向平均扭矩(Nm)" class="DigNum (严格)"("NumText.BGColor"=w905) -> ()  [unwired: 2 in, 2 out]
                n1077 = property on="右工位正逆平均扭矩差(Nm)" class="DigNum (严格)"("NumText.BGColor"=w905) -> ()  [unwired: 2 in, 2 out]
                n1078 = property on="右工位逆向最大扭矩(Nm)" class="DigNum (严格)"("NumText.BGColor"=w905) -> ()  [unwired: 2 in, 2 out]
                n1079 = property on="右工位正向最小扭矩(Nm)" class="DigNum (严格)"("NumText.BGColor"=w905) -> ()  [unwired: 2 in, 2 out]
                n1080 = property on="右工位逆向最小扭矩(Nm)" class="DigNum (严格)"("NumText.BGColor"=w905) -> ()  [unwired: 2 in, 2 out]
                n1081 = property on="右工位逆向波动扭矩(Nm)" class="DigNum (严格)"("NumText.BGColor"=w905) -> ()  [unwired: 2 in, 2 out]
                n1082 = property on="右工位逆向平均扭矩(Nm)" class="DigNum (严格)"("NumText.BGColor"=w905) -> ()  [unwired: 2 in, 2 out]
                n1083 = local write "合格指示灯"(w913) -> ()
                n1084 = local write "不合格指示灯"(w913) -> ()
                n1085 = local write "右工位正向最小扭矩(Nm)"(w906) -> ()
                n1086 = local write "右工位正逆平均扭矩差(Nm)"(w906) -> ()
                n1087 = local write "右工位正向平均扭矩(Nm)"(w906) -> ()
                n1088 = local write "右工位正向最大扭矩(Nm)"(w906) -> ()
                n1089 = local write "右工位正向波动扭矩(Nm)"(w906) -> ()
                n1090 = local write "右工位逆向最大扭矩(Nm)"(w906) -> ()
                n1091 = local write "右工位逆向最小扭矩(Nm)"(w906) -> ()
                n1092 = local write "右工位逆向波动扭矩(Nm)"(w906) -> ()
                n1093 = local write "右工位逆向平均扭矩(Nm)"(w906) -> ()
                n1094 = for {
                  N: 4 -> [_]
                  tunnel: [cluster{dbl[], dbl[]} {[], []}] -> w911 mode=indexing
                }
                "力位移曲线 3" <- w911
                n1095 = shared-variable "我的电脑\\Modbus.lvlib\\空载速度"() -> (w909:sgl)  [unwired: 1 in, 1 out]
                n1096 = property on="右工位正逆平均扭矩差(Nm)" class="DigNum (严格)"("NumText.BGColor"=w905) -> ()  [unwired: 2 in, 2 out]
                n1097 = local write "右工位正逆平均扭矩差(Nm)"(w906) -> ()
                n1098 = Multiply(x=w909, y=sgl 6.0) -> (x*y=w908:sgl)
                n1099 = global write "Global.vi" "空载速度(°/s)"(w908) -> ()
              }
              frame 200 {
                n1100 = stacked-sequence {
                  frame #0 {
                    w920 = FALSE ("合格指示灯")
                    w918 = u32 13816530
                    w921 = 0.0 ("正向空载最小扭矩(Nm)")
                    n1101 = shared-variable "我的电脑\\Modbus.lvlib\\右工位生产结果"(u16 0 ("右工位生产结果")) -> ()  [unwired: 1 in, 1 out]
                    n1102 = local write "右工位正向最小扭矩(Nm)"(w921) -> ()
                    n1103 = local write "右工位正向最大扭矩(Nm)"(w921) -> ()
                    n1104 = local write "右工位正向波动扭矩(Nm)"(w921) -> ()
                    n1105 = local write "右工位正向平均扭矩(Nm)"(w921) -> ()
                    n1106 = local write "右工位逆向最小扭矩(Nm)"(w921) -> ()
                    n1107 = local write "右工位逆向最大扭矩(Nm)"(w921) -> ()
                    n1108 = local write "右工位逆向波动扭矩(Nm)"(w921) -> ()
                    n1109 = local write "右工位逆向平均扭矩(Nm)"(w921) -> ()
                    n1110 = local write "合格指示灯"(w920) -> ()
                    n1111 = local write "不合格指示灯"(w920) -> ()
                    n1112 = property on="右工位正向最大扭矩(Nm)" class="DigNum (严格)"("NumText.BGColor"=w918) -> ()  [unwired: 2 in, 2 out]
                    n1113 = property on="右工位逆向平均扭矩(Nm)" class="DigNum (严格)"("NumText.BGColor"=w918) -> ()  [unwired: 2 in, 2 out]
                    n1114 = property on="右工位正向最小扭矩(Nm)" class="DigNum (严格)"("NumText.BGColor"=w918) -> ()  [unwired: 2 in, 2 out]
                    n1115 = property on="右工位正向波动扭矩(Nm)" class="DigNum (严格)"("NumText.BGColor"=w918) -> ()  [unwired: 2 in, 2 out]
                    n1116 = property on="右工位正向平均扭矩(Nm)" class="DigNum (严格)"("NumText.BGColor"=w918) -> ()  [unwired: 2 in, 2 out]
                    n1117 = property on="右工位逆向最小扭矩(Nm)" class="DigNum (严格)"("NumText.BGColor"=w918) -> ()  [unwired: 2 in, 2 out]
                    n1118 = property on="右工位逆向最大扭矩(Nm)" class="DigNum (严格)"("NumText.BGColor"=w918) -> ()  [unwired: 2 in, 2 out]
                    n1119 = property on="右工位逆向波动扭矩(Nm)" class="DigNum (严格)"("NumText.BGColor"=w918) -> ()  [unwired: 2 in, 2 out]
                    n1120 = for {
                      N: 4 -> [_]
                      tunnel: [cluster{dbl[], dbl[]} {[], []}] -> w917 mode=indexing
                    }
                    n1121 = local write "力位移曲线 3"(w917) -> ()
                  }
                  frame #1 {
                    w923 = TRUE ("Initialize 2")
                    n1122 = local write "Initialize 3"(w923) -> ()
                    n1123 = local write "Initialize 5"(w923) -> ()
                    n1124 = local read "力位移曲线 3"() -> (w924:cluster{dbl[], dbl[]}[])
                    n1125 = for {
                      tunnel: [w928] -> w925 mode=indexing
                      tunnel: w924 -> [w927] mode=indexing
                      i -> [w926]
                      n1126 = case shown="0" w926 {
                        tunnel: [w929 w951] -> w928
                        tunnel: w927 -> [w929 _]
                        frame Default {
                        }
                        frame 0 {
                          n1127 = local read "判定框参数"() -> (w942:string[][])
                          n1128 = Index Array(array=w942, index (row) #1=0 ("索引 (行)"), index (row) #2=1 ("索引 (行)"), index (row) #3=2 ("索引 (行)"), index (row) #4=3 ("索引 (行)")) -> (element #1=w950:string[], element #2=w949:string[], element #3=w948:string[], element #4=w947:string[])  [unwired: 4 in]
                          n1129 = Index Array(array=w949, index=1 ("索引")) -> (element=w945:string)
                          n1130 = Index Array(array=w950, index=1 ("索引")) -> (element=w946:string)
                          n1131 = Index Array(array=w947, index=1 ("索引")) -> (element=w943:string)
                          n1132 = Index Array(array=w948, index=1 ("索引")) -> (element=w944:string)
                          n1133 = Fract/Exp String To Number(string=w945) -> (number=w932:dbl)  [unwired: 3 in, 1 out]
                          n1134 = Fract/Exp String To Number(string=w943) -> (number=w930:dbl)  [unwired: 3 in, 1 out]
                          n1135 = Fract/Exp String To Number(string=w946) -> (number=w933:dbl)  [unwired: 3 in, 1 out]
                          n1136 = Fract/Exp String To Number(string=w944) -> (number=w931:dbl)  [unwired: 3 in, 1 out]
                          n1137 = Build Array(w933, w933, w932, w932, w933) -> (w952:dbl[])
                          n1138 = Build Array(w931, w930, w930, w931, w931) -> (w953:dbl[])
                          n1139 = Bundle(w952, w953) -> (w951:cluster{dbl[], dbl[]})  [unwired: 1 in]
                        }
                      }
                    }
                    n1140 = local write "力位移曲线 3"(w925) -> ()
                  }
                  frame #2 {
                    n1141 = local read "力位移曲线 3"() -> (w954:cluster{dbl[], dbl[]}[])
                    n1142 = for {
                      tunnel: [w958] -> w955 mode=indexing
                      tunnel: w954 -> [w957] mode=indexing
                      i -> [w956]
                      n1143 = case shown="1" w956 {
                        tunnel: [w959 w981] -> w958
                        tunnel: w957 -> [w959 _]
                        frame Default {
                        }
                        frame 1 {
                          n1144 = local read "判定框参数"() -> (w972:string[][])
                          n1145 = Index Array(array=w972, index (row) #1=4 ("索引 (行)"), index (row) #2=5 ("索引 (行)"), index (row) #3=6 ("索引 (行)"), index (row) #4=7 ("索引 (行)")) -> (element #1=w980:string[], element #2=w979:string[], element #3=w978:string[], element #4=w977:string[])  [unwired: 4 in]
                          n1146 = Index Array(array=w979, index=1 ("索引")) -> (element=w975:string)
                          n1147 = Index Array(array=w980, index=1 ("索引")) -> (element=w976:string)
                          n1148 = Index Array(array=w978, index=1 ("索引")) -> (element=w974:string)
                          n1149 = Index Array(array=w977, index=1 ("索引")) -> (element=w973:string)
                          n1150 = Fract/Exp String To Number(string=w975) -> (number=w962:dbl)  [unwired: 3 in, 1 out]
                          n1151 = Fract/Exp String To Number(string=w974) -> (number=w961:dbl)  [unwired: 3 in, 1 out]
                          n1152 = Fract/Exp String To Number(string=w976) -> (number=w963:dbl)  [unwired: 3 in, 1 out]
                          n1153 = Fract/Exp String To Number(string=w973) -> (number=w960:dbl)  [unwired: 3 in, 1 out]
                          n1154 = Build Array(w963, w963, w962, w962, w963) -> (w982:dbl[])
                          n1155 = Build Array(w960, w961, w961, w960, w960) -> (w983:dbl[])
                          n1156 = Bundle(w982, w983) -> (w981:cluster{dbl[], dbl[]})  [unwired: 1 in]
                        }
                      }
                    }
                    n1157 = local write "力位移曲线 3"(w955) -> ()
                  }
                }
              }
              frame 1001 {
                n1158 = stacked-sequence {
                  frame #0 {
                    n1159 = local write "字符串"("0" ("字符串")) -> ()
                    n1160 = local read "code 2"() -> (w986:string)
                    n1161 = String Length(string=w986) -> (length=w988:i32)
                    n1162 = Greater Or Equal?(x=w988, y=3) -> (x >= y?=w987:bool)
                    n1163 = case shown="真" w987 {
                      frame False {
                      }
                      frame True {
                        n1164 = shared-variable "我的电脑\\Modbus.lvlib\\右工位状态"(u16 1003 ("左工位状态")) -> ()  [unwired: 1 in, 1 out]
                        n1165 = local read "code 2"() -> (w989:string)
                        n1166 = Concatenate Strings(w989) -> (w991:string)
                        n1167 = local write "右工位追溯码"(w991) -> ()
                        n1168 = shared-variable "我的电脑\\Global.lvlib\\右工位追溯码"(w991) -> ()  [unwired: 1 in, 1 out]
                      }
                    }
                  }
                  frame #1 {
                    n1169 = global read "Global1.vi" "联机模式"() -> (w992:enum16{"单机", "追溯"})
                    n1170 = case shown="\"追溯\"" w992 {
                      selector: w992 -> [_ w994]
                      frame "单机", Default {
                      }
                      frame "追溯" {
                        n1171 = shared-variable "我的电脑\\Global.lvlib\\右工位追溯码"() -> ()  [unwired: 1 in, 2 out]
                        n1172 = local read "右工位追溯码"() -> (w993:string)
                        n1173 = local read "PRODUCTID"() -> (w1002:string)
                        n1174 = Bundle("右工位追溯码"=w993, "PRODUCTID"=w1002) -> (w1000:cluster{"右工位追溯码":string, "PRODUCTID":string})  [unwired: 1 in]
                        n1175 = call "GetSQLstring.vi"("联机模式"=w994) -> ("错误输出"=w997:errorcluster, "连接字符串"=w996:string)  [unwired: 9 in]
                        n1176 = call-poly <vilib>:"DB Tools Open Connection.vi"("error in (no error)"=w997, "connection information"=w996) -> ("error out"=w995:errorcluster, "connection reference"=w998:T15)  [unwired: 6 in]
                        n1177 = Build Array(w1000) -> (w1001:cluster{"右工位追溯码":string, "PRODUCTID":string}[])
                        n1178 = for {
                          tunnel: w1001 -> [w1007] mode=indexing
                          tunnel: w998 -> [w1006]
                          shift-right: [w1004] -> w999
                          shift-left: w995 -> [w1010]
                          w1003 = string[] ["CODE_SENSOR", "PRODUCT_ID"] ("columns")
                          w1008 = "Code" ("table")
                          n1179 = call <vilib>:"DB Tools Insert Data.vi"("data"=w1007, "error in (no error)"=w1010, "columns"=w1003, "table"=w1008, "connection reference"=w1006) -> ("error out"=w1009:errorcluster, "connection reference out"=w1005:T15)  [unwired: 5 in]
                          n1180 = case shown="无错误" w1009 {
                            selector: w1009 -> [w1011 w1014]
                            tunnel: w1003 -> [_ _]
                            tunnel: w1005 -> [w1012 w1015]
                            tunnel: w1008 -> [_ _]
                            tunnel: w1007 -> [_ _]
                            tunnel: [w1012 w1015] -> _
                            tunnel: [w1011 w1013] -> w1004
                            frame No Error {
                            }
                            frame Error {
                              n1181 = call <vilib>:"Clear Errors.vi"("error in (no error)"=w1014) -> ("error out"=w1013:errorcluster)  [unwired: 5 in, 1 out]
                            }
                          }
                        }
                        n1182 = call <vilib>:"Simple Error Handler.vi"("error in (no error)"=w999) -> ()  [unwired: 4 in, 5 out]
                      }
                    }
                  }
                  frame #2 {
                    n1183 = global read "Global1.vi" "联机模式"() -> (w1016:enum16{"单机", "追溯"})
                    n1184 = case shown="\"追溯\"" w1016 {
                      tunnel: w1016 -> [_ w1018]
                      frame "单机", Default {
                      }
                      frame "追溯" {
                        w1020 = "'" ("字符串")
                        n1185 = shared-variable "我的电脑\\Global.lvlib\\右工位追溯码"() -> ()  [unwired: 1 in, 2 out]
                        n1186 = call "GetSQLstring.vi"("联机模式"=w1018) -> ("错误输出"=w1026:errorcluster, "连接字符串"=w1025:string)  [unwired: 9 in]
                        n1187 = local read "右工位追溯码"() -> (w1017:string)
                        n1188 = local read "PRODUCTID"() -> (w1037:string)
                        n1189 = Concatenate Strings("SELECT CODE_ID FROM CODE  WHERE CODE_SENSOR = '" ("table"), w1017, w1020, " AND PRODUCT_ID='" ("字符串"), w1037, w1020) -> (w1027:string)
                        n1190 = call-poly <vilib>:"DB Tools Open Connection.vi"("error in (no error)"=w1026, "connection information"=w1025) -> ("error out"=w1032:errorcluster, "connection reference"=w1031:T15)  [unwired: 6 in]
                        n1191 = call-poly <vilib>:"DB Tools Execute Query.vi"("error in (no error)"=w1032, "SQL query"=w1027, "connection reference"=w1031) -> ("error out"=w1029:errorcluster, "recordset reference"=w1028:T34)  [unwired: 5 in]
                        n1192 = call-poly <vilib>:"DB Tools Fetch Recordset Data.vi"("error in (no error)"=w1029, "recordset reference"=w1028) -> ("error out"=w1033:errorcluster, "recordset data"=w1030:variant[][])  [unwired: 3 in, 1 out]
                        n1193 = Variant To Data(error in=w1033, type=string[][] [], Variant=w1030) -> (data=w1034:string[][])  [unwired: 1 out]
                        n1194 = Index Array(array=w1034, index (row)=0 ("索引 (行)")) -> (element=w1035:string[])  [unwired: 1 in]
                        n1195 = Index Array(array=w1035, index=0 ("索引 (行)")) -> (element=w1036:string)
                        n1196 = local write "RIGHTCODEID"(w1036) -> ()
                      }
                    }
                  }
                }
              }
              frame 1002 {
                n1197 = stacked-sequence {
                  frame #0 {
                    n1198 = local read "code 3"() -> (w1039:string)
                    n1199 = String Length(string=w1039) -> (length=w1041:i32)
                    n1200 = Greater Or Equal?(x=w1041, y=3) -> (x >= y?=w1040:bool)
                    n1201 = case shown="真" w1040 {
                      frame False {
                      }
                      frame True {
                        n1202 = shared-variable "我的电脑\\Modbus.lvlib\\右工位状态"(u16 1003 ("左工位状态")) -> ()  [unwired: 1 in, 1 out]
                        n1203 = local read "code 3"() -> (w1042:string)
                        n1204 = Concatenate Strings(w1042) -> (w1044:string)
                        n1205 = local write "右工位追溯码"(w1044) -> ()
                        n1206 = shared-variable "我的电脑\\Global.lvlib\\右工位追溯码"(w1044) -> ()  [unwired: 1 in, 1 out]
                      }
                    }
                  }
                  frame #1 {
                    n1207 = global read "Global1.vi" "联机模式"() -> (w1045:enum16{"单机", "追溯"})
                    n1208 = case shown="\"追溯\"" w1045 {
                      selector: w1045 -> [_ w1047]
                      frame "单机", Default {
                      }
                      frame "追溯" {
                        n1209 = shared-variable "我的电脑\\Global.lvlib\\右工位追溯码"() -> ()  [unwired: 1 in, 2 out]
                        n1210 = call "GetSQLstring.vi"("联机模式"=w1047) -> ("错误输出"=w1050:errorcluster, "连接字符串"=w1049:string)  [unwired: 9 in]
                        n1211 = local read "右工位追溯码"() -> (w1046:string)
                        n1212 = local read "PRODUCTID"() -> (w1055:string)
                        n1213 = Bundle("右工位追溯码"=w1046, "PRODUCTID"=w1055) -> (w1053:cluster{"右工位追溯码":string, "PRODUCTID":string})  [unwired: 1 in]
                        n1214 = call-poly <vilib>:"DB Tools Open Connection.vi"("error in (no error)"=w1050, "connection information"=w1049) -> ("error out"=w1048:errorcluster, "connection reference"=w1051:T15)  [unwired: 6 in]
                        n1215 = Build Array(w1053) -> (w1054:cluster{"右工位追溯码":string, "PRODUCTID":string}[])
                        n1216 = for {
                          tunnel: w1054 -> [w1060] mode=indexing
                          tunnel: w1051 -> [w1059]
                          shift-right: [w1057] -> w1052
                          shift-left: w1048 -> [w1063]
                          w1056 = string[] ["CODE_SENSOR", "PRODUCT_ID"] ("columns")
                          w1061 = "Code" ("table")
                          n1217 = call <vilib>:"DB Tools Insert Data.vi"("data"=w1060, "error in (no error)"=w1063, "columns"=w1056, "table"=w1061, "connection reference"=w1059) -> ("error out"=w1062:errorcluster, "connection reference out"=w1058:T15)  [unwired: 5 in]
                          n1218 = case shown="错误" w1062 {
                            selector: w1062 -> [w1064 w1067]
                            tunnel: w1056 -> [_ _]
                            tunnel: w1058 -> [w1065 w1068]
                            tunnel: w1061 -> [_ _]
                            tunnel: w1060 -> [_ _]
                            tunnel: [w1065 w1068] -> _
                            tunnel: [w1064 w1066] -> w1057
                            frame No Error {
                            }
                            frame Error {
                              n1219 = call <vilib>:"Clear Errors.vi"("error in (no error)"=w1067) -> ("error out"=w1066:errorcluster)  [unwired: 5 in, 1 out]
                            }
                          }
                        }
                        n1220 = call <vilib>:"Simple Error Handler.vi"("error in (no error)"=w1052) -> ()  [unwired: 4 in, 5 out]
                      }
                    }
                  }
                  frame #2 {
                    n1221 = global read "Global1.vi" "联机模式"() -> (w1069:enum16{"单机", "追溯"})
                    n1222 = case shown="\"追溯\"" w1069 {
                      tunnel: w1069 -> [_ w1071]
                      frame "单机", Default {
                      }
                      frame "追溯" {
                        w1073 = "'" ("字符串")
                        n1223 = shared-variable "我的电脑\\Global.lvlib\\右工位追溯码"() -> ()  [unwired: 1 in, 2 out]
                        n1224 = call "GetSQLstring.vi"("联机模式"=w1071) -> ("错误输出"=w1079:errorcluster, "连接字符串"=w1078:string)  [unwired: 9 in]
                        n1225 = local read "右工位追溯码"() -> (w1070:string)
                        n1226 = local read "PRODUCTID"() -> (w1090:string)
                        n1227 = Concatenate Strings("SELECT CODE_ID FROM CODE  WHERE CODE_SENSOR = '" ("table"), w1070, w1073, " AND PRODUCT_ID='" ("字符串"), w1090, w1073) -> (w1080:string)
                        n1228 = call-poly <vilib>:"DB Tools Open Connection.vi"("error in (no error)"=w1079, "connection information"=w1078) -> ("error out"=w1085:errorcluster, "connection reference"=w1084:T15)  [unwired: 6 in]
                        n1229 = call-poly <vilib>:"DB Tools Execute Query.vi"("error in (no error)"=w1085, "SQL query"=w1080, "connection reference"=w1084) -> ("error out"=w1082:errorcluster, "recordset reference"=w1081:T34)  [unwired: 5 in]
                        n1230 = call-poly <vilib>:"DB Tools Fetch Recordset Data.vi"("error in (no error)"=w1082, "recordset reference"=w1081) -> ("error out"=w1086:errorcluster, "recordset data"=w1083:variant[][])  [unwired: 3 in, 1 out]
                        n1231 = Variant To Data(error in=w1086, type=string[][] [], Variant=w1083) -> (data=w1087:string[][])  [unwired: 1 out]
                        n1232 = Index Array(array=w1087, index (row)=0 ("索引 (行)")) -> (element=w1088:string[])  [unwired: 1 in]
                        n1233 = Index Array(array=w1088, index=0 ("索引 (行)")) -> (element=w1089:string)
                        n1234 = local write "RIGHTCODEID"(w1089) -> ()
                      }
                    }
                  }
                }
              }
            }
          }
          event "系数": Value Change {
            n1235 = event-data() -> ()  [unwired: 1 in, 6 out]
            n1236 = property on="系数 2" class="Tbl (严格)"("Visible"=TRUE ("可见")) -> ()  [unwired: 2 in, 2 out]
          }
          event "删除": Value Change {
            n1237 = event-data() -> ("NewVal"=w1676:bool)  [unwired: 1 in, 5 out]
            n1238 = case shown="真" w1676 {
              tunnel: w1677 -> [_ w1679]
              frame False {
              }
              frame True {
                n1239 = Concatenate Strings("确认删除“", "请选择要删除的产品", "”吗？") -> (w1681:string)
                n1240 = Two Button Dialog(message=w1681) -> (T button?=w1680:bool)  [unwired: 2 in]
                n1241 = case shown="真" w1680 {
                  tunnel: w1679 -> [_ w1685]
                  tunnel: "请选择要删除的产品" -> [_ w1684]
                  frame False {
                  }
                  frame True {
                    n1242 = call <vilib>:"Open Config Data.vi"("configuration file path"=w1685) -> ("error out"=w1687:errorcluster, "refnum"=w1690:T4)  [unwired: 8 in, 1 out]
                    n1243 = call <vilib>:"Remove Section.vi"("section"=w1684, "error in (no error)"=w1687, "refnum"=w1690) -> ("error out"=w1689:errorcluster, "section exists?"=w1686:bool, "refnum out"=w1688:T4)  [unwired: 6 in]
                    n1244 = call <vilib>:"Close Config Data.vi"("error in (no error)"=w1689, "refnum"=w1688) -> ()  [unwired: 8 in, 2 out]
                    n1245 = case shown="假" w1686 {
                      frame False {
                        n1246 = One Button Dialog(message="删除失败！\n请确认产品存在！" ("消息")) -> ()  [unwired: 1 in, 1 out]
                      }
                      frame True {
                        n1247 = One Button Dialog(message="删除成功！" ("消息")) -> ()  [unwired: 1 in, 1 out]
                      }
                    }
                  }
                }
              }
            }
          }
          event "确定": Value Change {
            n1248 = event-data() -> ("NewVal"=w1694:bool)  [unwired: 1 in, 5 out]
            n1249 = Wait Until Next ms Multiple(millisecond multiple=u32 10 ("毫秒倍数")) -> ()  [unwired: 1 out]
            n1250 = case shown="真" w1694 {
              frame False {
              }
              frame True {
                n1251 = stacked-sequence {
                  seq-local: [w1697 _ _ _ _ _ _ _ _] -> [_ _ _ _ _ _ _ _ _]
                  frame #0 {
                    n1252 = local read "产品型号"() -> (w1696:string)
                    "产品型号" <- w1696
                    n1253 = property on="选项卡控件 2" class="TabCtl (严格)"("Value"=enum32{"检测曲线", "参数查看"}."检测曲线" ("选项卡控件 2")) -> ()  [unwired: 2 in, 2 out]
                    n1254 = shared-variable "我的电脑\\Global.lvlib\\产品型号"(w1696) -> ()  [unwired: 1 in, 1 out]
                    n1255 = String Subset(string=w1696, offset (0)=u16 2 ("偏移量(0)"), length (rest)=u16 4 ("长度（剩余）")) -> (substring=w1697:string)
                    n1256 = Decimal String To Number(string=w1697) -> ()  [unwired: 2 in, 2 out]
                  }
                  frame #1 {
                    n1257 = local read "坐标轴参数"() -> (w1709:string[][])
                    n1258 = Index Array(array=w1709, index (row) #1=0 ("索引 (行)"), index (row) #2=1 ("索引 (行)"), index (row) #3=2 ("索引 (行)"), index (row) #4=3 ("索引 (行)"), index (row) #5=4 ("索引 (行)")) -> (element #1=w1721:string[], element #2=w1716:string[], element #3=w1715:string[], element #4=w1714:string[], element #5=w1701:string[])  [unwired: 5 in]
                    n1259 = Index Array(array=w1721, index=1 ("索引")) -> (element=w1713:string)
                    n1260 = Index Array(array=w1716, index=1 ("索引")) -> (element=w1712:string)
                    n1261 = Index Array(array=w1715, index=1 ("索引")) -> (element=w1711:string)
                    n1262 = Index Array(array=w1714, index=1 ("索引")) -> (element=w1710:string)
                    n1263 = Index Array(array=w1701, index=1 ("索引")) -> (element=w1702:string)
                    n1264 = Fract/Exp String To Number(string=w1713) -> (number=w1708:dbl)  [unwired: 3 in, 1 out]
                    n1265 = Fract/Exp String To Number(string=w1712) -> (number=w1707:dbl)  [unwired: 3 in, 1 out]
                    n1266 = Fract/Exp String To Number(string=w1711) -> (number=w1706:dbl)  [unwired: 3 in, 1 out]
                    n1267 = Fract/Exp String To Number(string=w1710) -> (number=w1705:dbl)  [unwired: 3 in, 1 out]
                    n1268 = Fract/Exp String To Number(string=w1702) -> (number=→"系数":dbl)  [unwired: 3 in, 1 out]
                    n1269 = property on="力位移曲线 4" class="XYGraph (严格)"("XScale.Minimum"=w1708) -> ()  [unwired: 2 in, 2 out]
                    n1270 = property on="力位移曲线 4" class="XYGraph (严格)"("XScale.Maximum"=w1707) -> ()  [unwired: 2 in, 2 out]
                    n1271 = property on="力位移曲线 4" class="XYGraph (严格)"("YScale.Minimum"=w1706) -> ()  [unwired: 2 in, 2 out]
                    n1272 = property on="力位移曲线 4" class="XYGraph (严格)"("YScale.Maximum"=w1705) -> ()  [unwired: 2 in, 2 out]
                  }
                  frame #2 {
                    n1273 = local read "坐标轴参数"() -> (w1730:string[][])
                    n1274 = Index Array(array=w1730, index (row) #1=0 ("索引 (行)"), index (row) #2=1 ("索引 (行)"), index (row) #3=2 ("索引 (行)"), index (row) #4=3 ("索引 (行)")) -> (element #1=w1742:string[], element #2=w1737:string[], element #3=w1736:string[], element #4=w1735:string[])  [unwired: 4 in]
                    n1275 = Index Array(array=w1742, index=1 ("索引")) -> (element=w1734:string)
                    n1276 = Index Array(array=w1737, index=1 ("索引")) -> (element=w1733:string)
                    n1277 = Index Array(array=w1736, index=1 ("索引")) -> (element=w1732:string)
                    n1278 = Index Array(array=w1735, index=1 ("索引")) -> (element=w1731:string)
                    n1279 = Fract/Exp String To Number(string=w1734) -> (number=w1729:dbl)  [unwired: 3 in, 1 out]
                    n1280 = Fract/Exp String To Number(string=w1733) -> (number=w1728:dbl)  [unwired: 3 in, 1 out]
                    n1281 = Fract/Exp String To Number(string=w1732) -> (number=w1727:dbl)  [unwired: 3 in, 1 out]
                    n1282 = Fract/Exp String To Number(string=w1731) -> (number=w1726:dbl)  [unwired: 3 in, 1 out]
                    n1283 = property on="力位移曲线 3" class="XYGraph (严格)"("XScale.Minimum"=w1729) -> ()  [unwired: 2 in, 2 out]
                    n1284 = property on="力位移曲线 3" class="XYGraph (严格)"("XScale.Maximum"=w1728) -> ()  [unwired: 2 in, 2 out]
                    n1285 = property on="力位移曲线 3" class="XYGraph (严格)"("YScale.Minimum"=w1727) -> ()  [unwired: 2 in, 2 out]
                    n1286 = property on="力位移曲线 3" class="XYGraph (严格)"("YScale.Maximum"=w1726) -> ()  [unwired: 2 in, 2 out]
                  }
                  frame #3 {
                    n1287 = local read "判定框参数"() -> (w1755:string[][])
                    n1288 = local read "判定框参数"() -> (w1779:string[][])
                    n1289 = local read "力位移曲线 3"() -> (w1756:cluster{dbl[], dbl[]}[])
                    n1290 = local read "力位移曲线 4"() -> (w1792:cluster{dbl[], dbl[]}[])
                    n1291 = Index Array(array=w1755, index (row) #1=0 ("索引 (行)"), index (row) #2=1 ("索引 (行)"), index (row) #3=2 ("索引 (行)"), index (row) #4=3 ("索引 (行)")) -> (element #1=w1769:string[], element #2=w1768:string[], element #3=w1767:string[], element #4=w1766:string[])  [unwired: 4 in]
                    n1292 = Index Array(array=w1779, index (row) #1=0 ("索引 (行)"), index (row) #2=1 ("索引 (行)"), index (row) #3=2 ("索引 (行)"), index (row) #4=3 ("索引 (行)")) -> (element #1=w1787:string[], element #2=w1782:string[], element #3=w1781:string[], element #4=w1780:string[])  [unwired: 4 in]
                    n1293 = Index Array(array=w1768, index=1 ("索引")) -> (element=w1760:string)
                    n1294 = Index Array(array=w1769, index=1 ("索引")) -> (element=w1761:string)
                    n1295 = Index Array(array=w1766, index=1 ("索引")) -> (element=w1758:string)
                    n1296 = Index Array(array=w1767, index=1 ("索引")) -> (element=w1759:string)
                    n1297 = Index Array(array=w1782, index=1 ("索引")) -> (element=w1773:string)
                    n1298 = Index Array(array=w1787, index=1 ("索引")) -> (element=w1774:string)
                    n1299 = Index Array(array=w1780, index=1 ("索引")) -> (element=w1771:string)
                    n1300 = Index Array(array=w1781, index=1 ("索引")) -> (element=w1772:string)
                    n1301 = Fract/Exp String To Number(string=w1760) -> (number=w1764:dbl)  [unwired: 3 in, 1 out]
                    n1302 = Fract/Exp String To Number(string=w1761) -> (number=w1765:dbl)  [unwired: 3 in, 1 out]
                    n1303 = Fract/Exp String To Number(string=w1758) -> (number=w1763:dbl)  [unwired: 3 in, 1 out]
                    n1304 = Fract/Exp String To Number(string=w1759) -> (number=w1762:dbl)  [unwired: 3 in, 1 out]
                    n1305 = Fract/Exp String To Number(string=w1773) -> (number=w1777:dbl)  [unwired: 3 in, 1 out]
                    n1306 = Fract/Exp String To Number(string=w1774) -> (number=w1778:dbl)  [unwired: 3 in, 1 out]
                    n1307 = Fract/Exp String To Number(string=w1771) -> (number=w1776:dbl)  [unwired: 3 in, 1 out]
                    n1308 = Fract/Exp String To Number(string=w1772) -> (number=w1775:dbl)  [unwired: 3 in, 1 out]
                    n1309 = for {
                      tunnel: [w1799] -> w1757 mode=indexing
                      tunnel: w1756 -> [w1798] mode=indexing
                      tunnel: w1765 -> [w1796]
                      tunnel: w1764 -> [w1795]
                      tunnel: w1763 -> [w1794]
                      tunnel: w1762 -> [w1793]
                      i -> [w1797]
                      n1310 = case shown="0" w1797 {
                        tunnel: [w1800 w1805] -> w1799
                        tunnel: w1798 -> [w1800 _]
                        tunnel: w1796 -> [_ w1804]
                        tunnel: w1795 -> [_ w1803]
                        tunnel: w1794 -> [_ w1802]
                        tunnel: w1793 -> [_ w1801]
                        frame Default {
                        }
                        frame 0 {
                          n1311 = Build Array(w1804, w1804, w1803, w1803, w1804) -> (w1806:dbl[])
                          n1312 = Build Array(w1801, w1802, w1802, w1801, w1801) -> (w1807:dbl[])
                          n1313 = Bundle(w1806, w1807) -> (w1805:cluster{dbl[], dbl[]})  [unwired: 1 in]
                        }
                      }
                    }
                    n1314 = for {
                      tunnel: [w1814] -> w1770 mode=indexing
                      tunnel: w1792 -> [w1813] mode=indexing
                      tunnel: w1778 -> [w1811]
                      tunnel: w1777 -> [w1810]
                      tunnel: w1776 -> [w1809]
                      tunnel: w1775 -> [w1808]
                      i -> [w1812]
                      n1315 = case shown="0" w1812 {
                        tunnel: [w1815 w1820] -> w1814
                        tunnel: w1813 -> [w1815 _]
                        tunnel: w1811 -> [_ w1819]
                        tunnel: w1810 -> [_ w1818]
                        tunnel: w1809 -> [_ w1817]
                        tunnel: w1808 -> [_ w1816]
                        frame Default {
                        }
                        frame 0 {
                          n1316 = Build Array(w1819, w1819, w1818, w1818, w1819) -> (w1821:dbl[])
                          n1317 = Build Array(w1816, w1817, w1817, w1816, w1816) -> (w1822:dbl[])
                          n1318 = Bundle(w1821, w1822) -> (w1820:cluster{dbl[], dbl[]})  [unwired: 1 in]
                        }
                      }
                    }
                    n1319 = local write "力位移曲线 3"(w1757) -> ()
                    n1320 = local write "力位移曲线 4"(w1770) -> ()
                  }
                  frame #4 {
                    n1321 = local read "判定框参数"() -> (w1831:string[][])
                    n1322 = local read "判定框参数"() -> (w1863:string[][])
                    n1323 = local read "力位移曲线 3"() -> (w1832:cluster{dbl[], dbl[]}[])
                    n1324 = local read "力位移曲线 4"() -> (w1868:cluster{dbl[], dbl[]}[])
                    n1325 = Index Array(array=w1831, index (row) #1=4 ("索引 (行)"), index (row) #2=5 ("索引 (行)"), index (row) #3=6 ("索引 (行)"), index (row) #4=7 ("索引 (行)")) -> (element #1=w1845:string[], element #2=w1844:string[], element #3=w1843:string[], element #4=w1842:string[])  [unwired: 4 in]
                    n1326 = Index Array(array=w1863, index (row) #1=4 ("索引 (行)"), index (row) #2=5 ("索引 (行)"), index (row) #3=6 ("索引 (行)"), index (row) #4=7 ("索引 (行)")) -> (element #1=w1867:string[], element #2=w1866:string[], element #3=w1865:string[], element #4=w1864:string[])  [unwired: 4 in]
                    n1327 = Index Array(array=w1844, index=1 ("索引")) -> (element=w1836:string)
                    n1328 = Index Array(array=w1845, index=1 ("索引")) -> (element=w1837:string)
                    n1329 = Index Array(array=w1842, index=1 ("索引")) -> (element=w1834:string)
                    n1330 = Index Array(array=w1843, index=1 ("索引")) -> (element=w1835:string)
                    n1331 = Index Array(array=w1866, index=1 ("索引")) -> (element=w1857:string)
                    n1332 = Index Array(array=w1867, index=1 ("索引")) -> (element=w1858:string)
                    n1333 = Index Array(array=w1864, index=1 ("索引")) -> (element=w1855:string)
                    n1334 = Index Array(array=w1865, index=1 ("索引")) -> (element=w1856:string)
                    n1335 = Fract/Exp String To Number(string=w1836) -> (number=w1840:dbl)  [unwired: 3 in, 1 out]
                    n1336 = Fract/Exp String To Number(string=w1837) -> (number=w1841:dbl)  [unwired: 3 in, 1 out]
                    n1337 = Fract/Exp String To Number(string=w1834) -> (number=w1839:dbl)  [unwired: 3 in, 1 out]
                    n1338 = Fract/Exp String To Number(string=w1835) -> (number=w1838:dbl)  [unwired: 3 in, 1 out]
                    n1339 = Fract/Exp String To Number(string=w1857) -> (number=w1861:dbl)  [unwired: 3 in, 1 out]
                    n1340 = Fract/Exp String To Number(string=w1858) -> (number=w1862:dbl)  [unwired: 3 in, 1 out]
                    n1341 = Fract/Exp String To Number(string=w1855) -> (number=w1860:dbl)  [unwired: 3 in, 1 out]
                    n1342 = Fract/Exp String To Number(string=w1856) -> (number=w1859:dbl)  [unwired: 3 in, 1 out]
                    n1343 = for {
                      tunnel: [w1875] -> w1833 mode=indexing
                      tunnel: w1832 -> [w1874] mode=indexing
                      tunnel: w1841 -> [w1872]
                      tunnel: w1840 -> [w1871]
                      tunnel: w1839 -> [w1870]
                      tunnel: w1838 -> [w1869]
                      i -> [w1873]
                      n1344 = case shown="1" w1873 {
                        tunnel: [w1876 w1881] -> w1875
                        tunnel: w1874 -> [w1876 _]
                        tunnel: w1872 -> [_ w1880]
                        tunnel: w1871 -> [_ w1879]
                        tunnel: w1870 -> [_ w1878]
                        tunnel: w1869 -> [_ w1877]
                        frame Default {
                        }
                        frame 1 {
                          n1345 = Build Array(w1880, w1880, w1879, w1879, w1880) -> (w1882:dbl[])
                          n1346 = Build Array(w1877, w1878, w1878, w1877, w1877) -> (w1883:dbl[])
                          n1347 = Bundle(w1882, w1883) -> (w1881:cluster{dbl[], dbl[]})  [unwired: 1 in]
                        }
                      }
                    }
                    n1348 = for {
                      tunnel: [w1890] -> w1854 mode=indexing
                      tunnel: w1868 -> [w1889] mode=indexing
                      tunnel: w1862 -> [w1887]
                      tunnel: w1861 -> [w1886]
                      tunnel: w1860 -> [w1885]
                      tunnel: w1859 -> [w1884]
                      i -> [w1888]
                      n1349 = case shown="1" w1888 {
                        tunnel: [w1891 w1896] -> w1890
                        tunnel: w1889 -> [w1891 _]
                        tunnel: w1887 -> [_ w1895]
                        tunnel: w1886 -> [_ w1894]
                        tunnel: w1885 -> [_ w1893]
                        tunnel: w1884 -> [_ w1892]
                        frame Default {
                        }
                        frame 1 {
                          n1350 = Build Array(w1895, w1895, w1894, w1894, w1895) -> (w1897:dbl[])
                          n1351 = Build Array(w1892, w1893, w1893, w1892, w1892) -> (w1898:dbl[])
                          n1352 = Bundle(w1897, w1898) -> (w1896:cluster{dbl[], dbl[]})  [unwired: 1 in]
                        }
                      }
                    }
                    n1353 = local write "力位移曲线 3"(w1833) -> ()
                    n1354 = local write "力位移曲线 4"(w1854) -> ()
                  }
                  frame #5 {
                    n1355 = local read "结果判定参数"() -> (w1941:string[][])
                    n1356 = Index Array(array=w1941, index (row) #1=0 ("索引 (行)"), index (row) #2=0 ("索引 (行)"), index (row) #3=1 ("索引 (行)"), index (row) #4=1 ("索引 (行)"), index (row) #5=2 ("索引 (行)"), index (row) #6=2 ("索引 (行)"), index (row) #7=3 ("索引 (行)"), index (row) #8=3 ("索引 (行)"), index (row) #9=4 ("索引 (行)"), index (row) #10=4 ("索引 (行)")) -> (element #1=w1949:string[], element #2=w1948:string[], element #3=w1947:string[], element #4=w1946:string[], element #5=w1928:string[], element #6=w1926:string[], element #7=w1912:string[], element #8=w1911:string[], element #9=w1902:string[], element #10=w1901:string[])  [unwired: 10 in]
                    n1357 = Index Array(array=w1949, index=1 ("索引")) -> (element=w1945:string)
                    n1358 = Index Array(array=w1948, index=2 ("索引")) -> (element=w1944:string)
                    n1359 = Index Array(array=w1947, index=1 ("索引")) -> (element=w1943:string)
                    n1360 = Index Array(array=w1946, index=2 ("索引")) -> (element=w1942:string)
                    n1361 = Index Array(array=w1928, index=1 ("索引")) -> (element=w1930:string)
                    n1362 = Index Array(array=w1926, index=2 ("索引")) -> (element=w1929:string)
                    n1363 = Index Array(array=w1912, index=1 ("索引")) -> (element=w1917:string)
                    n1364 = Index Array(array=w1911, index=2 ("索引")) -> (element=w1915:string)
                    n1365 = Index Array(array=w1902, index=1 ("索引")) -> (element=w1904:string)
                    n1366 = Index Array(array=w1901, index=2 ("索引")) -> (element=w1906:string)
                    n1367 = Fract/Exp String To Number(string=w1945) -> (number=→"最大值上限":dbl)  [unwired: 3 in, 1 out]
                    n1368 = Fract/Exp String To Number(string=w1944) -> (number=→"最大值下限":dbl)  [unwired: 3 in, 1 out]
                    n1369 = Fract/Exp String To Number(string=w1943) -> (number=→"波动值上限":dbl)  [unwired: 3 in, 1 out]
                    n1370 = Fract/Exp String To Number(string=w1942) -> (number=→"波动值下限":dbl)  [unwired: 3 in, 1 out]
                    n1371 = Fract/Exp String To Number(string=w1930) -> (number=→"平均值上限":dbl)  [unwired: 3 in, 1 out]
                    n1372 = Fract/Exp String To Number(string=w1929) -> (number=→"平均值下限":dbl)  [unwired: 3 in, 1 out]
                    n1373 = Fract/Exp String To Number(string=w1917) -> (number=→"最小值上限":dbl)  [unwired: 3 in, 1 out]
                    n1374 = Fract/Exp String To Number(string=w1915) -> (number=→"最小值下限":dbl)  [unwired: 3 in, 1 out]
                    n1375 = Fract/Exp String To Number(string=w1904) -> (number=→"平均值差上限":dbl)  [unwired: 3 in, 1 out]
                    n1376 = Fract/Exp String To Number(string=w1906) -> (number=→"平均值差下限":dbl)  [unwired: 3 in, 1 out]
                  }
                  frame #6 {
                    n1377 = Index Array(array="系数 2", index (row) #1=0 ("索引 (行)"), index (row) #2=1 ("索引 (行)"), index (row) #3=2 ("索引 (行)"), index (row) #4=3 ("禁用的索引 (列)"), index (row) #5=4 ("索引 (行)"), index (row) #6=5 ("索引 (行)"), index (row) #7=6 ("索引 (行)")) -> (element #1=w1983:string[], element #2=w1977:string[], element #3=w1976:string[], element #4=w1975:string[], element #5=w1974:string[], element #6=w1973:string[], element #7=w1955:string[])  [unwired: 7 in]
                    n1378 = Index Array(array=w1983) -> (element=w1981:string)  [unwired: 1 in]
                    n1379 = Index Array(array=w1977) -> (element=w1978:string)  [unwired: 1 in]
                    n1380 = Index Array(array=w1976) -> (element=w1972:string)  [unwired: 1 in]
                    n1381 = Index Array(array=w1975) -> (element=w1971:string)  [unwired: 1 in]
                    n1382 = Index Array(array=w1974) -> (element #1=w1970:string, element #2=w1958:string)  [unwired: 2 in]
                    n1383 = Index Array(array=w1973) -> (element #1=w1969:string, element #2=w1956:string)  [unwired: 2 in]
                    n1384 = Index Array(array=w1955) -> (element #1=w1953:string, element #2=w1952:string)  [unwired: 2 in]
                    n1385 = Fract/Exp String To Number(string=w1981) -> (number=→"左平均扭矩系数":dbl)  [unwired: 3 in, 1 out]
                    n1386 = Fract/Exp String To Number(string=w1978) -> (number=→"右平均扭矩系数":dbl)  [unwired: 3 in, 1 out]
                    n1387 = Fract/Exp String To Number(string=w1972) -> (number=→"左扭矩波动":dbl)  [unwired: 3 in, 1 out]
                    n1388 = Fract/Exp String To Number(string=w1971) -> (number=→"右扭矩波动":dbl)  [unwired: 3 in, 1 out]
                    n1389 = Fract/Exp String To Number(string=w1970) -> (number=→"左空载系数":dbl)  [unwired: 3 in, 1 out]
                    n1390 = Fract/Exp String To Number(string=w1958) -> (number=→"左逆向空载":dbl)  [unwired: 3 in, 1 out]
                    n1391 = Fract/Exp String To Number(string=w1969) -> (number=→"右空载系数":dbl)  [unwired: 3 in, 1 out]
                    n1392 = Fract/Exp String To Number(string=w1956) -> (number=→"右逆向空载":dbl)  [unwired: 3 in, 1 out]
                    n1393 = Fract/Exp String To Number(string=w1953) -> (number=w1951:dbl)  [unwired: 3 in, 1 out]
                    n1394 = Fract/Exp String To Number(string=w1952) -> (number=w1950:dbl)  [unwired: 3 in, 1 out]
                    n1395 = global write "Global.vi" "左标定"(w1951) -> ()
                    n1396 = global write "Global.vi" "右标定"(w1950) -> ()
                  }
                  frame #7 {
                    n1397 = global read "Global1.vi" "联机模式"() -> (w1986:enum16{"单机", "追溯"})
                    n1398 = case shown="\"追溯\"" w1986 {
                      tunnel: w1986 -> [_ w2006]
                      frame "单机", Default {
                      }
                      frame "追溯" {
                        n1399 = call "Get_Device_ID.vi"() -> ("Device_ID"=w2008:string)  [unwired: 10 in, 1 out]
                        n1400 = local read "产品型号"() -> (w1987:string)
                        n1401 = local read "用户名"() -> (w1990:string)
                        n1402 = local write "DEVICEID"(w2008) -> ()
                        n1403 = call "GET_PRODUCT_ID.vi"("PRODFUCT_NAME"=w1987) -> ("PRODUCT_ID"=w2007:string)  [unwired: 10 in]
                        n1404 = local write "PRODUCTID"(w2007) -> ()
                        n1405 = call "GetSQLstring.vi"("联机模式"=w2006) -> ("错误输出"=w2004:errorcluster, "连接字符串"=w2005:string)  [unwired: 9 in]
                        n1406 = call-poly <vilib>:"DB Tools Open Connection.vi"("error in (no error)"=w2004, "connection information"=w2005) -> ("error out"=w1997:errorcluster, "connection reference"=w1998:T15)  [unwired: 6 in]
                        n1407 = Concatenate Strings("SELECT USER_ID FROM [User]\n  WHERE USER_NAME = '" ("字符串"), w1990, "'" ("字符串")) -> (w2003:string)
                        n1408 = call-poly <vilib>:"DB Tools Execute Query.vi"("error in (no error)"=w1997, "SQL query"=w2003, "connection reference"=w1998) -> ("error out"=w2001:errorcluster, "recordset reference"=w2002:T34)  [unwired: 5 in]
                        n1409 = call-poly <vilib>:"DB Tools Fetch Recordset Data.vi"("error in (no error)"=w2001, "recordset reference"=w2002) -> ("error out"=w1996:errorcluster, "recordset data"=w2000:variant[][])  [unwired: 3 in, 1 out]
                        n1410 = Variant To Data(error in=w1996, type=string[][] [], Variant=w2000) -> (data=w1995:string[][])  [unwired: 1 out]
                        n1411 = Index Array(array=w1995, index (row)=0 ("索引 (行)")) -> (element=w1993:string[])  [unwired: 1 in]
                        n1412 = Index Array(array=w1993, index=0 ("索引 (行)")) -> (element=w1989:string)
                        n1413 = local write "USERID"(w1989) -> ()
                      }
                    }
                    n1414 = property on="系数 2" class="Tbl (严格)"("Visible"=FALSE ("可见")) -> ()  [unwired: 2 in, 2 out]
                  }
                  frame #8 {
                    w2009 = "参数装载成功！" ("消息")
                    n1415 = call "浮动通知.vi"("通知内容"=w2009) -> ()  [unwired: 11 in]
                    n1416 = One Button Dialog(message=w2009) -> ()  [unwired: 1 in, 1 out]
                  }
                }
              }
            }
          }
          event User Event {
            n1417 = event-data() -> ("StatusChange"=w2011:refnum<class "MGI_MenuItemStatusChange.lvclass">)  [unwired: 1 in, 4 out]
            n1418 = call <userlib>:"BasicInfo.vi"("MGI_MenuItemStatusChange in"=w2011) -> ("Tag"=w2010:string)  [unwired: 7 in, 3 out]
            n1419 = case shown="\"退出\"" w2010 {
              frame "文件", Default {
              }
              frame "传感器标定" {
                n1420 = vi-ref "Setting.vi"() -> (w2013:refnum<vi>)
                n1421 = call "CallVI.vi"("VI引用"=w2013, "状态"=T1."Standard") -> ()  [unwired: 11 in, 3 out]
              }
              frame "退出" {
                n1422 = Quit LabVIEW(quit? (T)=TRUE ("退出？(T)")) -> ()
              }
            }
          }
          event "系数": Mouse Enter {
            n1423 = event-data() -> ()  [unwired: 1 in, 4 out]
            n1424 = property on="系数" class="Bool"("Colors [4]"=cluster{u32, u32}[] [{16777216, 16777216}] ("颜色[4]")) -> ()  [unwired: 2 in, 2 out]
          }
          event "添加": Value Change {
            n1425 = event-data() -> ("NewVal"=w2018:bool)  [unwired: 1 in, 5 out]
            n1426 = local read "请输入添加的产品名称"() -> (w2019:string)
            n1427 = call <vilib>:"Trim Whitespace.vi"("string"=w2019) -> ("trimmed string"=w2020:string)  [unwired: 1 in]
            n1428 = White Space?(1:w2020) -> (0:w2021:bool)
            n1429 = case shown="真" w2021 {
              tunnel: w2016 -> [w2024 _]
              tunnel: w2018 -> [w2023 _]
              tunnel: w2017 -> [w2022 _]
              frame False {
                n1430 = case shown="真" w2023 {
                  tunnel: w2024 -> [_ w2026]
                  tunnel: w2022 -> [_ w2025]
                  frame False {
                  }
                  frame True {
                    n1431 = for {
                      tunnel: w2026 -> [w2029] mode=indexing
                      tunnel: w2025 -> [w2028]
                      n1432 = call "Read_Write ParaINI File.vi"("Mode"=enum16{"Read", "Write"}."Write", "Section"="请输入添加的产品名称", "Filepath"=w2028, "Ctl Refnum"=w2029) -> ()  [unwired: 7 in, 1 out]
                    }
                  }
                }
              }
              frame True {
                w2031 = 64 items=["None"=0, "Hand, Error, Stop"=16, "Question"=32, "Exclamation, Warning"=48, "Asterisk, Information"=64] ("icon")
                w2032 = 0 items=["OK", "OKCancel", "AbortRetryIgnore", "YesNoCancel", "YesNo", "RetryCancel"] ("buttons")
                n1433 = call "信息框（标题、文本、图标）.vi"("icon"=w2031, "buttons"=w2032, "caption"="添加失败", "text"="请输入产品名称!") -> ()  [unwired: 6 in, 2 out]
              }
            }
          }
          event "产品型号": Value Change {
            n1434 = event-data() -> ()  [unwired: 1 in, 6 out]
            n1435 = stacked-sequence {
              tunnel: w2035 -> [_ w2038]
              tunnel: w2036 -> [_ w2037]
              frame #0 {
              }
              frame #1 {
                n1436 = for {
                  tunnel: w2038 -> [w2041] mode=indexing
                  tunnel: w2037 -> [w2040]
                  n1437 = local read "产品型号"() -> (w2039:string)
                  n1438 = call "Read_Write ParaINI File.vi"("Mode"=enum16{"Read", "Write"}."Read", "Section"=w2039, "Filepath"=w2040, "Ctl Refnum"=w2041) -> ()  [unwired: 7 in, 1 out]
                }
              }
            }
          }
          event "退出": Value Change {
            n1439 = event-data() -> ()  [unwired: 1 in, 6 out]
            n1440 = control-ref of="本VI"() -> (w2045:refnum<vi>)
            n1441 = invoke class="VI" method="FP.Close"(reference=w2045) -> (reference out=w2043:refnum<vi>, error out=w2044:errorcluster)  [unwired: 2 in, 1 out]
            n1442 = Close Reference(reference=w2043, error in (no error)=w2044) -> ()  [unwired: 1 out]
          }
          event "更新": Value Change {
            n1443 = event-data() -> ("NewVal"=w2048:bool)  [unwired: 1 in, 5 out]
            n1444 = case shown="真" w2048 {
              tunnel: w2047 -> [_ w2051]
              tunnel: w2046 -> [_ w2050]
              frame False {
              }
              frame True {
                n1445 = for {
                  tunnel: w2051 -> [w2056]
                  tunnel: w2050 -> [w2055] mode=indexing
                  tunnel: [w2054] -> w2049
                  n1446 = local read "产品型号"() -> (w2058:string)
                  n1447 = call "Read_Write ParaINI File.vi"("Mode"=enum16{"Read", "Write"}."Write", "Section"=w2058, "Filepath"=w2056, "Ctl Refnum"=w2055) -> ("error out"=w2054:errorcluster)  [unwired: 7 in]
                }
                n1448 = case shown="无错误" w2049 {
                  frame No Error {
                    n1449 = call "浮动通知.vi"("通知内容"="更新成功！") -> ()  [unwired: 11 in]
                  }
                  frame Error {
                    n1450 = call "浮动通知.vi"("通知内容"="更新失败！") -> ()  [unwired: 11 in]
                  }
                }
              }
            }
          }
          event "请输入添加的产品名称": Value Change {
            n1451 = event-data() -> ("NewVal"=w2059:string)  [unwired: 1 in, 5 out]
            n1452 = control-ref of="产品型号"() -> (w2060:refnum<vi>)
            n1453 = property on="属性节点" class="CmbBox"(reference=w2060) -> ("Strings[]"=w2061:string[])  [unwired: 1 in, 2 out]
            n1454 = for {
              tunnel: w2059 -> [w2062]
              tunnel: w2061 -> [w2063] mode=indexing
              n1455 = Equal?(x=w2062, y=w2063) -> (x = y?=w2064:bool)
              n1456 = case shown="真" w2064 {
                tunnel: w2062 -> [_ w2065]
                frame False {
                }
                frame True {
                  n1457 = stacked-sequence {
                    tunnel: w2065 -> [w2071 _]
                    frame #0 {
                      w2066 = 64 items=["None"=0, "Hand, Error, Stop"=16, "Question"=32, "Exclamation, Warning"=48, "Asterisk, Information"=64] ("icon")
                      w2067 = 0 items=["OK", "OKCancel", "AbortRetryIgnore", "YesNoCancel", "YesNo", "RetryCancel"] ("buttons")
                      n1458 = Concatenate Strings("已经存在产品”" ("text"), w2071, "“\n请勿重复添加！" ("字符串")) -> (w2069:string)
                      n1459 = call "信息框（标题、文本、图标）.vi"("icon"=w2066, "buttons"=w2067, "caption"="产品重复", "text"=w2069) -> ()  [unwired: 6 in, 2 out]
                    }
                    frame #1 {
                      n1460 = local write "请输入添加的产品名称"("" ("请输入添加的产品名称")) -> ()
                    }
                  }
                }
              }
            }
          }
          event Panel Close? {
            n1461 = event-data() -> ()  [unwired: 1 in, 4 out]
            n1462 = control-ref of="本VI"() -> (w2083:refnum<vi>)
            n1463 = vi-ref "client.vi"() -> (w2075:refnum<vi>)
            n1464 = vi-ref "传感器读取.vi"() -> (w2078:refnum<vi>)
            n1465 = global write "Global.vi" "程序关闭"(TRUE ("程序关闭")) -> ()
            n1466 = invoke class="VI" method="FP.Close"(reference=w2075) -> (reference out=w2076:refnum<vi>, error out=w2077:errorcluster)  [unwired: 2 in, 1 out]
            n1467 = invoke class="VI" method="FP.Close"(reference=w2078) -> (reference out=w2079:refnum<vi>, error out=w2080:errorcluster)  [unwired: 2 in, 1 out]
            n1468 = invoke class="VI" method="FP.Close"(reference=w2083) -> (reference out=w2081:refnum<vi>, error out=w2082:errorcluster)  [unwired: 2 in, 1 out]
            n1469 = Close Reference(reference=w2076, error in (no error)=w2077) -> ()  [unwired: 1 out]
            n1470 = Close Reference(reference=w2079, error in (no error)=w2080) -> ()  [unwired: 1 out]
            n1471 = Close Reference(reference=w2081, error in (no error)=w2082) -> ()  [unwired: 1 out]
            n1472 = event-data("Discard?"=TRUE ("放弃？")) -> ()  [unwired: 1 in, 1 out]
          }
          event "设备故障": Value Change {
            n1473 = event-data() -> ()  [unwired: 1 in, 6 out]
            n1474 = global read "Global1.vi" "用户信息"() -> (w2090:T2)
            n1475 = Unbundle By Name(w2090) -> ("用户名"=w2088:string)
            n1476 = Bundle("设备名称"="芯轴分总成磨合台", "用户名"=w2088, "设备状态"="设备状态", "附加信息"="附加信息") -> (w2085:T3)  [unwired: 1 in]
            n1477 = vi-ref "client.vi"() -> (w2092:refnum<vi>)
            n1478 = invoke class="VI" method="Ctrl Val.Set"(reference=w2092, "Control Name"="设备信息" ("控件名"), "Value"=w2085) -> ()  [unwired: 2 in, 5 out]
          }
          event "设备缺料": Value Change {
            n1479 = event-data() -> ()  [unwired: 1 in, 6 out]
            n1480 = global read "Global1.vi" "用户信息"() -> (w2098:T2)
            n1481 = Unbundle By Name(w2098) -> ("用户名"=w2096:string)
            n1482 = Bundle("设备名称"="芯轴分总成磨合台", "用户名"=w2096, "设备状态 2"="设备状态 2", "附加信息 2"="附加信息 2") -> (w2093:T35)  [unwired: 1 in]
            n1483 = vi-ref "client.vi"() -> (w2100:refnum<vi>)
            n1484 = invoke class="VI" method="Ctrl Val.Set"(reference=w2100, "Control Name"="设备信息" ("控件名"), "Value"=w2093) -> ()  [unwired: 2 in, 5 out]
          }
          event "质量报警": Value Change {
            n1485 = event-data() -> ()  [unwired: 1 in, 6 out]
            n1486 = global read "Global1.vi" "用户信息"() -> (w2106:T2)
            n1487 = Unbundle By Name(w2106) -> ("用户名"=w2104:string)
            n1488 = Bundle("设备名称"="芯轴分总成磨合台", "用户名"=w2104, "设备状态 3"="设备状态 3", "附加信息 3"="附加信息 3") -> (w2101:T36)  [unwired: 1 in]
            n1489 = vi-ref "client.vi"() -> (w2108:refnum<vi>)
            n1490 = invoke class="VI" method="Ctrl Val.Set"(reference=w2108, "Control Name"="设备信息" ("控件名"), "Value"=w2101) -> ()  [unwired: 2 in, 5 out]
          }
          event "确定按钮": Value Change {
            n1491 = event-data() -> ()  [unwired: 1 in, 6 out]
            n1492 = vi-ref "User_manager.vi"() -> (w2110:refnum<vi>)
            n1493 = call "CallVI.vi"("VI引用"=w2110, "状态"=T1."Maximized") -> ()  [unwired: 11 in, 3 out]
          }
        }
        n1494 = global read "Global.vi" "程序关闭"() -> (w199:bool)
      }
    }
  }
